vi "myRIO_BRig_RT_v0,31.vi"() -> ()   [LabVIEW 2014]
uses:
  <vilib>/Platform/TimedLoop/XDataNode/XDataNode.xnode
  <vilib>/Platform/TimedLoop/XDataNode/nitl_modes.ctl
  <vilib>/Platform/TimedLoop/XDataNode/XDNodeRunTimeDep.lvlib
  <vilib>/Platform/TimedLoop/XDataNode/wakeup.ctl
  <vilib>/Platform/TimedLoop/XDataNode/timing_clust.ctl
  <vilib>/rvi/interface/nirviReadWriteControl/nirviReadWriteControl.xnode
  <vilib>/rvi/interface/Simulation/niFpgaSimulationCallBeginRW.vi
  <vilib>/rvi/errors/niLvFpgaAdjustHostInterfaceError.vi
  <vilib>/rvi/interface/nirviCloseFPGA/nirviCloseFPGA.xnode
  <vilib>/myRIO/Instrument Drivers/Utilities/Utilities.lvlib
  <vilib>/rvi/interface/nirviOpenFPGA/nirviOpenFPGA.xnode
  myRIO_BRig_RT__Case_Exp_stateList.ctl
  <vilib>/WebDAVClient/Advanced/SessionHandle.ctl
  <vilib>/WebDAVClient/NI_WebDAV.lvlib
  myRIO_BRig_RT__Case_NonExp_stateList.ctl
  NiFpgaLv.dll
  <vilib>/Utility/error.llb/Error Cluster From Error Code.vi
  <vilib>/FPGAPlugInAG/Dynamic/niLvFpga_Close_Dynamic.vi
  myRIO_BRig_FPGA_v2,5__PortC__build.lvbitx
  myRIO_BRig_FPGA_v2,5__PortC.vi
  <vilib>/FPGAPlugInAG/myRIO-1900/niLvFpga_Open_myRIO-1900.vi
  <vilib>/rvi/interface/common/dynamic/niFpgaDynamicAddResources.vi
panel:
  in  "LC_Cue1_delayOpt":bool
  in  "LC_ENL1_delayOpt":bool
  in  "Tcycle_Cue_max":u16=1000 caption="Max [ms]" min=5 max=5000 step=5
  in  "Tcycle_Cue_min":u16=1000 caption="Min [ms]" min=5 max=5000 step=5
  in  "SendData":bool
  out "cSpout":enum16{"Left", "Right"}(ring) caption="Left or Right Spout"
  out "A4":u32 caption="LickCounter_Right"
  out "A2":u32 caption="LickCounter_Left"
  in  "tDelay_laser_wro":u32
  in  "tCycle_laser_wro":u32=1000
  in  "tDelay_laser_rew":u32
  in  "laserResponse_wrong_LED":bool
  out "error_initTrial":errorcluster
  out "error_Selection_pre":errorcluster
  out "error_Selection":errorcluster
  in  "tCycle_laser_rew":u32=1000
  out "SelectWrong":bool
  out "SelectReward":bool
  in  "Left(F)_or_Right(T)":bool
  in  "ignoreWrong":bool
  in  "SelectionState":bool
  in  "laserResponse_wrong":bool
  in  "laserResponse_reward":bool
  in  "laserResponse_reward_LED":bool
  out "nRewards_Right":u16 caption="# Rewards Total (Right)"
  out "nRewards_Left":u16 caption="# Rewards Total (Left)"
  out "nRewards_cur":u16 caption="# Rewards in Current Block"
  out "TpB_target":u16 caption="Target Trials Per Block"
  out "cState_NonExp":T1 caption="NonExperimental State"
  out "iBlock":u16 caption="Current Block"
  out "cState":T2 caption="Experimental State"
  out "iTrial":u16 caption="Current Trial"
  in  "warmupType":bool
  in  "TestConnection":bool
  in  "warmup":bool caption="WarmUp"
  in  "Host Filename Prefix":string="Exp1_TM2"
  out "Connected To Host?":bool
  in  "Host Password":string="sabalab"
  in  "Host UserName":string="Test2"
  in  "sp_RightSpout":u16(slide)=2 max=2 step=1 scale=0.0..2.0
  in  "sp_LeftSpout":u16(slide)=2 max=2 step=1 scale=0.0..2.0
  in  "BUR_max":u16 caption="Count Reward Structure  (0 = off)"
  in  "LC_Wrong_Probability":u16
  in  "LC_Wrong_Trial":u16(slide) max=2 step=1 scale=0.0..2.0
  in  "LC_Wrong_Block":u16(slide) max=2 step=1 scale=0.0..2.0
  in  "LC_Wrong_OnOff":bool
  in  "LC_Reward_Probability":u16
  in  "LC_Reward_Trial":u16(slide) max=2 step=1 scale=0.0..2.0
  in  "LC_Reward_Block":u16(slide) max=2 step=1 scale=0.0..2.0
  in  "LC_Reward_OnOff":bool
  in  "LC_Cue2_Probability":u16
  in  "LC_Cue2_Trial":u16(slide) max=2 step=1 scale=0.0..1.0
  in  "LC_Cue2_Block":u16(slide) max=2 step=1 scale=0.0..2.0
  in  "LC_Cue2_OnOff":bool
  in  "LC_Cue1_Probability":u16
  in  "LC_Cue1_Trial":u16(slide) max=2 step=1 scale=0.0..1.0
  in  "LC_Cue1_Block":u16(slide) max=2 step=1 scale=0.0..2.0
  in  "LC_Cue1_OnOff":bool
  in  "LC_ENL2_Probability":u16
  in  "LC_ENL2_Trial":u16(slide) max=2 step=1 scale=0.0..1.0
  in  "LC_ENL2_Block":u16(slide) max=2 step=1 scale=0.0..2.0
  in  "LC_ENL2_OnOff":bool
  in  "LC_ENL1_Probability":u16
  in  "LC_ENL1_Trial":u16(slide) max=2 step=1 scale=0.0..1.0
  in  "LC_ENL1_Block":u16(slide) max=2 step=1 scale=0.0..2.0
  in  "A6":bool caption="Activate Recording?\n(Select Prior to\nStarting Experiment)"
  in  "Tcycle_Timeout":u16=1000 caption="Timeout Time [ms]" min=10 max=10000 step=1
  in  "Tcycle_Wrong":u16=1000 caption="Wrong Time [ms]" min=10 max=10000 step=1
  in  "Tcycle_Selection":u16=1000 caption="Answer Time [ms]" min=1 max=10000 step=1
  in  "Tcycle_RewardPost":u16=1000 caption="Consumption Time [ms]" min=250 max=10000 step=250
  in  "Tcycle_Reward_L":u16=500 caption="Reward Time [ms]" min=1 max=1000 step=1
  in  "Tcycle_Reward_R":u16=500 caption="Reward Time [ms]" min=1 max=1000 step=1
  in  "TpB_Max_R":u16=4 caption="Max TrialsPerBlock" min=1 max=12 step=1
  in  "TpB_Min_R":u16=4 caption="Min TrialsPerBlock" min=1 max=12 step=1
  in  "TpB_Max_L":u16=4 caption="Max TrialsPerBlock" min=1 max=12 step=1
  in  "TpB_Min_L":u16=4 caption="Min TrialsPerBlock" min=1 max=12 step=1
  in  "BUR_min":u16 caption="Count Reward Structure  (0 = off)"
  in  "TrialUntilReward":bool caption="Ignore Wrong \nSelection"
  in  "CueCycles":u16=1 caption="Cue Structure" min=1 max=1 step=1
  in  "MTrig_Laser_Tcycle":u16=10 caption="Time [ms]"
  in  "MTrig_Laser_trig":bool
  in  "MTrig_Audio_trig__R":bool caption="Trigger Audio"
  in  "MTrig_Audio_trig__L":bool caption="Trigger Audio"
  in  "RewCalib_Trig_R":bool caption="Calibrate_R"
  in  "RewCalib_Trig_L":bool caption="Calibrate_L"
  in  "MTrig_Solenoid_Tcycle__R":u16=300 caption="Time [ms]"
  in  "MTrig_Solenoid_Tcycle__L":u16=300 caption="Time [ms]"
  in  "MTrig_Solenoid_trig__R":bool caption="Solenoid"
  in  "MTrig_Solenoid_trig__L":bool caption="Solenoid"
  in  "STOP_abort":bool caption="Stop LabView\n(Stops myRio and FPGA)"
  in  "STOP_endBlock":bool caption="Stop Experiment\n@ End of Block"
  in  "STOP_endTrial":bool caption="Stop Experiment\n@ End of Trial"
  in  "START":bool caption="Start Experiment"
  in  "Tcycle_CuePenalty":u16=1000 caption="Penalty [ms]" min=1 max=10000 step=1
  in  "Audio_Amp__R":u16=100 caption="Amp"
  in  "Audio_Freq__R":u16=5 caption="Freq [kHz]" max=14 step=1
  in  "Audio_Amp__L":u16=100 caption="Amp"
  in  "Audio_Freq__L":u16=5 caption="Freq [kHz]" max=14 step=1
  in  "LC_Wrong_Tdelay":u16
  in  "LC_Cue2_Tdelay":u16
  in  "LC_ENL2_Tdelay":u16
  in  "LC_Reward_Tdelay":u16
  in  "LC_Cue1_Tdelay":u16
  in  "LC_ENL1_Tdelay":u16
  in  "LC_ENL1_OnOff":bool
  in  "Tcycle_ENLPenalty":u16=100 caption="Penalty [ms]" min=10 max=100 step=10
  in  "Tcycle_ENL_max":u16=1000 caption="Max [ms]" min=250 max=10000 step=250
  in  "Tcycle_ENL_min":u16=1000 caption="Min [ms]" min=250 max=10000 step=250
  # "Manual Control"
  # "Task Structure"
  # "Task Timing"
  # "Laser Control    [10ms pulse]\n\n                              On/Off      Block          Trial    Probability [%]   Delay [ms]"
  # "Manual Solenoid Trigger\nLeft              Right"
  # "Master Structure"
  # "Enforced NonLick"
  # "Enforced NonLick 1"
  # "from end"
  # "Time = Cue Min"
  # "Min\n \n  \nMax"
  # "from start"
  # "(1) = Switching\n(2) = Two Choice"
  # "Enforced NonLick 2"
  # "Cue"
  # "Cue 1"
  # "from end"
  # "from start"
  # "Cue then reward"
  # "Min"
  # "Max"
  # "Cue 2"
  # "Cue with reward"
  # "Trial Per Block Structure\n       Left                    Right"
  # "Spout Selection Control"
  # "Manual Speaker Trigger\nLeft              Right"
  # "Selection Reward"
  # "Answer Time\n         [ms]\n\n  \nWrong Choice Penalty\n         [ms]\n \n \nChoice Timeout Penalty\n         [ms]"
  # "Selection Wrong"
  # "Cue Control"
  # "Left              Right"
  # "State"
  # "Manual Laser Trigger"
  # "Freq [kHz]\n \n \nAmp\n \n\n \n\nSpeaker\nSetting"
  # "Reward Control\n                 Left              Right"
  # "Min = 1\nMax = 32k"
  # "Reward Time\n         [ms]"
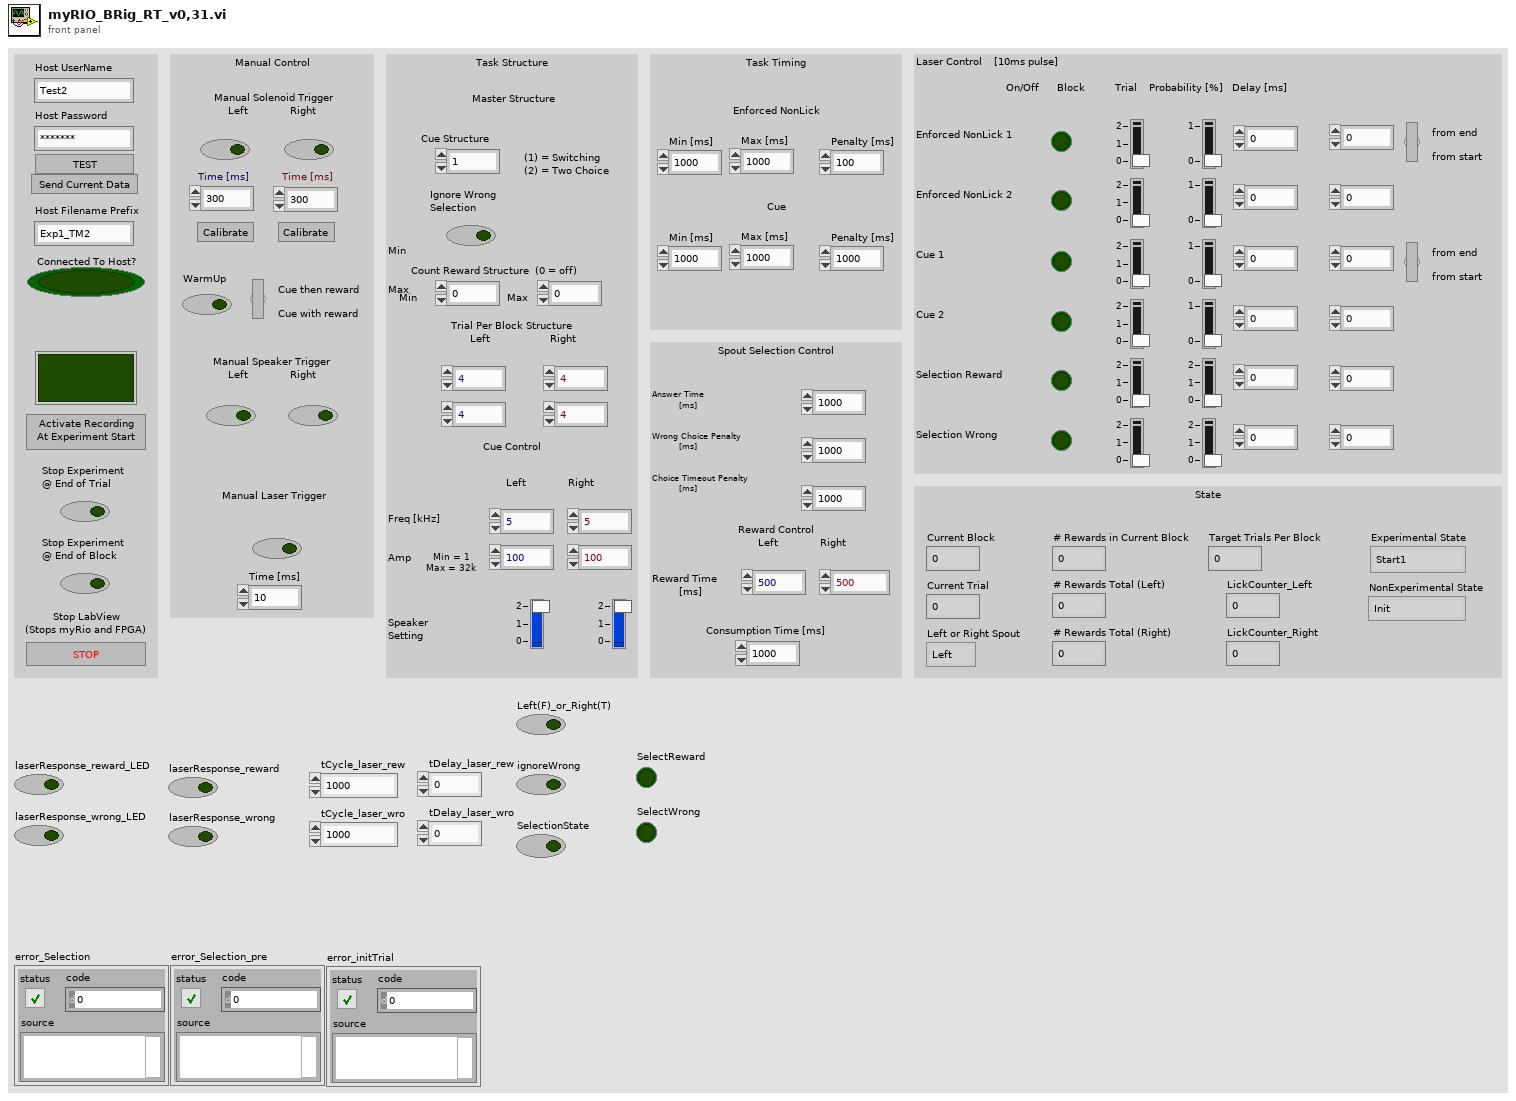
[diagram p1: front panel]
types:
  T1 = typedef "myRIO_BRig_RT__Case_NonExp_stateList.ctl" = enum16{"Init", "UploadSettings_pre", "UploadSettings_Read_dataExp", "UploadSettings_dataExp_1", "UploadSettings_Read_dataLC", "UploadSettings_dataLC_1", "UploadSettings_dataLC_2", "UploadSettings_Read_dataMTrig", "UploadSettings_dataMTrig_1", "UploadSettings_post", "Idle_pre", "IdleEmpty", "IdleEmpty2", "IdleEmpty3", "IdleEmpty4", "Idle", "Idle_2", "Idle_3", "Idle_4", "Idle_post", "Cue_pre__pre", "Cue_pre", "Cue", "Cue_post", "RewardCalibration_pre", "DispenseWater_pre__pre", "DispenseWater_pre", "DispenseWater", "DispenseWater_post", "TestConnection", "SendData", "End"}
  T2 = typedef "myRIO_BRig_RT__Case_Exp_stateList.ctl" = enum16{"Start1", "Start2", "Start3", "saveSettings1", "saveSettings2", "saveSettings3", "saveSettings4_LC_ENL", "saveSettings5_LC_Cue", "saveSettings6_LC_Other", "setSettings_Audio", "setSettings_Laser", "initBlock_pre", "initBlock", "initBlock2", "initBlock_post", "initTrial_pre", "initTrial", "initTrial2", "initTrial3", "initTrial4", "initTrial_LC_ENL1", "initTrial_LC_Cue1", "initTrial_post", "ENL1_pre", "ENL1", "ENL1_post", "ENL1Penalty_pre", "ENL1Penalty", "ENL2_pre", "ENL2", "ENL2Penalty_pre", "ENL2Penalty", "Cue1_pre", "Cue1", "Cue1_post", "Cue1Penalty_pre", "Cue1Penalty", "Cue2_pre", "Cue2", "Cue2Penalty_pre", "Cue2Penalty", "Selection_pre", "Selection", "Select_post", "SelectReward_pre", "SelectReward", "SelectRewardPost_pre", "SelectRewardPost", "SelectWrong_pre", "SelectWrong", "SelectWrong_post", "SelectTimeout_pre", "SelectTimeout", "SelectTimeout_post", "endTrial_pre", "endTrial1", "endTrial2", "endTrial3", "endTrial_post", "endBlock_pre", "endBlock", "endBlock_post", "endExp", "commConnect", "commUpload_pre", "commUpload_dataBlock", "commUpload_dataCurrent", "commUpload_dataExp", "commUpload_dataLC", "commUpload_dataTrial", "commUpload_post", "saveData_pre", "saveData_dataBlock", "saveData_dataCurrent", "saveData_dataExp", "saveData_dataLC", "saveData_dataTrial", "saveData_post"}
  T3 = typedef "XDNodeRunTimeDep.lvlib/timing_clust.ctl" = cluster{"Expected End [f-1]":u64, "Actual End [f-1]":u64, "Finished Late? [f-1]":bool, "Expected End [i-1]":u64, "Actual End [i-1]":u64, "Finished Late? [i-1]":bool, "Expected Start [i]":u64, "Actual Start [i]":u64, "Expected Start [f]":u64, "Actual Start [f]":u64, "Source Name":string, "Structure Name":string, "Period":i64, "Deadline":i64, "Offset":i64, "Start":i64, "Priority":i32, "Timeout":i32, "Mode":T4, "Wakeup Reason":T5, "Error":errorcluster, "Source Type":string, "Secondary Source Type":string, "Global End Time":u64, "Global Start Time":u64, "Frame Duration":u64, "Iteration Duration":u64, "Assigned CPU":i32, "I/O Scan Engine Mode":u32}
  T4 = typedef "XDNodeRunTimeDep.lvlib/nitl_modes.ctl" = enum32{"No Change", "Process missed periods, maintain original phase", "Discard missed periods, maintain original phase", "Process missed periods, ignore original phase", "Discard missed periods, ignore original phase"}
  T5 = typedef "XDNodeRunTimeDep.lvlib/wakeup.ctl" = enum32{"Normal", "Aborted", "Asynchronous wakeup", "Timing source error", "Timed loop error", "Timeout"}
  T6 = typedef "NI_WebDAV.lvlib/SessionHandle.ctl" = refnum<k1>
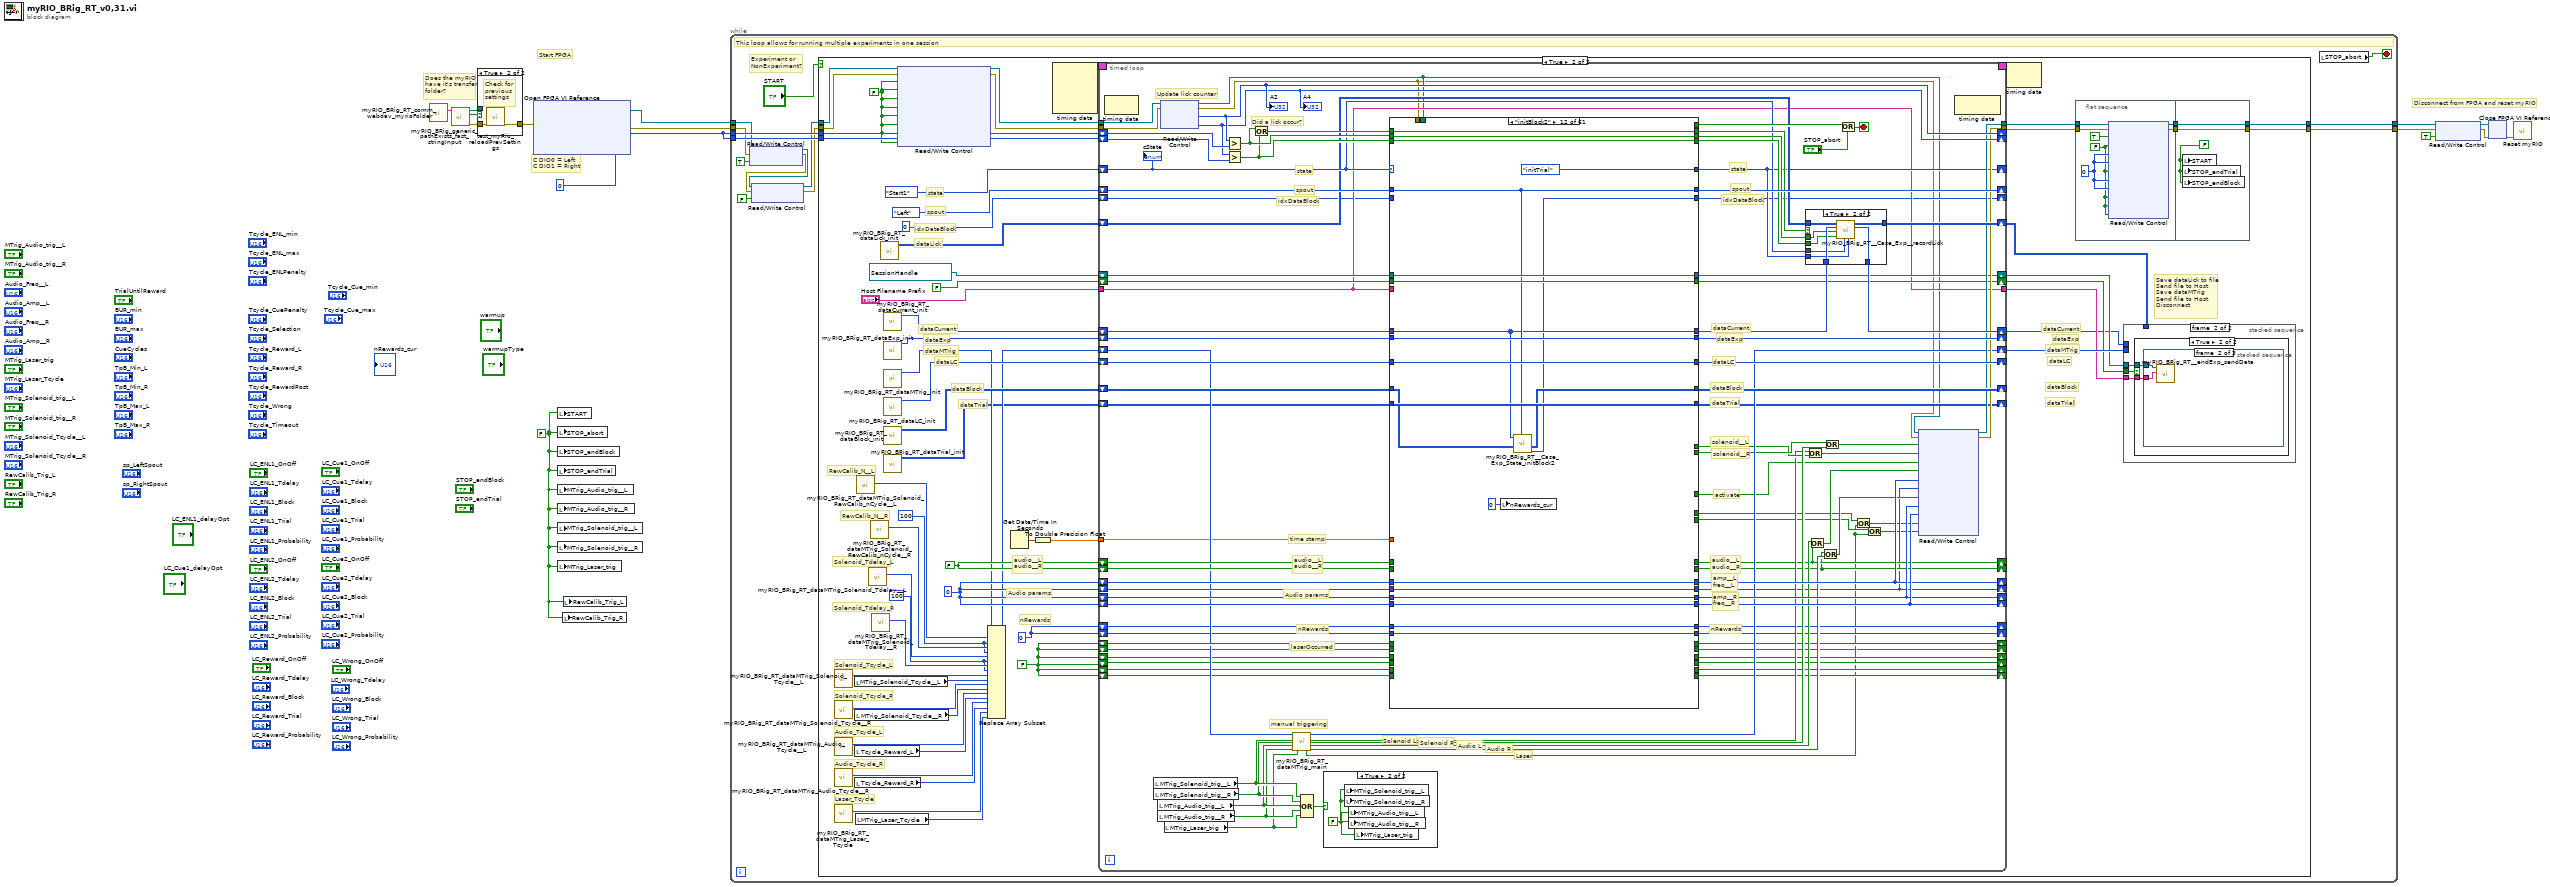
[diagram p0: block diagram]
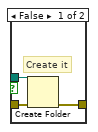
[diagram p2: hidden frame]
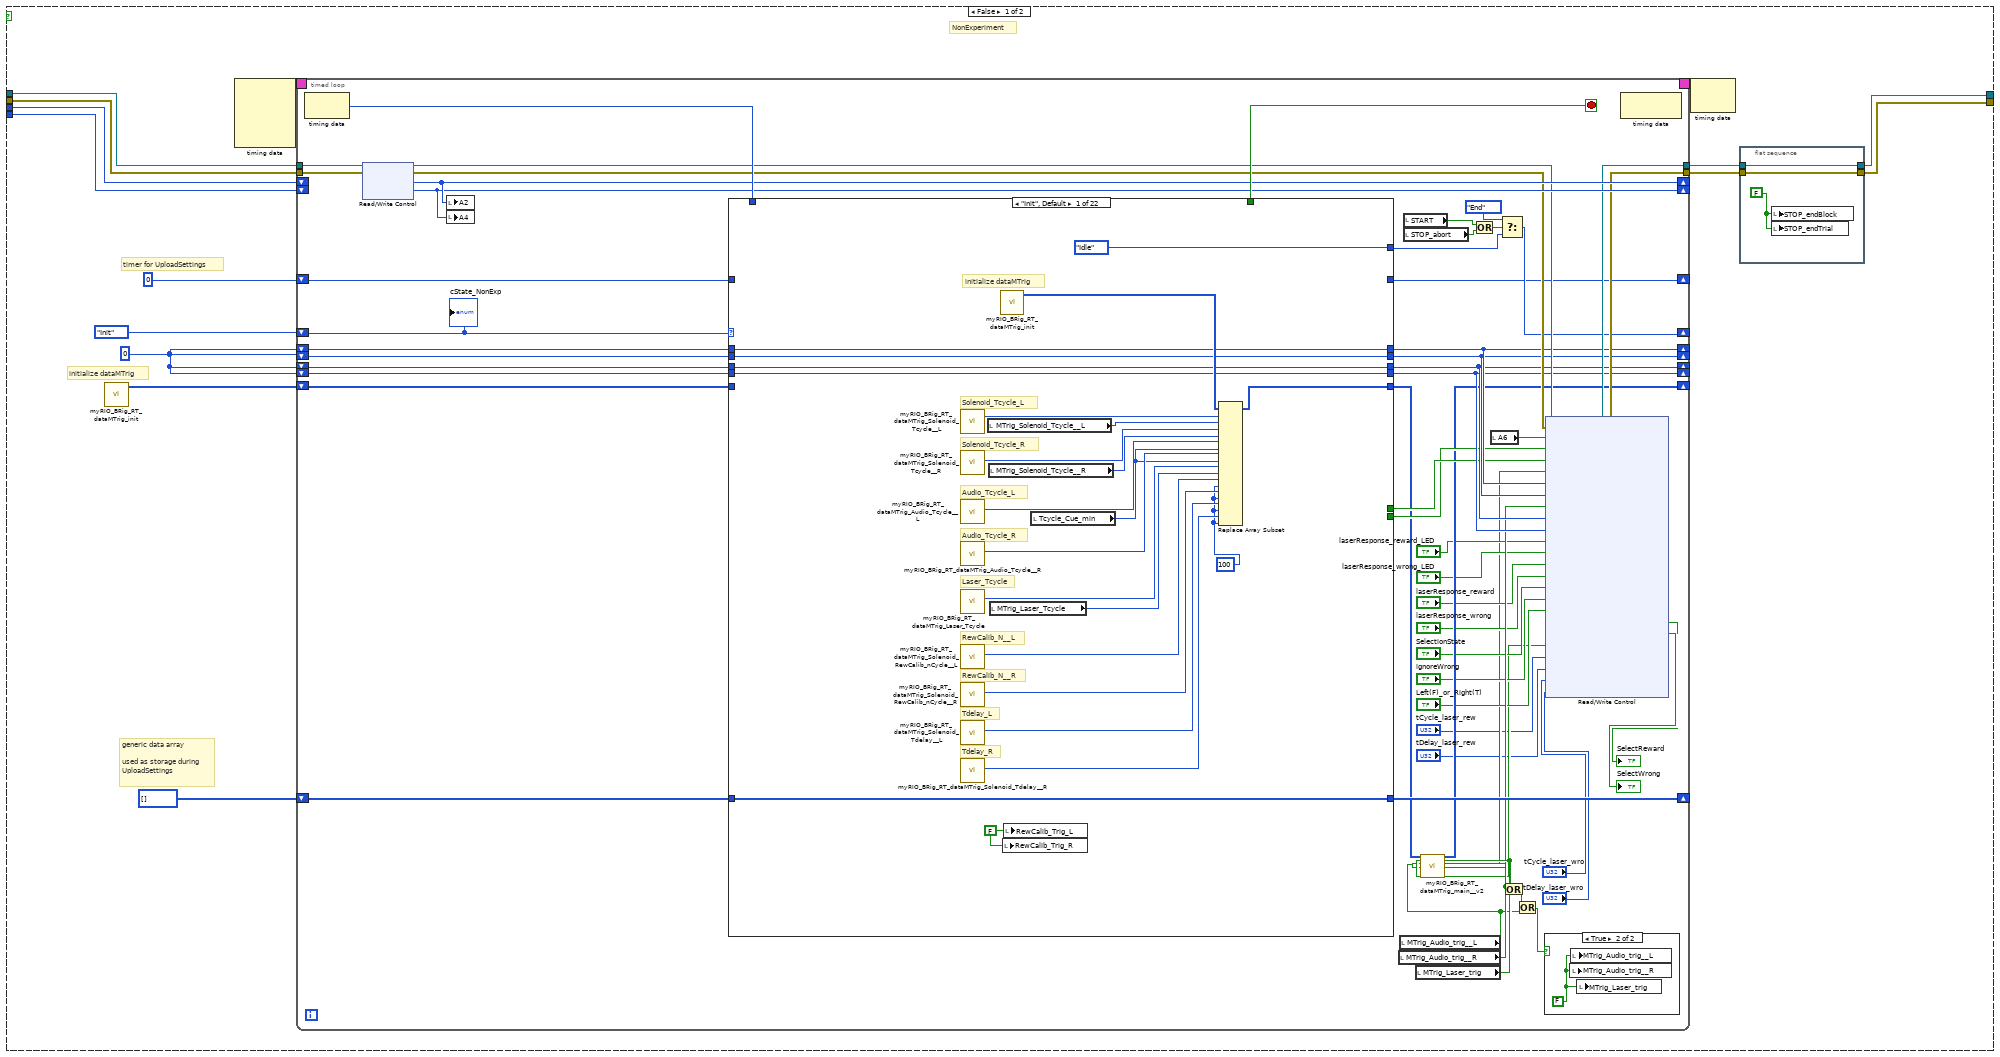
[diagram p3: hidden frame]
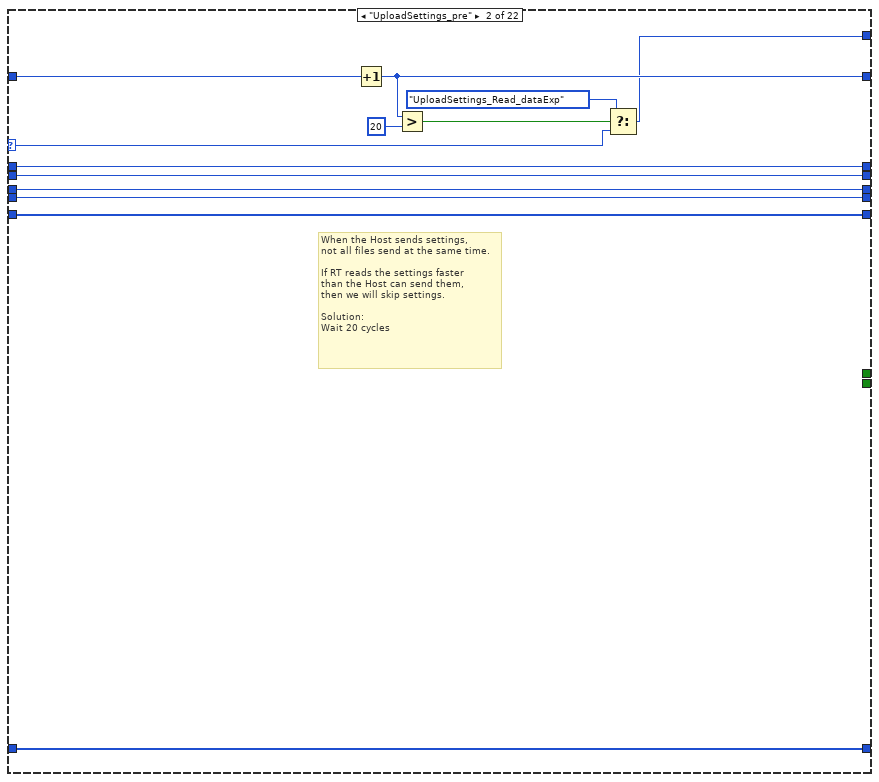
[diagram p5: hidden frame]
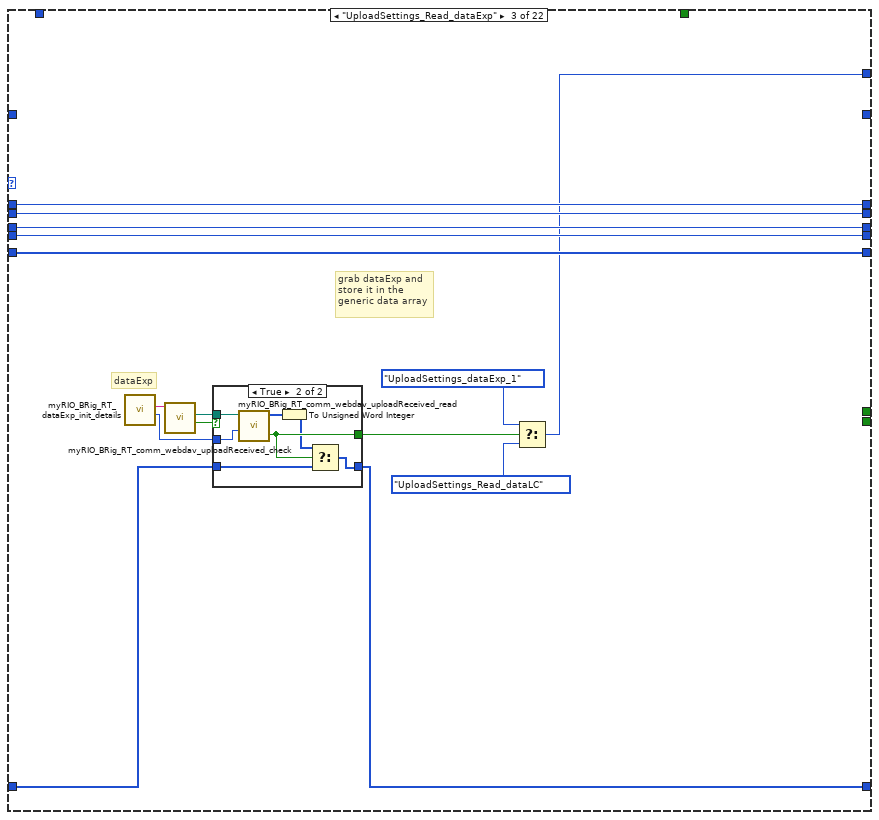
[diagram p6: hidden frame]
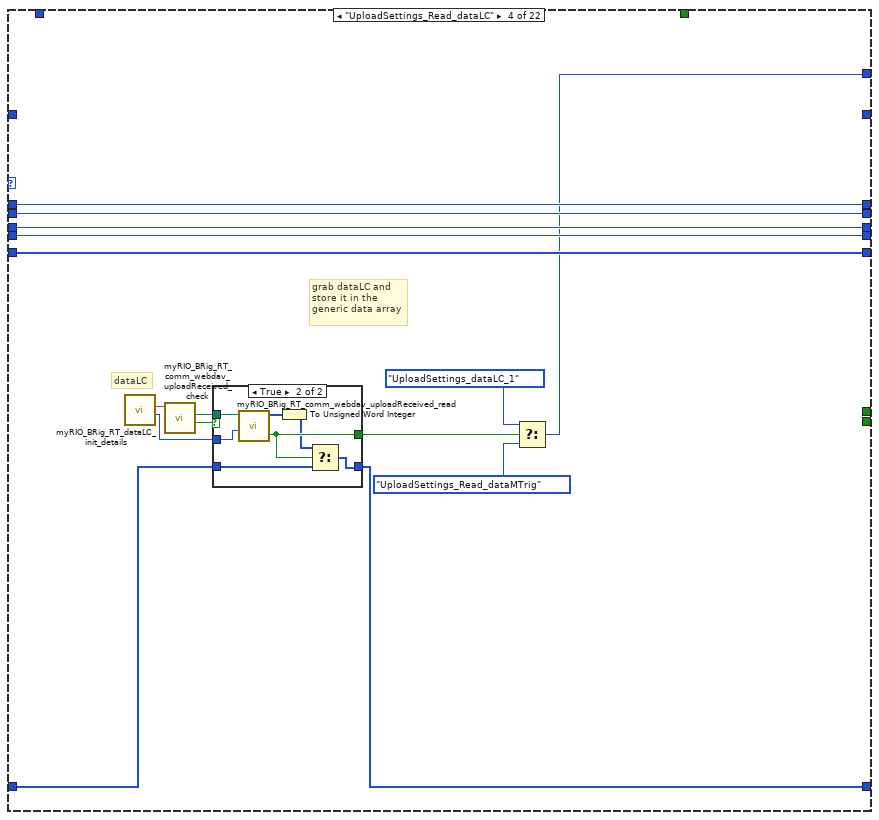
[diagram p8: hidden frame]
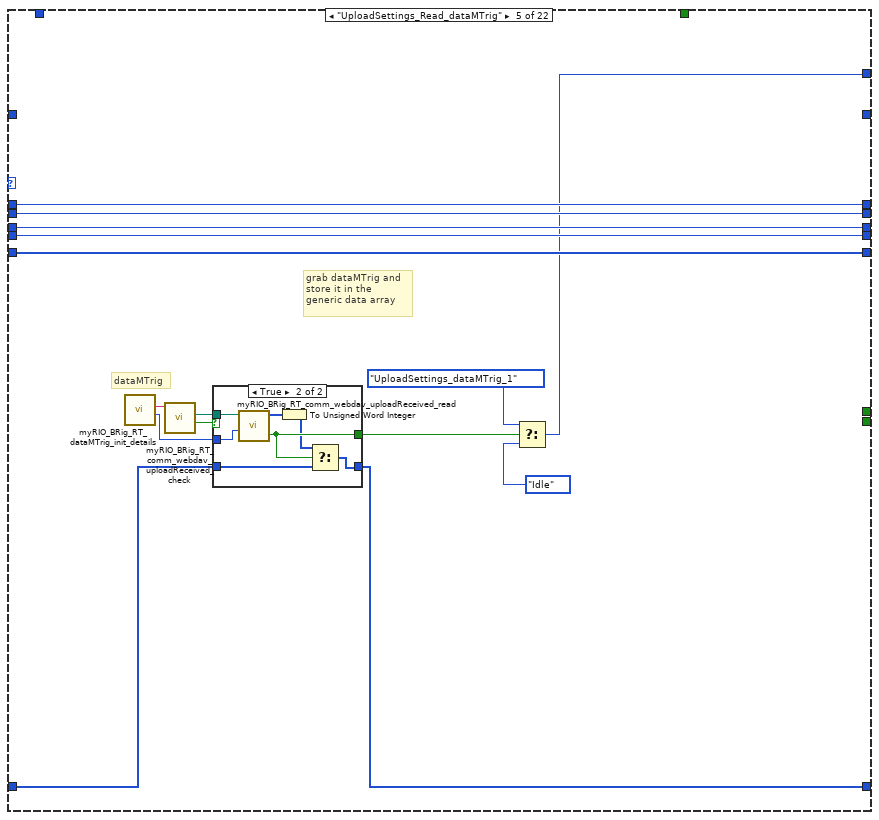
[diagram p10: hidden frame]
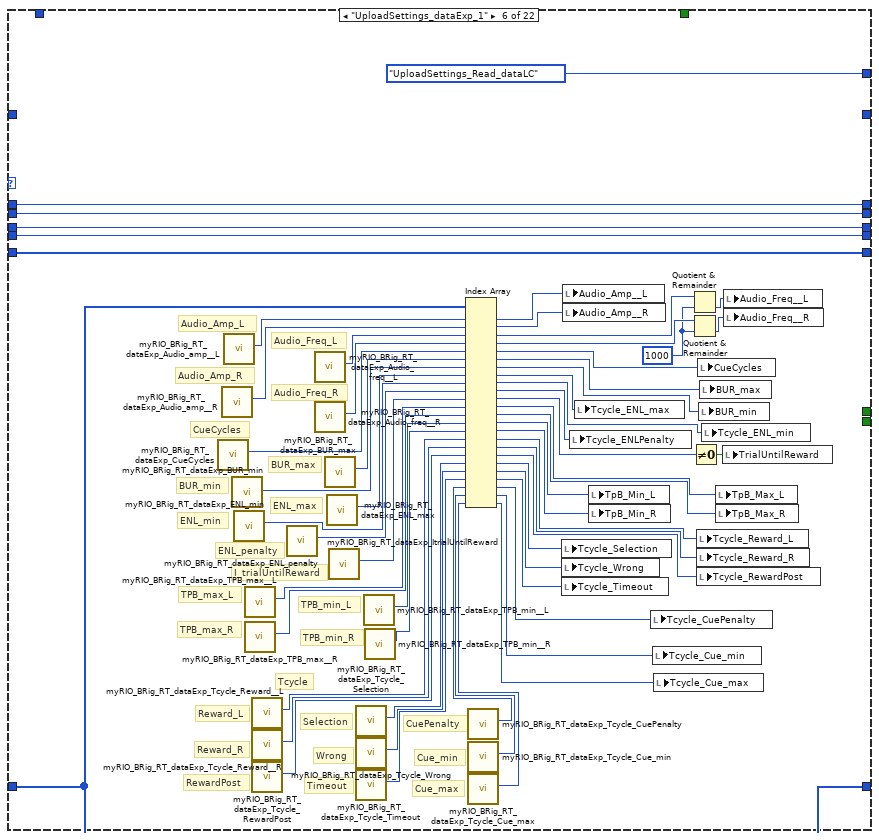
[diagram p12: hidden frame]
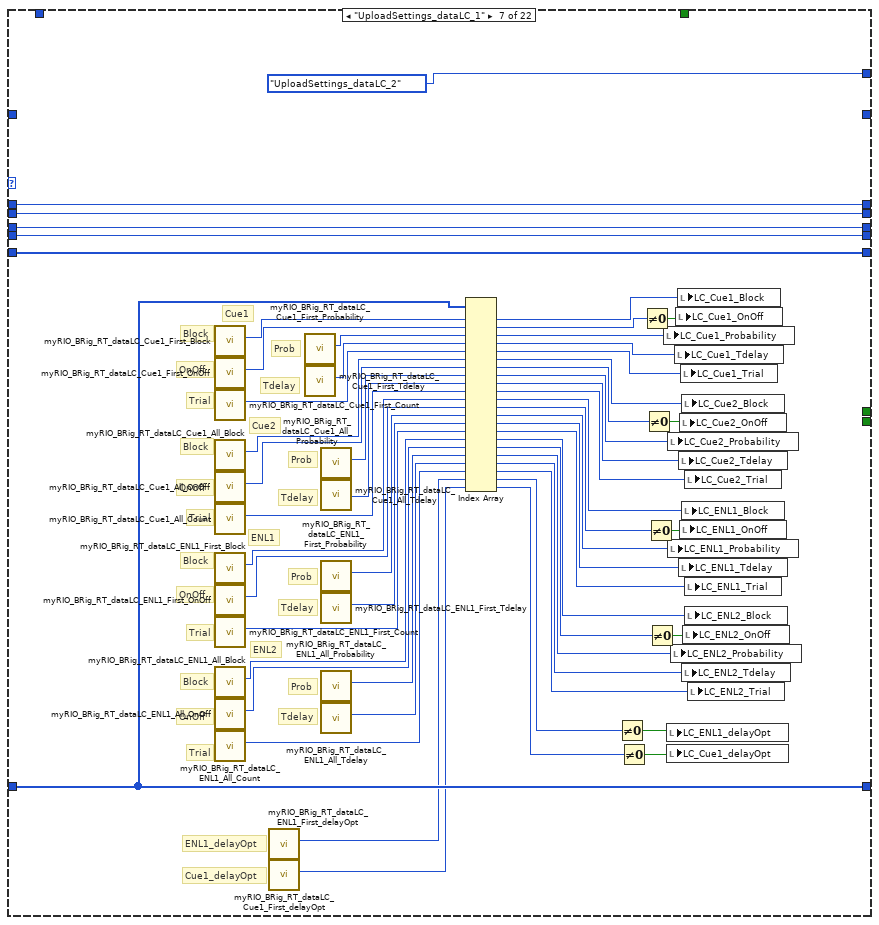
[diagram p13: hidden frame]
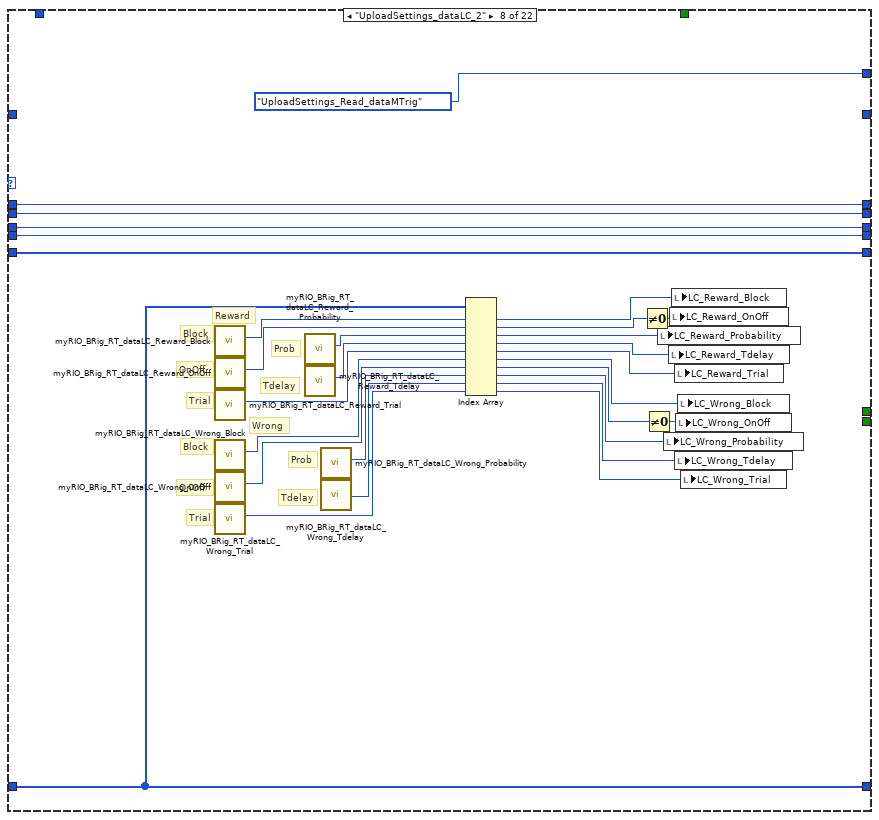
[diagram p14: hidden frame]
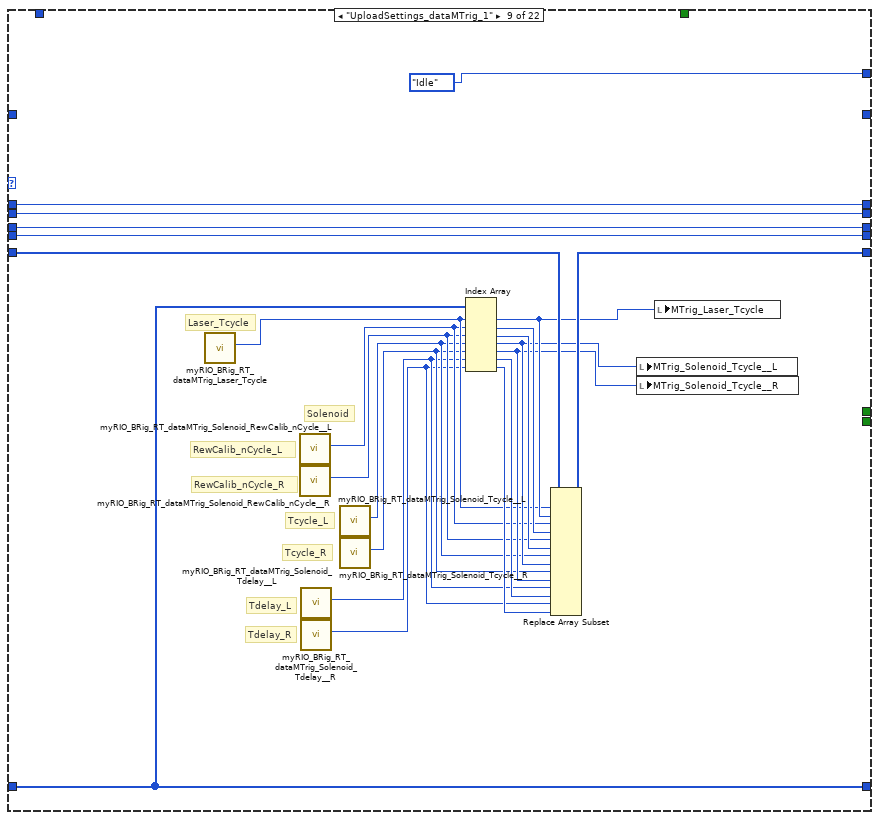
[diagram p15: hidden frame]
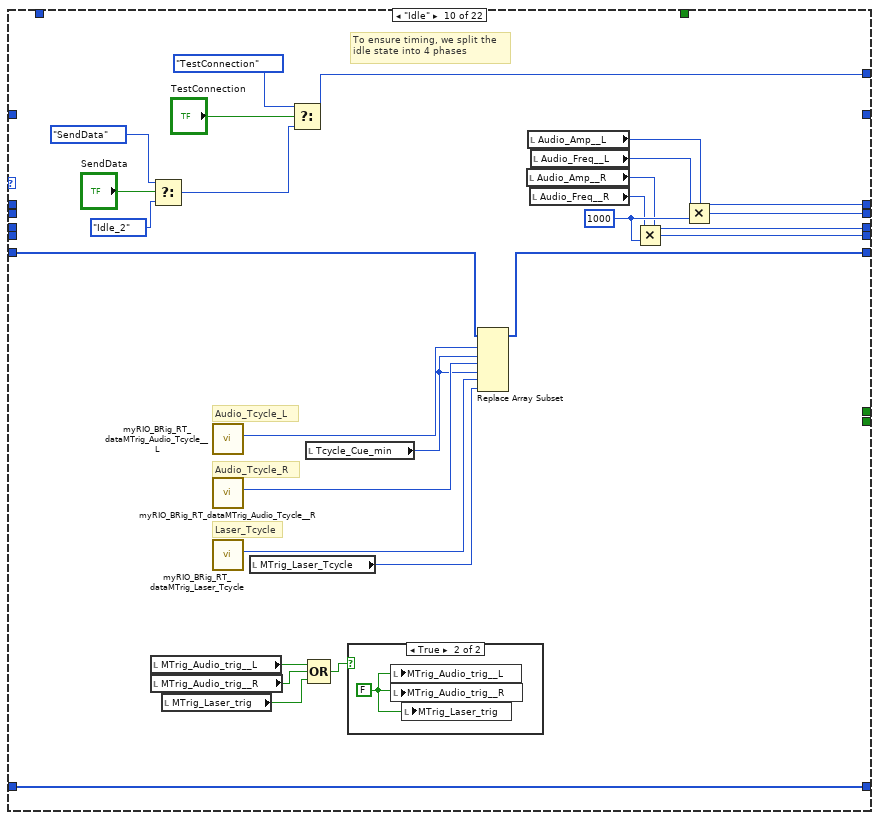
[diagram p16: hidden frame]
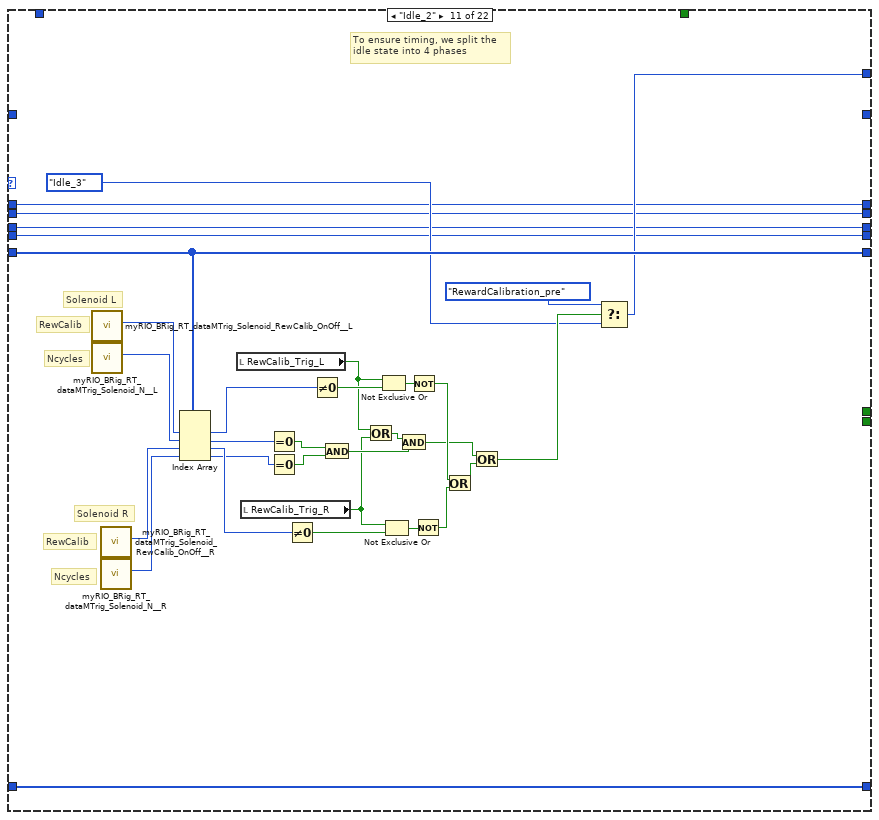
[diagram p18: hidden frame]
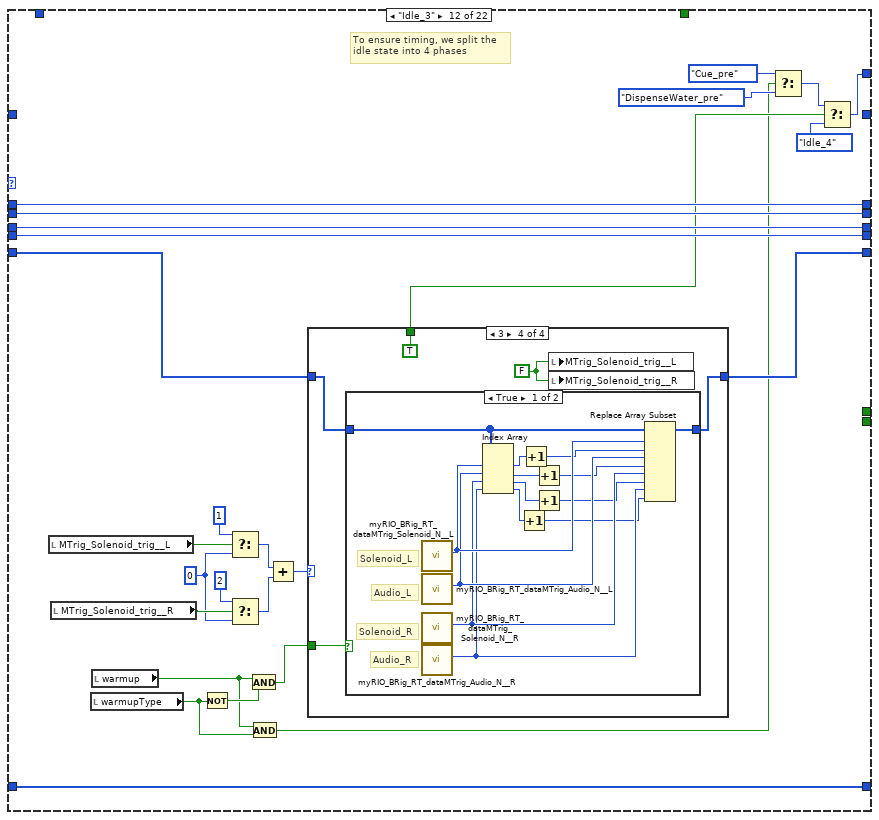
[diagram p19: hidden frame]
diagram:
  w9 = u32 0
  w6 = FALSE
  # "Does the myRIO\nhave it's transfer\nfolder?"
  # "C DIO0 = Left\nC DIO1 = Right"
  # "Start FPGA"
  # "Disconnect from FPGA and reset myRIO"
  n1 = call "myRIO_BRig_RT_comm_webdav_myrioFolder.vi"() -> ("output_myrioFolder"=w4:string)  [unwired: 11 in]
  n2 = call "myRIO_BRig_generic_pathExists_fast_stringInput.vi"("input_filePath"=w4) -> ("output_error"=w3:errorcluster, "output_Iexist"=w2:bool, "output_filePath"=w1:path)  [unwired: 8 in]
  n3 = case shown="True" w2 {
    tunnel: w1 -> [w18 _]
    tunnel: w3 -> [w17 w20]
    tunnel: [w16 w19] -> w5
    frame False {
      # "Create it"
      n4 = Create Folder(path (use dialog)=w18, error in=w17) -> (error out=w16:errorcluster)  [unwired: 1 in, 2 out]
    }
    frame True {
      # "Check for\nprevious\nsettings"
      n5 = call "test_myRio_reloadPrevSettings.vi"("input_error"=w20) -> ("output_error"=w19:errorcluster)  [unwired: 10 in]
    }
  }
  n6 = xnode "Open FPGA VI Reference"("error in"=w5) -> ("FPGA VI Reference Out"=w11:refnum<k20>, "error out"=w10:errorcluster)  [unwired: 1 in]
  n7 = local write "START"(w6) -> ()
  n8 = local write "STOP_abort"(w6) -> ()
  n9 = local write "STOP_endBlock"(w6) -> ()
  n10 = local write "STOP_endTrial"(w6) -> ()
  n11 = local write "MTrig_Audio_trig__L"(w6) -> ()
  n12 = local write "MTrig_Audio_trig__R"(w6) -> ()
  n13 = local write "MTrig_Solenoid_trig__L"(w6) -> ()
  n14 = local write "MTrig_Solenoid_trig__R"(w6) -> ()
  n15 = local write "MTrig_Laser_trig"(w6) -> ()
  n16 = local write "RewCalib_Trig_R"(w6) -> ()
  n17 = local write "RewCalib_Trig_L"(w6) -> ()
  n18 = while {
    tunnel: w11 -> [w24]
    tunnel: w10 -> [w29]
    tunnel: w9 -> [w32]
    tunnel: w9 -> [w31]
    tunnel: [w22] -> w8
    tunnel: [w21] -> w7
    stop <- w30 stop-if-true
    # "Experiment or\nNonExperiment?"
    # "This loop allows for running multiple experiments in one session"
    n19 = xnode "Read/Write Control"("FPGA VI Reference In"=w24, "error in"=w29, "Counts_Reset"=TRUE) -> ("FPGA VI Reference Out"=w26:refnum<k20>, "error out"=w27:errorcluster)
    n20 = xnode "Read/Write Control"("FPGA VI Reference In"=w26, "error in"=w27, "Counts_Reset"=FALSE) -> ("FPGA VI Reference Out"=w23:refnum<k20>, "error out"=w25:errorcluster)
    n21 = case shown="True" "START" {
      tunnel: w32 -> [w45 w908]
      tunnel: w31 -> [w44 w907]
      tunnel: w25 -> [w42 w858]
      tunnel: w23 -> [w43 w857]
      tunnel: [w40 w904] -> w22
      tunnel: [w38 w899] -> w21
      frame False {
        w37 = u16 0 ("Audio_Amp__L")
        # "generic data array\n\nused as storage during\nUploadSettings"
        # "timer for UploadSettings"
        # "initialize dataMTrig"
        # "NonExperiment"
        n22 = call "myRIO_BRig_RT_dataMTrig_init.vi"() -> ("output_dataMTrig"=w46:u16[])  [unwired: 5 in]
        n23 = node-c288() -> (w49:T3)  [unwired: 4 in]
        n24 = timed-loop {
          timing: w49 -> [_]
          timing-out: [_] -> w48
          shift-right: [w83] -> _
          shift-left: w46 -> [w107]
          shift-right: [w72] -> _
          shift-left: myRIO_BRig_RT__Case_NonExp_stateList."Init" ("Enum") -> [w97]
          shift-right: [w105] -> _
          shift-left: w45 -> [_]
          shift-right: [w104] -> _
          shift-left: w44 -> [_]
          tunnel: [w100] -> w41
          tunnel: [w98] -> w39
          tunnel: w42 -> [w103]
          tunnel: w43 -> [w102]
          shift-right: [w96] -> _
          shift-left: u16[] [] ("output_data") -> [w95]
          shift-right: [w90] -> _
          shift-left: w37 -> [w94]
          shift-right: [w89] -> _
          shift-left: w37 -> [w93]
          shift-right: [w88] -> _
          shift-left: w37 -> [w92]
          shift-right: [w87] -> _
          shift-left: w37 -> [w91]
          shift-right: [w54] -> _
          shift-left: u16 0 ("Audio_Amp__L") -> [w55]
          stop <- w108 stop-if-true
          n25 = node-c288() -> (w106:i64)  [unwired: 1 in]
          n26 = xnode "Read/Write Control"("FPGA VI Reference In"=w102, "error in"=w103) -> ("FPGA VI Reference Out"=w101:refnum<k20>, "error out"=w99:errorcluster, "A2_LickL"=w105:u32, "A4_LickR"=w104:u32)
          n27 = local write "A2"(w105) -> ()
          n28 = local write "A4"(w104) -> ()
          n29 = case shown="\"Init\", Default" w97 {
            selector: w97 -> [_ w141 _ _ _ _ _ _ _ _ _ _ _ _ w567 _ _ w752 _ _ _ w849]
            tunnel: [myRIO_BRig_RT__Case_NonExp_stateList."Idle" ("Enum") w139 w146 w169 w192 myRIO_BRig_RT__Case_NonExp_stateList."UploadSettings_Read_dataLC" ("Enum") myRIO_BRig_RT__Case_NonExp_stateList."UploadSettings_dataLC_2" ("Enum") myRIO_BRig_RT__Case_NonExp_stateList."UploadSettings_Read_dataMTrig" ("f") myRIO_BRig_RT__Case_NonExp_stateList."Idle" ("Enum") w393 w414 w447 w538 myRIO_BRig_RT__Case_NonExp_stateList."Cue" ("t") w566 myRIO_BRig_RT__Case_NonExp_stateList."DispenseWater_pre" ("Enum") w694 w750 w777 myRIO_BRig_RT__Case_NonExp_stateList."Idle" ("Enum") myRIO_BRig_RT__Case_NonExp_stateList."Idle" ("Enum") w849] -> w73
            tunnel: [w124 w134 w156 w179 w202 w273 w330 w359 w379 w404 w429 w458 w536 w554 w580 w604 w731 w757 w788 w831 w841 w847] -> w84
            tunnel: [_ _ _ _ _ _ _ _ _ _ _ _ _ _ _ _ _ _ _ _ _ TRUE] -> w108
            tunnel: w107 -> [_ w134 w156 w179 w202 w273 w330 w359 w380 w403 w429 w459 w536 w555 w580 w590 w727 w758 w789 w831 w841 w847]
            tunnel: w106 -> [_ _ _ _ _ _ _ _ _ _ _ _ _ _ _ _ _ w762 _ _ _ _]
            tunnel: [w113 w133 w147 w170 w193 w217 w280 w331 w360 w388 w409 w441 w531 w542 w565 w581 w679 w735 w770 w819 w835 w842] -> w96
            tunnel: w95 -> [w113 w133 w148 w171 w194 w217 w280 w331 w360 w388 w409 w441 w531 w542 w565 w581 w679 w735 w770 w819 w835 w842]
            tunnel: [w117 w137 w159 w182 w205 w270 w328 w334 w377 w399 w412 w451 w533 w562 w577 w584 w733 w768 w795 w822 w838 w845] -> w89
            tunnel: [w115 w135 w157 w180 w203 w268 w326 w332 w375 w398 w410 w453 w535 w560 w579 w582 w732 w766 w793 w820 w836 w843] -> w87
            tunnel: [w118 w138 w160 w183 w206 w271 w329 w335 w378 w397 w413 w450 w532 w564 w576 w585 w734 w769 w796 w823 w839 w846] -> w90
            tunnel: [w116 w136 w158 w181 w204 w269 w327 w333 w376 w396 w411 w452 w534 w561 w578 w583 w732 w767 w794 w821 w837 w844] -> w88
            tunnel: w94 -> [w118 w138 w160 w183 w206 w271 w329 w335 w378 _ w413 w450 w532 w564 w576 w585 w734 w769 w796 w823 w839 w846]
            tunnel: w93 -> [w117 w137 w159 w182 w205 w270 w328 w334 w377 _ w412 w451 w533 w562 w577 w584 w733 w768 w795 w822 w838 w845]
            tunnel: w92 -> [w116 w136 w158 w181 w204 w269 w327 w333 w376 _ w411 w452 w534 w561 w578 w583 w732 w767 w794 w821 w837 w844]
            tunnel: w91 -> [w115 w135 w157 w180 w203 w268 w326 w332 w375 _ w410 w453 w535 w560 w579 w582 _ w766 w793 w820 w836 w843]
            tunnel: [_ _ _ _ _ _ _ _ _ _ _ _ _ _ _ _ _ w759 _ _ _ _] -> w86
            tunnel: [_ _ _ _ _ _ _ _ _ _ _ _ _ _ _ _ _ w741 _ _ _ _] -> w85
            tunnel: w55 -> [_ w145 _ _ _ _ _ _ _ _ _ _ _ _ _ _ _ _ _ _ _ _]
            tunnel: [_ w144 _ _ _ _ _ _ _ _ _ _ _ _ _ _ _ _ _ _ _ _] -> w54
            frame "Init", Default {
              w114 = FALSE ("RewCalib_Trig_L")
              w110 = u16 100 ("new element/subarray")
              # "Tdelay_R"
              # "Tdelay_L"
              # "RewCalib_N__R"
              # "RewCalib_N__L"
              # "Solenoid_Tcycle_R"
              # "Solenoid_Tcycle_L"
              # "Laser_Tcycle"
              # "Audio_Tcycle_R"
              # "Audio_Tcycle_L"
              # "initialize dataMTrig"
              n30 = call "myRIO_BRig_RT_dataMTrig_Solenoid_Tcycle__L.vi"() -> ("output_Solenoid_Tcycle__L"=w126:i32)  [unwired: 11 in]
              n31 = call "myRIO_BRig_RT_dataMTrig_Solenoid_Tcycle__R.vi"() -> ("output_Solenoid_Tcycle__R"=w127:i32)  [unwired: 11 in]
              n32 = call "myRIO_BRig_RT_dataMTrig_Audio_Tcycle__L.vi"() -> ("output_Audio_Tcycle__L"=w128:i32)  [unwired: 11 in]
              n33 = call "myRIO_BRig_RT_dataMTrig_Audio_Tcycle__R.vi"() -> ("output_Audio_Tcycle__R"=w129:i32)  [unwired: 11 in]
              n34 = call "myRIO_BRig_RT_dataMTrig_Laser_Tcycle.vi"() -> ("output_Laser_Tcycle"=w130:i32)  [unwired: 11 in]
              n35 = call "myRIO_BRig_RT_dataMTrig_Solenoid_RewCalib_nCycle__L.vi"() -> ("output_Solenoid_RewCalib_nCycle__L"=w122:i32)  [unwired: 11 in]
              n36 = call "myRIO_BRig_RT_dataMTrig_Solenoid_RewCalib_nCycle__R.vi"() -> ("output_Solenoid_RewCalib_nCycle__R"=w121:i32)  [unwired: 11 in]
              n37 = call "myRIO_BRig_RT_dataMTrig_Solenoid_Tdelay__L.vi"() -> ("output_Solenoid_Tdelay__L"=w120:i32)  [unwired: 11 in]
              n38 = call "myRIO_BRig_RT_dataMTrig_Solenoid_Tdelay__R.vi"() -> ("output_Solenoid_Tdelay__R"=w119:i32)  [unwired: 11 in]
              n39 = local read "MTrig_Solenoid_Tcycle__L"() -> (w131:u16)
              n40 = local read "MTrig_Solenoid_Tcycle__R"() -> (w132:u16)
              n41 = local read "MTrig_Laser_Tcycle"() -> (w111:u16)
              n42 = call "myRIO_BRig_RT_dataMTrig_init.vi"() -> ("output_dataMTrig"=w125:u16[])  [unwired: 5 in]
              n43 = local write "RewCalib_Trig_R"(w114) -> ()
              n44 = local write "RewCalib_Trig_L"(w114) -> ()
              n45 = local read "Tcycle_Cue_min"() -> (w112:u16)
              n46 = Replace Array Subset(array=w125, new element #1=w131, index #1=w126, new element #2=w132, index #2=w127, new element #3=w112, index #3=w128, new element #4=w112, index #4=w129, new element #5=w111, index #5=w130, new element #6=w110, index #6=w122, new element #7=w110, index #7=w121, new element #8=w110, index #8=w120, new element #9=w110, index #9=w119) -> (w124:u16[])
            }
            frame "UploadSettings_pre" {
              # "When the Host sends settings,\nnot all files send at the same time.\n\nIf RT reads the settings faster\nthan the Host can send them,\nthen we will skip settings.\n\nSolution:\nWait 20 cycles"
              n47 = Increment(x=w145) -> (x+1=w144:u16)
              n48 = Greater?(x=w144, y=u16 20) -> (0:w142:bool)
              n49 = Select(t=myRIO_BRig_RT__Case_NonExp_stateList."UploadSettings_Read_dataExp", s=w142, f=w141) -> (s? t:f=w139:T1)
            }
            frame "UploadSettings_Read_dataExp" {
              # "grab dataExp and\nstore it in the\ngeneric data array"
              # "dataExp"
              n50 = call "myRIO_BRig_RT_dataExp_init_details.vi"() -> ("output_dataSize"=w152:i32, "output_dataName"=w155:string)  [unwired: 10 in]
              n51 = call "myRIO_BRig_RT_comm_webdav_uploadReceived_check.vi"("input_dataName"=w155) -> ("output_Iexist"=w154:bool, "output_dataPath"=w153:path)  [unwired: 9 in]
              n52 = case shown="True" w154 {
                tunnel: w153 -> [_ w168]
                tunnel: w152 -> [_ w167]
                tunnel: [_ w166] -> w151
                tunnel: w148 -> [w161 w165]
                tunnel: [w161 w162] -> w147
                frame False {
                }
                frame True {
                  n53 = call "myRIO_BRig_RT_comm_webdav_uploadReceived_read.vi"("input_dataSize"=w167, "input_filePath"=w168) -> ("output_Ivalid"=w166:bool, "output_data"=w164:i64[])  [unwired: 8 in]
                  n54 = To Unsigned Word Integer(number=w164) -> (unsigned 16bit integer=w163:u16[])
                  n55 = Select(t=w163, s=w166, f=w165) -> (s? t:f=w162:u16[])
                }
              }
              n56 = Select(t=myRIO_BRig_RT__Case_NonExp_stateList."UploadSettings_dataExp_1", s=w151, f=myRIO_BRig_RT__Case_NonExp_stateList."UploadSettings_Read_dataLC" ("t")) -> (s? t:f=w146:T1)
            }
            frame "UploadSettings_Read_dataLC" {
              # "grab dataLC and\nstore it in the\ngeneric data array"
              # "dataLC"
              n57 = call "myRIO_BRig_RT_dataLC_init_details.vi"() -> ("output_dataSize"=w175:i32, "output_dataName"=w178:string)  [unwired: 10 in]
              n58 = call "myRIO_BRig_RT_comm_webdav_uploadReceived_check.vi"("input_dataName"=w178) -> ("output_Iexist"=w177:bool, "output_dataPath"=w176:path)  [unwired: 9 in]
              n59 = case shown="True" w177 {
                tunnel: w176 -> [_ w191]
                tunnel: w175 -> [_ w190]
                tunnel: [_ w189] -> w174
                tunnel: w171 -> [w184 w188]
                tunnel: [w184 w185] -> w170
                frame False {
                }
                frame True {
                  n60 = call "myRIO_BRig_RT_comm_webdav_uploadReceived_read.vi"("input_dataSize"=w190, "input_filePath"=w191) -> ("output_Ivalid"=w189:bool, "output_data"=w187:i64[])  [unwired: 8 in]
                  n61 = To Unsigned Word Integer(number=w187) -> (unsigned 16bit integer=w186:u16[])
                  n62 = Select(t=w186, s=w189, f=w188) -> (s? t:f=w185:u16[])
                }
              }
              n63 = Select(t=myRIO_BRig_RT__Case_NonExp_stateList."UploadSettings_dataLC_1", s=w174, f=myRIO_BRig_RT__Case_NonExp_stateList."UploadSettings_Read_dataMTrig" ("t")) -> (s? t:f=w169:T1)
            }
            frame "UploadSettings_Read_dataMTrig" {
              # "grab dataMTrig and\nstore it in the\ngeneric data array"
              # "dataMTrig"
              n64 = call "myRIO_BRig_RT_dataMTrig_init_details.vi"() -> ("output_dataSize"=w198:i32, "output_dataName"=w201:string)  [unwired: 10 in]
              n65 = call "myRIO_BRig_RT_comm_webdav_uploadReceived_check.vi"("input_dataName"=w201) -> ("output_Iexist"=w200:bool, "output_dataPath"=w199:path)  [unwired: 9 in]
              n66 = case shown="True" w200 {
                tunnel: w199 -> [_ w214]
                tunnel: w198 -> [_ w213]
                tunnel: [_ w212] -> w197
                tunnel: w194 -> [w207 w211]
                tunnel: [w207 w208] -> w193
                frame False {
                }
                frame True {
                  n67 = call "myRIO_BRig_RT_comm_webdav_uploadReceived_read.vi"("input_dataSize"=w213, "input_filePath"=w214) -> ("output_Ivalid"=w212:bool, "output_data"=w210:i64[])  [unwired: 8 in]
                  n68 = To Unsigned Word Integer(number=w210) -> (unsigned 16bit integer=w209:u16[])
                  n69 = Select(t=w209, s=w212, f=w211) -> (s? t:f=w208:u16[])
                }
              }
              n70 = Select(t=myRIO_BRig_RT__Case_NonExp_stateList."UploadSettings_dataMTrig_1", s=w197, f=myRIO_BRig_RT__Case_NonExp_stateList."Idle" ("t")) -> (s? t:f=w192:T1)
            }
            frame "UploadSettings_dataExp_1" {
              w218 = u16 1000 ("y")
              # "Cue_max"
              # "Cue_min"
              # "CuePenalty"
              # "Timeout"
              # "Wrong"
              # "Selection"
              # "RewardPost"
              # "Reward_R"
              # "Reward_L"
              # "Tcycle"
              # "TPB_min_R"
              # "TPB_min_L"
              # "TPB_max_R"
              # "TPB_max_L"
              # "I_trialUntilReward"
              # "ENL_penalty"
              # "ENL_min"
              # "ENL_max"
              # "BUR_max"
              # "BUR_min"
              # "CueCycles"
              # "Audio_Freq_R"
              # "Audio_Freq_L"
              # "Audio_Amp_R"
              # "Audio_Amp_L"
              n71 = call "myRIO_BRig_RT_dataExp_CueCycles.vi"() -> ("output_CueCycles"=w261:i32)  [unwired: 11 in]
              n72 = call "myRIO_BRig_RT_dataExp_Audio_amp__R.vi"() -> ("output_Audio_amp__R"=w265:i32)  [unwired: 11 in]
              n73 = call "myRIO_BRig_RT_dataExp_Audio_amp__L.vi"() -> ("output_Audio_amp__L"=w267:i32)  [unwired: 11 in]
              n74 = call "myRIO_BRig_RT_dataExp_BUR_min.vi"() -> ("output_BUR_min"=w258:i32)  [unwired: 11 in]
              n75 = call "myRIO_BRig_RT_dataExp_ENL_min.vi"() -> ("output_ENL_min"=w254:i32)  [unwired: 11 in]
              n76 = call "myRIO_BRig_RT_dataExp_TPB_max__L.vi"() -> ("output_TPB_max__L"=w246:i32)  [unwired: 11 in]
              n77 = call "myRIO_BRig_RT_dataExp_TPB_max__R.vi"() -> ("output_TPB_max__R"=w245:i32)  [unwired: 11 in]
              n78 = call "myRIO_BRig_RT_dataExp_Tcycle_Reward__L.vi"() -> ("output_Tcycle_Reward__L"=w238:i32)  [unwired: 11 in]
              n79 = call "myRIO_BRig_RT_dataExp_Tcycle_Reward__R.vi"() -> ("output_Tcycle_Reward__R"=w237:i32)  [unwired: 11 in]
              n80 = call "myRIO_BRig_RT_dataExp_Tcycle_RewardPost.vi"() -> ("output_Tcycle_RewardPost"=w236:i32)  [unwired: 11 in]
              n81 = call "myRIO_BRig_RT_dataExp_ENL_penalty.vi"() -> ("output_ENL_penalty"=w253:i32)  [unwired: 11 in]
              n82 = call "myRIO_BRig_RT_dataExp_Audio_freq__L.vi"() -> ("output_Audio_freq__L"=w263:i32)  [unwired: 11 in]
              n83 = call "myRIO_BRig_RT_dataExp_Audio_freq__R.vi"() -> ("output_Audio_freq__R"=w262:i32)  [unwired: 11 in]
              n84 = call "myRIO_BRig_RT_dataExp_BUR_max.vi"() -> ("output_BUR_max"=w259:i32)  [unwired: 11 in]
              n85 = call "myRIO_BRig_RT_dataExp_ENL_max.vi"() -> ("output_ENL_max"=w255:i32)  [unwired: 11 in]
              n86 = call "myRIO_BRig_RT_dataExp_ItrialUntilReward.vi"() -> ("output_I_trialUntilReward"=w249:i32)  [unwired: 11 in]
              n87 = call "myRIO_BRig_RT_dataExp_Tcycle_Selection.vi"() -> ("output_Tcycle_Selection"=w235:i32)  [unwired: 11 in]
              n88 = call "myRIO_BRig_RT_dataExp_Tcycle_Wrong.vi"() -> ("output_Tcycle_Wrong"=w234:i32)  [unwired: 11 in]
              n89 = call "myRIO_BRig_RT_dataExp_Tcycle_Timeout.vi"() -> ("output_Tcycle_Timeout"=w233:i32)  [unwired: 11 in]
              n90 = call "myRIO_BRig_RT_dataExp_TPB_min__L.vi"() -> ("output_TPB_min__L"=w244:i32)  [unwired: 11 in]
              n91 = call "myRIO_BRig_RT_dataExp_TPB_min__R.vi"() -> ("output_TPB_min__R"=w243:i32)  [unwired: 11 in]
              n92 = call "myRIO_BRig_RT_dataExp_Tcycle_CuePenalty.vi"() -> ("output_Tcycle_CuePenalty"=w226:i32)  [unwired: 11 in]
              n93 = call "myRIO_BRig_RT_dataExp_Tcycle_Cue_min.vi"() -> ("output_Tcycle_Cue_min"=w225:i32)  [unwired: 11 in]
              n94 = call "myRIO_BRig_RT_dataExp_Tcycle_Cue_max.vi"() -> ("output_Tcycle_Cue_max"=w224:i32)  [unwired: 11 in]
              n95 = Index Array(array=w217, index #1=w267, index #2=w265, index #3=w263, index #4=w262, index #5=w261, index #6=w259, index #7=w258, index #8=w255, index #9=w254, index #10=w253, index #11=w249, index #12=w246, index #13=w245, index #14=w244, index #15=w243, index #16=w238, index #17=w237, index #18=w236, index #19=w235, index #20=w234, index #21=w233, index #22=w226, index #23=w225, index #24=w224) -> (element #1=w266:u16, element #2=w264:u16, element #3=w221:u16, element #4=w220:u16, element #5=w260:u16, element #6=w257:u16, element #7=w256:u16, element #8=w252:u16, element #9=w251:u16, element #10=w250:u16, element #11=w247:u16, element #12=w242:u16, element #13=w241:u16, element #14=w240:u16, element #15=w239:u16, element #16=w232:u16, element #17=w231:u16, element #18=w230:u16, element #19=w229:u16, element #20=w228:u16, element #21=w227:u16, element #22=w223:u16, element #23=w216:u16, element #24=w215:u16)
              n96 = local write "Tcycle_Selection"(w229) -> ()
              n97 = local write "Tcycle_Wrong"(w228) -> ()
              n98 = local write "Tcycle_Timeout"(w227) -> ()
              n99 = local write "Audio_Amp__L"(w266) -> ()
              n100 = local write "Audio_Amp__R"(w264) -> ()
              n101 = local write "Tcycle_ENLPenalty"(w250) -> ()
              n102 = local write "Tcycle_ENL_max"(w252) -> ()
              n103 = local write "TpB_Min_L"(w240) -> ()
              n104 = local write "TpB_Min_R"(w239) -> ()
              n105 = local write "Tcycle_CuePenalty"(w223) -> ()
              n106 = local write "Tcycle_Cue_min"(w216) -> ()
              n107 = local write "Tcycle_Cue_max"(w215) -> ()
              n108 = Quotient & Remainder(x=w221, y=w218) -> (floor(x/y)=w222:u16)  [unwired: 1 out]
              n109 = Quotient & Remainder(x=w220, y=w218) -> (floor(x/y)=w219:u16)  [unwired: 1 out]
              n110 = Not Equal To 0?(x=w247) -> (x != 0?=w248:bool)
              n111 = local write "Tcycle_Reward_L"(w232) -> ()
              n112 = local write "Tcycle_Reward_R"(w231) -> ()
              n113 = local write "Tcycle_RewardPost"(w230) -> ()
              n114 = local write "CueCycles"(w260) -> ()
              n115 = local write "BUR_min"(w256) -> ()
              n116 = local write "BUR_max"(w257) -> ()
              n117 = local write "Tcycle_ENL_min"(w251) -> ()
              n118 = local write "TpB_Max_L"(w242) -> ()
              n119 = local write "TpB_Max_R"(w241) -> ()
              n120 = local write "TrialUntilReward"(w248) -> ()
              n121 = local write "Audio_Freq__L"(w222) -> ()
              n122 = local write "Audio_Freq__R"(w219) -> ()
            }
            frame "UploadSettings_dataLC_1" {
              # "Cue1_delayOpt"
              # "ENL1_delayOpt"
              # "ENL1"
              # "Cue2"
              # "Cue1"
              # "Trial"
              # "Tdelay"
              # "Prob"
              # "OnOff"
              # "Block"
              # "ENL2"
              # "Trial"
              # "Tdelay"
              # "Prob"
              # "OnOff"
              # "Block"
              # "Trial"
              # "Tdelay"
              # "Prob"
              # "Block"
              # "OnOff"
              # "Trial"
              # "Tdelay"
              # "Prob"
              # "OnOff"
              # "Block"
              n123 = call "myRIO_BRig_RT_dataLC_Cue1_First_Block.vi"() -> ("output_Cue1_First_Block"=w324:i32)  [unwired: 11 in]
              n124 = call "myRIO_BRig_RT_dataLC_Cue1_First_OnOff.vi"() -> ("output_Cue1_First_OnOff"=w322:i32)  [unwired: 11 in]
              n125 = call "myRIO_BRig_RT_dataLC_Cue1_First_Count.vi"() -> ("output_Cue1_First_Count"=w319:i32)  [unwired: 11 in]
              n126 = call "myRIO_BRig_RT_dataLC_Cue1_All_Block.vi"() -> ("output_Cue1_All_Block"=w306:i32)  [unwired: 11 in]
              n127 = call "myRIO_BRig_RT_dataLC_Cue1_All_OnOff.vi"() -> ("output_Cue1_All_OnOff"=w305:i32)  [unwired: 11 in]
              n128 = call "myRIO_BRig_RT_dataLC_Cue1_All_Count.vi"() -> ("output_Cue1_All_Count"=w316:i32)  [unwired: 11 in]
              n129 = call "myRIO_BRig_RT_dataLC_ENL1_First_Block.vi"() -> ("output_ENL1_First_Block"=w304:i32)  [unwired: 11 in]
              n130 = call "myRIO_BRig_RT_dataLC_ENL1_First_OnOff.vi"() -> ("output_ENL1_First_OnOff"=w315:i32)  [unwired: 11 in]
              n131 = call "myRIO_BRig_RT_dataLC_ENL1_First_Count.vi"() -> ("output_ENL1_First_Count"=w312:i32)  [unwired: 11 in]
              n132 = call "myRIO_BRig_RT_dataLC_ENL1_All_Block.vi"() -> ("output_ENL1_All_Block"=w311:i32)  [unwired: 11 in]
              n133 = call "myRIO_BRig_RT_dataLC_ENL1_All_OnOff.vi"() -> ("output_ENL1_All_OnOff"=w310:i32)  [unwired: 11 in]
              n134 = call "myRIO_BRig_RT_dataLC_ENL1_All_Count.vi"() -> ("output_ENL1_All_Count"=w307:i32)  [unwired: 11 in]
              n135 = call "myRIO_BRig_RT_dataLC_ENL1_First_delayOpt.vi"() -> ("output_ENL1_First_delayOpt"=w279:i32)  [unwired: 11 in]
              n136 = call "myRIO_BRig_RT_dataLC_Cue1_First_delayOpt.vi"() -> ("output_Cue1_First_delayOpt"=w278:i32)  [unwired: 11 in]
              n137 = call "myRIO_BRig_RT_dataLC_Cue1_First_Probability.vi"() -> ("output_Cue1_First_Probability"=w321:i32)  [unwired: 11 in]
              n138 = call "myRIO_BRig_RT_dataLC_Cue1_First_Tdelay.vi"() -> ("output_Cue1_First_Tdelay"=w320:i32)  [unwired: 11 in]
              n139 = call "myRIO_BRig_RT_dataLC_Cue1_All_Probability.vi"() -> ("output_Cue1_All_Probability"=w318:i32)  [unwired: 11 in]
              n140 = call "myRIO_BRig_RT_dataLC_Cue1_All_Tdelay.vi"() -> ("output_Cue1_All_Tdelay"=w317:i32)  [unwired: 11 in]
              n141 = call "myRIO_BRig_RT_dataLC_ENL1_First_Probability.vi"() -> ("output_ENL1_First_Probability"=w314:i32)  [unwired: 11 in]
              n142 = call "myRIO_BRig_RT_dataLC_ENL1_First_Tdelay.vi"() -> ("output_ENL1_First_Tdelay"=w313:i32)  [unwired: 11 in]
              n143 = call "myRIO_BRig_RT_dataLC_ENL1_All_Probability.vi"() -> ("output_ENL1_All_Probability"=w309:i32)  [unwired: 11 in]
              n144 = call "myRIO_BRig_RT_dataLC_ENL1_All_Tdelay.vi"() -> ("output_ENL1_All_Tdelay"=w308:i32)  [unwired: 11 in]
              n145 = Index Array(array=w280, index #1=w324, index #2=w322, index #3=w321, index #4=w320, index #5=w319, index #6=w306, index #7=w305, index #8=w318, index #9=w317, index #10=w316, index #11=w304, index #12=w315, index #13=w314, index #14=w313, index #15=w312, index #16=w311, index #17=w310, index #18=w309, index #19=w308, index #20=w307, index #21=w279, index #22=w278) -> (element #1=w323:u16, element #2=w302:u16, element #3=w301:u16, element #4=w300:u16, element #5=w299:u16, element #6=w295:u16, element #7=w294:u16, element #8=w293:u16, element #9=w292:u16, element #10=w291:u16, element #11=w290:u16, element #12=w289:u16, element #13=w288:u16, element #14=w287:u16, element #15=w286:u16, element #16=w285:u16, element #17=w284:u16, element #18=w283:u16, element #19=w282:u16, element #20=w281:u16, element #21=w276:u16, element #22=w274:u16)
              n146 = Not Equal To 0?(x=w276) -> (x != 0?=w277:bool)
              n147 = Not Equal To 0?(x=w274) -> (x != 0?=w275:bool)
              n148 = Not Equal To 0?(x=w302) -> (x != 0?=w303:bool)
              n149 = Not Equal To 0?(x=w294) -> (x != 0?=w298:bool)
              n150 = Not Equal To 0?(x=w289) -> (x != 0?=w297:bool)
              n151 = Not Equal To 0?(x=w284) -> (x != 0?=w296:bool)
              n152 = local write "LC_Cue1_Probability"(w301) -> ()
              n153 = local write "LC_ENL1_delayOpt"(w277) -> ()
              n154 = local write "LC_Cue1_delayOpt"(w275) -> ()
              n155 = local write "LC_Cue2_Probability"(w293) -> ()
              n156 = local write "LC_ENL1_Probability"(w288) -> ()
              n157 = local write "LC_ENL2_Probability"(w283) -> ()
              n158 = local write "LC_Cue1_Tdelay"(w300) -> ()
              n159 = local write "LC_Cue1_OnOff"(w303) -> ()
              n160 = local write "LC_Cue1_Block"(w323) -> ()
              n161 = local write "LC_Cue2_Tdelay"(w292) -> ()
              n162 = local write "LC_ENL1_Tdelay"(w287) -> ()
              n163 = local write "LC_Cue2_OnOff"(w298) -> ()
              n164 = local write "LC_ENL1_OnOff"(w297) -> ()
              n165 = local write "LC_Cue1_Trial"(w299) -> ()
              n166 = local write "LC_Cue2_Block"(w295) -> ()
              n167 = local write "LC_ENL1_Block"(w290) -> ()
              n168 = local write "LC_ENL2_Tdelay"(w282) -> ()
              n169 = local write "LC_ENL2_OnOff"(w296) -> ()
              n170 = local write "LC_Cue2_Trial"(w291) -> ()
              n171 = local write "LC_ENL1_Trial"(w286) -> ()
              n172 = local write "LC_ENL2_Block"(w285) -> ()
              n173 = local write "LC_ENL2_Trial"(w281) -> ()
            }
            frame "UploadSettings_dataLC_2" {
              # "Wrong"
              # "Reward"
              # "Trial"
              # "Tdelay"
              # "Prob"
              # "Block"
              # "OnOff"
              # "Trial"
              # "Tdelay"
              # "Prob"
              # "OnOff"
              # "Block"
              n174 = call "myRIO_BRig_RT_dataLC_Reward_Block.vi"() -> ("output_Reward_Block"=w357:i32)  [unwired: 11 in]
              n175 = call "myRIO_BRig_RT_dataLC_Reward_OnOff.vi"() -> ("output_Reward_OnOff"=w355:i32)  [unwired: 11 in]
              n176 = call "myRIO_BRig_RT_dataLC_Reward_Trial.vi"() -> ("output_Reward_Trial"=w352:i32)  [unwired: 11 in]
              n177 = call "myRIO_BRig_RT_dataLC_Wrong_Block.vi"() -> ("output_Wrong_Block"=w348:i32)  [unwired: 11 in]
              n178 = call "myRIO_BRig_RT_dataLC_Wrong_OnOff.vi"() -> ("output_Wrong_OnOff"=w347:i32)  [unwired: 11 in]
              n179 = call "myRIO_BRig_RT_dataLC_Wrong_Trial.vi"() -> ("output_Wrong_Trial"=w349:i32)  [unwired: 11 in]
              n180 = call "myRIO_BRig_RT_dataLC_Reward_Probability.vi"() -> ("output_Reward_Probability"=w354:i32)  [unwired: 11 in]
              n181 = call "myRIO_BRig_RT_dataLC_Reward_Tdelay.vi"() -> ("output_Reward_Tdelay"=w353:i32)  [unwired: 11 in]
              n182 = call "myRIO_BRig_RT_dataLC_Wrong_Probability.vi"() -> ("output_Wrong_Probability"=w351:i32)  [unwired: 11 in]
              n183 = call "myRIO_BRig_RT_dataLC_Wrong_Tdelay.vi"() -> ("output_Wrong_Tdelay"=w350:i32)  [unwired: 11 in]
              n184 = Index Array(array=w331, index #1=w357, index #2=w355, index #3=w354, index #4=w353, index #5=w352, index #6=w348, index #7=w347, index #8=w351, index #9=w350, index #10=w349) -> (element #1=w356:u16, element #2=w345:u16, element #3=w344:u16, element #4=w343:u16, element #5=w342:u16, element #6=w340:u16, element #7=w339:u16, element #8=w338:u16, element #9=w337:u16, element #10=w336:u16)
              n185 = Not Equal To 0?(x=w345) -> (x != 0?=w346:bool)
              n186 = Not Equal To 0?(x=w339) -> (x != 0?=w341:bool)
              n187 = local write "LC_Reward_Probability"(w344) -> ()
              n188 = local write "LC_Wrong_Probability"(w338) -> ()
              n189 = local write "LC_Reward_Tdelay"(w343) -> ()
              n190 = local write "LC_Reward_OnOff"(w346) -> ()
              n191 = local write "LC_Reward_Block"(w356) -> ()
              n192 = local write "LC_Reward_Trial"(w342) -> ()
              n193 = local write "LC_Wrong_Tdelay"(w337) -> ()
              n194 = local write "LC_Wrong_OnOff"(w341) -> ()
              n195 = local write "LC_Wrong_Block"(w340) -> ()
              n196 = local write "LC_Wrong_Trial"(w336) -> ()
            }
            frame "UploadSettings_dataMTrig_1" {
              # "Tdelay_R"
              # "Tdelay_L"
              # "Tcycle_R"
              # "Tcycle_L"
              # "RewCalib_nCycle_R"
              # "RewCalib_nCycle_L"
              # "Solenoid"
              # "Laser_Tcycle"
              n197 = call "myRIO_BRig_RT_dataMTrig_Laser_Tcycle.vi"() -> ("output_Laser_Tcycle"=w367:i32)  [unwired: 11 in]
              n198 = call "myRIO_BRig_RT_dataMTrig_Solenoid_RewCalib_nCycle__L.vi"() -> ("output_Solenoid_RewCalib_nCycle__L"=w366:i32)  [unwired: 11 in]
              n199 = call "myRIO_BRig_RT_dataMTrig_Solenoid_RewCalib_nCycle__R.vi"() -> ("output_Solenoid_RewCalib_nCycle__R"=w365:i32)  [unwired: 11 in]
              n200 = call "myRIO_BRig_RT_dataMTrig_Solenoid_Tdelay__L.vi"() -> ("output_Solenoid_Tdelay__L"=w362:i32)  [unwired: 11 in]
              n201 = call "myRIO_BRig_RT_dataMTrig_Solenoid_Tdelay__R.vi"() -> ("output_Solenoid_Tdelay__R"=w361:i32)  [unwired: 11 in]
              n202 = call "myRIO_BRig_RT_dataMTrig_Solenoid_Tcycle__L.vi"() -> ("output_Solenoid_Tcycle__L"=w364:i32)  [unwired: 11 in]
              n203 = call "myRIO_BRig_RT_dataMTrig_Solenoid_Tcycle__R.vi"() -> ("output_Solenoid_Tcycle__R"=w363:i32)  [unwired: 11 in]
              n204 = Index Array(array=w360, index #1=w367, index #2=w366, index #3=w365, index #4=w364, index #5=w363, index #6=w362, index #7=w361) -> (element #1=w374:u16, element #2=w373:u16, element #3=w372:u16, element #4=w371:u16, element #5=w370:u16, element #6=w369:u16, element #7=w368:u16)
              n205 = Replace Array Subset(array=w380, new element #1=w374, index #1=w367, new element #2=w373, index #2=w366, new element #3=w372, index #3=w365, new element #4=w371, index #4=w364, new element #5=w370, index #5=w363, new element #6=w369, index #6=w362, new element #7=w368, index #7=w361) -> (w379:u16[])
              n206 = local write "MTrig_Solenoid_Tcycle__L"(w371) -> ()
              n207 = local write "MTrig_Solenoid_Tcycle__R"(w370) -> ()
              n208 = local write "MTrig_Laser_Tcycle"(w374) -> ()
            }
            frame "Idle" {
              w400 = u16 1000 ("y")
              # "To ensure timing, we split the\nidle state into 4 phases"
              # "Laser_Tcycle"
              # "Audio_Tcycle_R"
              # "Audio_Tcycle_L"
              n209 = local read "MTrig_Audio_trig__L"() -> (w389:bool)
              n210 = local read "MTrig_Audio_trig__R"() -> (w391:bool)
              n211 = Select(t=myRIO_BRig_RT__Case_NonExp_stateList."SendData" ("Enum"), s="SendData", f=myRIO_BRig_RT__Case_NonExp_stateList."Idle_2" ("Enum")) -> (s? t:f=w384:T1)
              n212 = local read "MTrig_Laser_trig"() -> (w390:bool)
              n213 = call "myRIO_BRig_RT_dataMTrig_Audio_Tcycle__L.vi"() -> ("output_Audio_Tcycle__L"=w407:i32)  [unwired: 11 in]
              n214 = call "myRIO_BRig_RT_dataMTrig_Audio_Tcycle__R.vi"() -> ("output_Audio_Tcycle__R"=w406:i32)  [unwired: 11 in]
              n215 = call "myRIO_BRig_RT_dataMTrig_Laser_Tcycle.vi"() -> ("output_Laser_Tcycle"=w405:i32)  [unwired: 11 in]
              n216 = local read "MTrig_Laser_Tcycle"() -> (w382:u16)
              n217 = Select(t=myRIO_BRig_RT__Case_NonExp_stateList."TestConnection" ("Enum"), s="TestConnection", f=w384) -> (s? t:f=w393:T1)
              n218 = local read "Tcycle_Cue_min"() -> (w383:u16)
              n219 = Compound Arithmetic op=OR(w389, w391, w390) -> (w392:bool)
              n220 = case shown="True" w392 {
                frame False {
                }
                frame True {
                  w408 = FALSE
                  n221 = local write "MTrig_Audio_trig__L"(w408) -> ()
                  n222 = local write "MTrig_Audio_trig__R"(w408) -> ()
                  n223 = local write "MTrig_Laser_trig"(w408) -> ()
                }
              }
              n224 = Replace Array Subset(array=w403, new element #1=w383, index #1=w407, new element #2=w383, index #2=w406, new element #3=w382, index #3=w405) -> (w404:u16[])
              n225 = local read "Audio_Amp__R"() -> (w396:u16)
              n226 = local read "Audio_Amp__L"() -> (w397:u16)
              n227 = local read "Audio_Freq__R"() -> (w394:u16)
              n228 = local read "Audio_Freq__L"() -> (w395:u16)
              n229 = Multiply(x=w394, y=w400) -> (x*y=w398:u16)
              n230 = Multiply(x=w395, y=w400) -> (x*y=w399:u16)
            }
            frame "Idle_2" {
              # "To ensure timing, we split the\nidle state into 4 phases"
              # "Ncycles"
              # "Ncycles"
              # "RewCalib"
              # "RewCalib"
              # "Solenoid R"
              # "Solenoid L"
              n231 = call "myRIO_BRig_RT_dataMTrig_Solenoid_RewCalib_OnOff__L.vi"() -> ("output_Solenoid_RewCalib_OnOff__L"=w438:i32)  [unwired: 11 in]
              n232 = call "myRIO_BRig_RT_dataMTrig_Solenoid_N__L.vi"() -> ("output_Solenoid_N__L"=w426:i32)  [unwired: 11 in]
              n233 = call "myRIO_BRig_RT_dataMTrig_Solenoid_RewCalib_OnOff__R.vi"() -> ("output_Solenoid_RewCalib_OnOff__R"=w423:i32)  [unwired: 11 in]
              n234 = call "myRIO_BRig_RT_dataMTrig_Solenoid_N__R.vi"() -> ("output_Solenoid_N__R"=w422:i32)  [unwired: 11 in]
              n235 = Index Array(array=w429, index #1=w438, index #2=w426, index #3=w423, index #4=w422) -> (element #1=w425:u16, element #2=w420:u16, element #3=w421:u16, element #4=w419:u16)
              n236 = local read "RewCalib_Trig_L"() -> (w418:bool)
              n237 = local read "RewCalib_Trig_R"() -> (w417:bool)
              n238 = Equal To 0?(x=w420) -> (x = 0?=w428:bool)
              n239 = Equal To 0?(x=w419) -> (x = 0?=w427:bool)
              n240 = Not Equal To 0?(x=w421) -> (x != 0?=w439:bool)
              n241 = Not Equal To 0?(x=w425) -> (x != 0?=w440:bool)
              n242 = And(x=w428, y=w427) -> (x .and. y?=w432:bool)
              n243 = Or(x=w418, y=w417) -> (x .or. y?=w433:bool)
              n244 = Not Exclusive Or(1:w440, 2:w418) -> (0:w435:bool)
              n245 = Not Exclusive Or(1:w439, 2:w417) -> (0:w437:bool)
              n246 = And(x=w433, y=w432) -> (x .and. y?=w415:bool)
              n247 = Not(x=w435) -> (.not. x?=w434:bool)
              n248 = Not(x=w437) -> (.not. x?=w436:bool)
              n249 = Or(x=w434, y=w436) -> (x .or. y?=w416:bool)
              n250 = Or(x=w415, y=w416) -> (x .or. y?=w431:bool)
              n251 = Select(t=myRIO_BRig_RT__Case_NonExp_stateList."RewardCalibration_pre" ("Enum"), s=w431, f=myRIO_BRig_RT__Case_NonExp_stateList."Idle_3" ("Enum")) -> (s? t:f=w414:T1)
            }
            frame "Idle_3" {
              w463 = u8 0 ("f")
              # "To ensure timing, we split the\nidle state into 4 phases"
              n252 = local read "MTrig_Solenoid_trig__L"() -> (w449:bool)
              n253 = local read "MTrig_Solenoid_trig__R"() -> (w464:bool)
              n254 = local read "warmupType"() -> (w455:bool)
              n255 = local read "warmup"() -> (w456:bool)
              n256 = Not(x=w455) -> (.not. x?=w457:bool)
              n257 = Select(t=u8 1, s=w449, f=w463) -> (s? t:f=w462:u8)
              n258 = Select(t=u8 2, s=w464, f=w463) -> (s? t:f=w461:u8)
              n259 = And(x=w456, y=w457) -> (x .and. y?=w454:bool)
              n260 = And(x=w456, y=w455) -> (x .and. y?=w444:bool)
              n261 = Add(x=w462, y=w461) -> (x+y=w460:u8)
              n262 = case shown="3" w460 {
                tunnel: w459 -> [w467 w471 w489 w507]
                tunnel: [w467 w470 w488 w506] -> w458
                tunnel: w454 -> [_ w469 w487 w505]
                tunnel: [_ TRUE TRUE TRUE] -> w446
                frame 0, Default {
                }
                frame 1 {
                  n263 = case shown="True" w469 {
                    tunnel: w471 -> [w480 w485]
                    tunnel: [w479 w484] -> w470
                    frame True {
                      # "Audio_L"
                      # "Solenoid_L"
                      n264 = call "myRIO_BRig_RT_dataMTrig_Solenoid_N__L.vi"() -> ("output_Solenoid_N__L"=w476:i32)  [unwired: 11 in]
                      n265 = call "myRIO_BRig_RT_dataMTrig_Audio_N__L.vi"() -> ("output_Audio_N__L"=w474:i32)  [unwired: 11 in]
                      n266 = Index Array(array=w480, index #1=w476, index #2=w474) -> (element #1=w478:u16, element #2=w477:u16)
                      n267 = Increment(x=w478) -> (x+1=w475:u16)
                      n268 = Increment(x=w477) -> (x+1=w473:u16)
                      n269 = Replace Array Subset(array=w480, new element #1=w475, index #1=w476, new element #2=w473, index #2=w474) -> (w479:u16[])
                    }
                    frame False {
                      # "Solenoid_L"
                      n270 = call "myRIO_BRig_RT_dataMTrig_Solenoid_N__L.vi"() -> ("output_Solenoid_N__L"=w482:i32)  [unwired: 11 in]
                      n271 = Index Array(array=w485, index=w482) -> (element=w483:u16)
                      n272 = Increment(x=w483) -> (x+1=w481:u16)
                      n273 = Replace Array Subset(array=w485, new element=w481, index=w482) -> (w484:u16[])
                    }
                  }
                  n274 = local write "MTrig_Solenoid_trig__L"(FALSE) -> ()
                }
                frame 2 {
                  n275 = case shown="True" w487 {
                    tunnel: w489 -> [w498 w503]
                    tunnel: [w497 w502] -> w488
                    frame True {
                      # "Audio_R"
                      # "Solenoid_R"
                      n276 = call "myRIO_BRig_RT_dataMTrig_Solenoid_N__R.vi"() -> ("output_Solenoid_N__R"=w494:i32)  [unwired: 11 in]
                      n277 = call "myRIO_BRig_RT_dataMTrig_Audio_N__R.vi"() -> ("output_Audio_N__R"=w493:i32)  [unwired: 11 in]
                      n278 = Index Array(array=w498, index #1=w494, index #2=w493) -> (element #1=w496:u16, element #2=w495:u16)
                      n279 = Increment(x=w495) -> (x+1=w491:u16)
                      n280 = Increment(x=w496) -> (x+1=w492:u16)
                      n281 = Replace Array Subset(array=w498, new element #1=w492, index #1=w494, new element #2=w491, index #2=w493) -> (w497:u16[])
                    }
                    frame False {
                      # "Solenoid_R"
                      n282 = call "myRIO_BRig_RT_dataMTrig_Solenoid_N__R.vi"() -> ("output_Solenoid_N__R"=w499:i32)  [unwired: 11 in]
                      n283 = Index Array(array=w503, index=w499) -> (element=w501:u16)
                      n284 = Increment(x=w501) -> (x+1=w500:u16)
                      n285 = Replace Array Subset(array=w503, new element=w500, index=w499) -> (w502:u16[])
                    }
                  }
                  n286 = local write "MTrig_Solenoid_trig__R"(FALSE) -> ()
                }
                frame 3 {
                  w508 = FALSE
                  n287 = case shown="True" w505 {
                    tunnel: w507 -> [w522 w530]
                    tunnel: [w521 w529] -> w506
                    frame True {
                      # "Audio_R"
                      # "Solenoid_R"
                      # "Audio_L"
                      # "Solenoid_L"
                      n288 = call "myRIO_BRig_RT_dataMTrig_Solenoid_N__L.vi"() -> ("output_Solenoid_N__L"=w516:i32)  [unwired: 11 in]
                      n289 = call "myRIO_BRig_RT_dataMTrig_Audio_N__L.vi"() -> ("output_Audio_N__L"=w514:i32)  [unwired: 11 in]
                      n290 = call "myRIO_BRig_RT_dataMTrig_Solenoid_N__R.vi"() -> ("output_Solenoid_N__R"=w512:i32)  [unwired: 11 in]
                      n291 = call "myRIO_BRig_RT_dataMTrig_Audio_N__R.vi"() -> ("output_Audio_N__R"=w511:i32)  [unwired: 11 in]
                      n292 = Index Array(array=w522, index #1=w516, index #2=w514, index #3=w512, index #4=w511) -> (element #1=w520:u16, element #2=w519:u16, element #3=w518:u16, element #4=w517:u16)
                      n293 = Increment(x=w517) -> (x+1=w509:u16)
                      n294 = Increment(x=w520) -> (x+1=w515:u16)
                      n295 = Increment(x=w519) -> (x+1=w513:u16)
                      n296 = Increment(x=w518) -> (x+1=w510:u16)
                      n297 = Replace Array Subset(array=w522, new element #1=w515, index #1=w516, new element #2=w513, index #2=w514, new element #3=w510, index #3=w512, new element #4=w509, index #4=w511) -> (w521:u16[])
                    }
                    frame False {
                      # "Solenoid_R"
                      # "Solenoid_L"
                      n298 = call "myRIO_BRig_RT_dataMTrig_Solenoid_N__L.vi"() -> ("output_Solenoid_N__L"=w526:i32)  [unwired: 11 in]
                      n299 = call "myRIO_BRig_RT_dataMTrig_Solenoid_N__R.vi"() -> ("output_Solenoid_N__R"=w523:i32)  [unwired: 11 in]
                      n300 = Index Array(array=w530, index #1=w526, index #2=w523) -> (element #1=w528:u16, element #2=w527:u16)
                      n301 = Increment(x=w528) -> (x+1=w525:u16)
                      n302 = Increment(x=w527) -> (x+1=w524:u16)
                      n303 = Replace Array Subset(array=w530, new element #1=w525, index #1=w526, new element #2=w524, index #2=w523) -> (w529:u16[])
                    }
                  }
                  n304 = local write "MTrig_Solenoid_trig__L"(w508) -> ()
                  n305 = local write "MTrig_Solenoid_trig__R"(w508) -> ()
                }
              }
              n306 = Select(t=myRIO_BRig_RT__Case_NonExp_stateList."Cue_pre", s=w444, f=myRIO_BRig_RT__Case_NonExp_stateList."DispenseWater_pre" ("Enum")) -> (s? t:f=w442:T1)
              n307 = Select(t=w442, s=w446, f=myRIO_BRig_RT__Case_NonExp_stateList."Idle_4" ("Enum")) -> (s? t:f=w447:T1)
            }
            frame "Idle_4" {
              # "use dataMTrig as it is one of the last to transfer"
              # "To ensure timing, we split the\nidle state into 4 phases"
              n308 = call "myRIO_BRig_RT_comm_webdav_uploadReceived_check_v2,0.vi"("input_dataName"="dataMTrig") -> ("output_Iexist"=w540:bool)  [unwired: 9 in, 1 out]
              n309 = Select(t=myRIO_BRig_RT__Case_NonExp_stateList."UploadSettings_pre" ("Enum"), s=w540, f=myRIO_BRig_RT__Case_NonExp_stateList."Idle") -> (s? t:f=w538:T1)
            }
            frame "Cue_pre" {
              w548 = u16 1 ("t")
              w547 = u16 0 ("new element/subarray")
              w544 = u16 0 ("new element/subarray")
              # "Ncycle"
              # "count"
              # "Audio_R"
              # "Solenoid_R"
              # "Solenoid_L"
              # "Ncycle"
              # "count"
              # "Audio_L"
              n310 = call "myRIO_BRig_RT_dataMTrig_Solenoid_N__L.vi"() -> ("output_Solenoid_N__L"=w559:i32)  [unwired: 11 in]
              n311 = call "myRIO_BRig_RT_dataMTrig_Solenoid_N__R.vi"() -> ("output_Solenoid_N__R"=w558:i32)  [unwired: 11 in]
              n312 = Index Array(array=w555, index #1=w559, index #2=w558) -> (element #1=w557:u16, element #2=w556:u16)
              n313 = Not Equal To 0?(x=w556) -> (x != 0?=w549:bool)
              n314 = Not Equal To 0?(x=w557) -> (x != 0?=w551:bool)
              n315 = Select(t=w548, s=w551, f=w547) -> (s? t:f=w550:u16)
              n316 = Select(t=w548, s=w549, f=w547) -> (s? t:f=w543:u16)
              n317 = call "myRIO_BRig_RT_dataMTrig_Audio_c__L.vi"() -> ("output_Audio_c__L"=w553:i32)  [unwired: 11 in]
              n318 = call "myRIO_BRig_RT_dataMTrig_Audio_N__L.vi"() -> ("output_Audio_N__L"=w552:i32)  [unwired: 11 in]
              n319 = call "myRIO_BRig_RT_dataMTrig_Audio_c__R.vi"() -> ("output_Audio_c__R"=w546:i32)  [unwired: 11 in]
              n320 = call "myRIO_BRig_RT_dataMTrig_Audio_N__R.vi"() -> ("output_Audio_N__R"=w545:i32)  [unwired: 11 in]
              n321 = Replace Array Subset(array=w555, new element #1=w544, index #1=w553, new element #2=w550, index #2=w552, new element #3=w544, index #3=w546, new element #4=w543, index #4=w545) -> (w554:u16[])
            }
            frame "Cue" {
              # "Ncycle"
              # "Audio_R"
              # "Ncycle"
              # "Audio_L"
              n322 = call "myRIO_BRig_RT_dataMTrig_Audio_N__L.vi"() -> ("output_Audio_N__L"=w575:i32)  [unwired: 11 in]
              n323 = call "myRIO_BRig_RT_dataMTrig_Audio_N__R.vi"() -> ("output_Audio_N__R"=w574:i32)  [unwired: 11 in]
              n324 = Index Array(array=w580, index #1=w575, index #2=w574) -> (element #1=w573:u16, element #2=w572:u16)
              n325 = Equal To 0?(x=w573) -> (x = 0?=w571:bool)
              n326 = Equal To 0?(x=w572) -> (x = 0?=w570:bool)
              n327 = And(x=w571, y=w570) -> (x .and. y?=w569:bool)
              n328 = Select(t=myRIO_BRig_RT__Case_NonExp_stateList."DispenseWater_pre", s=w569, f=w567) -> (s? t:f=w566:T1)
            }
            frame "RewardCalibration_pre" {
              (unwired) FALSE
              w586 = FALSE
              w597 = u8 0
              w613 = u8 0
              # "Are we starting a RewardCalibration?\nOr are we stopping a RewardCalibration?\nOr is a RewardCalibration over?"
              # "RewCalib\nOnOff"
              # "N"
              # "Solenoid R"
              # "RewCalib\nOnOff"
              # "N"
              # "Solenoid L"
              n329 = local read "RewCalib_Trig_L"() -> (w620:bool)
              n330 = local read "RewCalib_Trig_R"() -> (w589:bool)
              n331 = call "myRIO_BRig_RT_dataMTrig_Solenoid_N__R.vi"() -> ("output_Solenoid_N__R"=w591:i32)  [unwired: 11 in]
              n332 = call "myRIO_BRig_RT_dataMTrig_Solenoid_RewCalib_OnOff__R.vi"() -> ("output_Solenoid_RewCalib_OnOff__R"=w588:i32)  [unwired: 11 in]
              n333 = call "myRIO_BRig_RT_dataMTrig_Solenoid_N__L.vi"() -> ("output_Solenoid_N__L"=w606:i32)  [unwired: 11 in]
              n334 = call "myRIO_BRig_RT_dataMTrig_Solenoid_RewCalib_OnOff__L.vi"() -> ("output_Solenoid_RewCalib_OnOff__L"=w607:i32)  [unwired: 11 in]
              n335 = Index Array(array=w590, index #1=w591, index #2=w588) -> (element #1=w601:u16, element #2=w596:u16)
              n336 = Index Array(array=w590, index #1=w606, index #2=w607) -> (element #1=w617:u16, element #2=w612:u16)
              n337 = Equal To 0?(x=w601) -> (x = 0?=w602:bool)
              n338 = Not Equal To 0?(x=w596) -> (x != 0?=w599:bool)
              n339 = Equal To 0?(x=w617) -> (x = 0?=w618:bool)
              n340 = Not Equal To 0?(x=w612) -> (x != 0?=w615:bool)
              n341 = local write "MTrig_Solenoid_trig__L"(w586) -> ()
              n342 = local write "MTrig_Solenoid_trig__R"(w586) -> ()
              n343 = Select(t=u8 1, s=w589, f=w597) -> (s? t:f=w593:u8)
              n344 = Select(t=u8 1, s=w620, f=w613) -> (s? t:f=w609:u8)
              n345 = Select(t=u8 2, s=w602, f=w597) -> (s? t:f=w594:u8)
              n346 = Select(t=u8 4, s=w599, f=w597) -> (s? t:f=w595:u8)
              n347 = Select(t=u8 2, s=w618, f=w613) -> (s? t:f=w610:u8)
              n348 = Select(t=u8 4, s=w615, f=w613) -> (s? t:f=w611:u8)
              n349 = Compound Arithmetic op=ADD(w593, w594, w595) -> (w592:u8)
              n350 = Compound Arithmetic op=ADD(w609, w610, w611) -> (w608:u8)
              n351 = case shown="7" w608 {
                tunnel: w590 -> [w650 w655 w657 w662 w667 w669 w672 w677]
                tunnel: [w650 w656 w657 w663 w668 w669 w673 w678] -> w605
                tunnel: w607 -> [_ w653 _ w660 w665 _ w671 w676]
                tunnel: w606 -> [_ w654 _ w661 w666 _ _ _]
                frame 0, Default {
                }
                frame 1 {
                  n352 = Replace Array Subset(array=w655, new element #1=u16 100 ("new element/subarray"), index #1=w654, new element #2=u16 1 ("new element/subarray"), index #2=w653) -> (w656:u16[])
                }
                frame 2 {
                }
                frame 3 {
                  n353 = Replace Array Subset(array=w662, new element #1=u16 100 ("new element/subarray"), index #1=w661, new element #2=u16 1 ("new element/subarray"), index #2=w660) -> (w663:u16[])
                }
                frame 4 {
                  w664 = u16 0 ("new element/subarray")
                  n354 = Replace Array Subset(array=w667, new element #1=w664, index #1=w666, new element #2=w664, index #2=w665) -> (w668:u16[])
                }
                frame 5 {
                }
                frame 6 {
                  n355 = Replace Array Subset(array=w672, new element=u16 0 ("new element/subarray"), index=w671) -> (w673:u16[])
                }
                frame 7 {
                  n356 = local write "RewCalib_Trig_L"(FALSE ("RewCalib_Trig_L")) -> ()
                  n357 = Replace Array Subset(array=w677, new element=u16 0 ("new element/subarray"), index=w676) -> (w678:u16[])
                }
              }
              n358 = case shown="7" w592 {
                tunnel: w605 -> [w621 w626 w628 w633 w638 w640 w643 w648]
                tunnel: [w621 w627 w628 w634 w639 w640 w644 w649] -> w604
                tunnel: w588 -> [_ w624 _ w631 w636 _ w642 w647]
                tunnel: w591 -> [_ w625 _ w632 w637 _ _ _]
                frame 0, Default {
                }
                frame 1 {
                  n359 = Replace Array Subset(array=w626, new element #1=u16 100 ("new element/subarray"), index #1=w625, new element #2=u16 1 ("new element/subarray"), index #2=w624) -> (w627:u16[])
                }
                frame 2 {
                }
                frame 3 {
                  n360 = Replace Array Subset(array=w633, new element #1=u16 100 ("new element/subarray"), index #1=w632, new element #2=u16 1 ("new element/subarray"), index #2=w631) -> (w634:u16[])
                }
                frame 4 {
                  w635 = u16 0 ("new element/subarray")
                  n361 = Replace Array Subset(array=w638, new element #1=w635, index #1=w637, new element #2=w635, index #2=w636) -> (w639:u16[])
                }
                frame 5 {
                }
                frame 6 {
                  n362 = Replace Array Subset(array=w643, new element=u16 0 ("new element/subarray"), index=w642) -> (w644:u16[])
                }
                frame 7 {
                  n363 = local write "RewCalib_Trig_R"(FALSE ("RewCalib_Trig_L")) -> ()
                  n364 = Replace Array Subset(array=w648, new element=u16 0 ("new element/subarray"), index=w647) -> (w649:u16[])
                }
              }
            }
            frame "DispenseWater_pre" {
              w685 = u16 0 ("t")
              w728 = u16 0 ("new element/subarray")
              # "just trust me on this one"
              # "RewCalib\nOnOff"
              # "RewCalib\nOnOff"
              # "nCycle"
              # "Solenoid__R"
              # "Tdelay"
              # "delay"
              # "nCycle"
              # "Solenoid__L"
              # "Tdelay"
              # "delay"
              # "Solenoid__R"
              # "count"
              # "Solenoid_Tcycle_R"
              # "Solenoid_Tcycle_L"
              # "Solenoid__L"
              # "count"
              n365 = call "myRIO_BRig_RT_dataMTrig_Solenoid_RewCalib_OnOff__L.vi"() -> ("output_Solenoid_RewCalib_OnOff__L"=w692:i32)  [unwired: 11 in]
              n366 = call "myRIO_BRig_RT_dataMTrig_Solenoid_N__L.vi"() -> ("output_Solenoid_N__L"=w683:i32)  [unwired: 11 in]
              n367 = call "myRIO_BRig_RT_dataMTrig_Solenoid_delay__L.vi"() -> ("output_Solenoid_delay__L"=w726:i32)  [unwired: 11 in]
              n368 = call "myRIO_BRig_RT_dataMTrig_Solenoid_Tdelay__L.vi"() -> ("output_Solenoid_Tdelay__L"=w725:i32)  [unwired: 11 in]
              n369 = call "myRIO_BRig_RT_dataMTrig_Solenoid_N__R.vi"() -> ("output_Solenoid_N__R"=w681:i32)  [unwired: 11 in]
              n370 = call "myRIO_BRig_RT_dataMTrig_Solenoid_delay__R.vi"() -> ("output_Solenoid_delay__R"=w715:i32)  [unwired: 11 in]
              n371 = call "myRIO_BRig_RT_dataMTrig_Solenoid_Tdelay__R.vi"() -> ("output_Solenoid_Tdelay__R"=w714:i32)  [unwired: 11 in]
              n372 = call "myRIO_BRig_RT_dataMTrig_Solenoid_RewCalib_OnOff__R.vi"() -> ("output_Solenoid_RewCalib_OnOff__R"=w688:i32)  [unwired: 11 in]
              n373 = Index Array(array=w727, index #1=w683, index #2=w726, index #3=w725, index #4=w681, index #5=w715, index #6=w714, index #7=w692, index #8=w688) -> (element #1=w684:u16, element #2=w724:u16, element #3=w719:u16, element #4=w687:u16, element #5=w709:u16, element #6=w708:u16, element #7=w693:u16, element #8=w690:u16)
              n374 = Equal To 0?(x=w724) -> (x = 0?=w723:bool)
              n375 = Equal To 0?(x=w709) -> (x = 0?=w713:bool)
              n376 = local read "RewCalib_Trig_L"() -> (w704:bool)
              n377 = local read "RewCalib_Trig_R"() -> (w699:bool)
              n378 = Not Equal To 0?(x=w684) -> (x != 0?=w722:bool)
              n379 = Not Equal To 0?(x=w687) -> (x != 0?=w712:bool)
              n380 = local read "MTrig_Solenoid_Tcycle__L"() -> (w721:u16)
              n381 = local read "MTrig_Solenoid_Tcycle__R"() -> (w707:u16)
              n382 = Not Equal To 0?(x=w693) -> (x != 0?=w703:bool)
              n383 = Not Equal To 0?(x=w690) -> (x != 0?=w701:bool)
              n384 = Not(x=w704) -> (.not. x?=w702:bool)
              n385 = Not(x=w699) -> (.not. x?=w700:bool)
              n386 = And(x=w703, y=w702) -> (x .and. y?=w698:bool)
              n387 = And(x=w701, y=w700) -> (x .and. y?=w697:bool)
              n388 = call "myRIO_BRig_RT_dataMTrig_Solenoid_c__L.vi"() -> ("output_Solenoid_c__L"=w730:i32)  [unwired: 11 in]
              n389 = call "myRIO_BRig_RT_dataMTrig_Solenoid_c__R.vi"() -> ("output_Solenoid_c__R"=w729:i32)  [unwired: 11 in]
              n390 = Select(t=w721, s=w722, f=u16 0) -> (s? t:f=w718:u16)
              n391 = Or(x=w698, y=w697) -> (x .or. y?=w686:bool)
              n392 = Select(t=w707, s=w712, f=u16 0) -> (s? t:f=w710:u16)
              n393 = Select(t=w718, s=w723, f=w719) -> (s? t:f=w716:u16)
              n394 = Select(t=w710, s=w713, f=w708) -> (s? t:f=w705:u16)
              n395 = call "myRIO_BRig_RT_dataMTrig_Solenoid_Tcycle__L.vi"() -> ("output_Solenoid_Tcycle__L"=w717:i32)  [unwired: 11 in]
              n396 = call "myRIO_BRig_RT_dataMTrig_Solenoid_Tcycle__R.vi"() -> ("output_Solenoid_Tcycle__R"=w706:i32)  [unwired: 11 in]
              n397 = Select(t=w685, s=w686, f=w684) -> (s? t:f=w682:u16)
              n398 = Select(t=w685, s=w686, f=w687) -> (s? t:f=w680:u16)
              n399 = Select(t=myRIO_BRig_RT__Case_NonExp_stateList."Idle" ("Enum"), s=w686, f=myRIO_BRig_RT__Case_NonExp_stateList."DispenseWater" ("Enum")) -> (s? t:f=w694:T1)
              n400 = Select(t=w685, s=w686, f=w693) -> (s? t:f=w691:u16)
              n401 = Select(t=w685, s=w686, f=w690) -> (s? t:f=w689:u16)
              n402 = Replace Array Subset(array=w727, new element #1=w728, index #1=w730, new element #2=w728, index #2=w729, new element #3=w716, index #3=w717, new element #4=w705, index #4=w706, new element #5=w691, index #5=w692, new element #6=w689, index #6=w688, new element #7=w682, index #7=w683, new element #8=w680, index #8=w681) -> (w731:u16[])
            }
            frame "DispenseWater" {
              # "D"
              # "C"
              # "B"
              # "A"
              # "(A) Add COUNT and INCREMENT\n(B) Is (A) smaller than Tcycle?\n(C) Are we dispensing water or in the delay phase?\n(D) If (A) is smaller than Tcycle   AND   if we are dispensing water\n      then send TRUE to solenoid"
              # "delay"
              # "Tcycle"
              # "Solenoid__R"
              # "count"
              # "delay"
              # "Tcycle"
              # "Solenoid__L"
              # "count"
              n403 = To Unsigned Word Integer(number=w762) -> (unsigned 16bit integer=w744:u16)
              n404 = call "myRIO_BRig_RT_dataMTrig_Solenoid_delay__R.vi"() -> ("output_Solenoid_delay__R"=w748:i32)  [unwired: 11 in]
              n405 = call "myRIO_BRig_RT_dataMTrig_Solenoid_c__R.vi"() -> ("output_Solenoid_c__R"=w747:i32)  [unwired: 11 in]
              n406 = call "myRIO_BRig_RT_dataMTrig_Solenoid_Tcycle__R.vi"() -> ("output_Solenoid_Tcycle__R"=w749:i32)  [unwired: 11 in]
              n407 = call "myRIO_BRig_RT_dataMTrig_Solenoid_delay__L.vi"() -> ("output_Solenoid_delay__L"=w764:i32)  [unwired: 11 in]
              n408 = call "myRIO_BRig_RT_dataMTrig_Solenoid_c__L.vi"() -> ("output_Solenoid_c__L"=w756:i32)  [unwired: 11 in]
              n409 = call "myRIO_BRig_RT_dataMTrig_Solenoid_Tcycle__L.vi"() -> ("output_Solenoid_Tcycle__L"=w765:i32)  [unwired: 11 in]
              n410 = Index Array(array=w758, index #1=w756, index #2=w765, index #3=w764, index #4=w747, index #5=w749, index #6=w748) -> (element #1=w763:u16, element #2=w753:u16, element #3=w761:u16, element #4=w743:u16, element #5=w740:u16, element #6=w739:u16)
              n411 = Add(x=w763, y=w744) -> (x+y=w754:u16)
              n412 = Add(x=w743, y=w744) -> (x+y=w745:u16)
              n413 = Less?(x=w754, y=w753) -> (x < y?=w737:bool)
              n414 = Equal To 0?(x=w761) -> (x = 0?=w760:bool)
              n415 = Less?(x=w745, y=w740) -> (x < y?=w738:bool)
              n416 = Equal To 0?(x=w739) -> (x = 0?=w746:bool)
              n417 = And(x=w737, y=w760) -> (x .and. y?=w759:bool)
              n418 = Or(x=w737, y=w738) -> (x .or. y?=w736:bool)
              n419 = And(x=w738, y=w746) -> (x .and. y?=w741:bool)
              n420 = Select(t=w754, s=w737, f=w753) -> (s? t:f=w755:u16)
              n421 = Select(t=w745, s=w738, f=w740) -> (s? t:f=w742:u16)
              n422 = Replace Array Subset(array=w758, new element #1=w755, index #1=w756, new element #2=w742, index #2=w747) -> (w757:u16[])
              n423 = Select(t=w752, s=w736, f=myRIO_BRig_RT__Case_NonExp_stateList."DispenseWater_post" ("Enum")) -> (s? t:f=w750:T1)
            }
            frame "DispenseWater_post" {
              # "nCycle"
              # "delay"
              # "Solenoid__R"
              # "nCycle"
              # "delay"
              # "Solenoid__L"
              n424 = call "myRIO_BRig_RT_dataMTrig_Solenoid_N__L.vi"() -> ("output_Solenoid_N__L"=w787:i32)  [unwired: 11 in]
              n425 = call "myRIO_BRig_RT_dataMTrig_Solenoid_delay__L.vi"() -> ("output_Solenoid_delay__L"=w786:i32)  [unwired: 11 in]
              n426 = call "myRIO_BRig_RT_dataMTrig_Solenoid_N__R.vi"() -> ("output_Solenoid_N__R"=w783:i32)  [unwired: 11 in]
              n427 = call "myRIO_BRig_RT_dataMTrig_Solenoid_delay__R.vi"() -> ("output_Solenoid_delay__R"=w782:i32)  [unwired: 11 in]
              n428 = Index Array(array=w789, index #1=w787, index #2=w786, index #3=w783, index #4=w782) -> (element #1=w791:u16, element #2=w790:u16, element #3=w774:u16, element #4=w776:u16)
              n429 = Not Equal To 0?(x=w791) -> (x != 0?=w792:bool)
              n430 = Not Equal To 0?(x=w774) -> (x != 0?=w775:bool)
              n431 = case shown="True" w775 {
                selector: w775 -> [_ w800]
                tunnel: w774 -> [w798 w806]
                tunnel: w776 -> [_ w807]
                tunnel: [w798 w804] -> w773
                tunnel: [u16 0 w803] -> w772
                tunnel: [_ w800] -> w771
                frame False {
                }
                frame True {
                  n432 = Equal To 0?(x=w807) -> (x = 0?=w799:bool)
                  n433 = Decrement(x=w806) -> (x-1=w805:u16)
                  n434 = Select(t=w805, s=w799, f=w806) -> (s? t:f=w804:u16)
                  n435 = Select(t=u16 1, s=w799, f=u16 0) -> (s? t:f=w803:u16)
                }
              }
              n436 = case shown="True" w792 {
                selector: w792 -> [_ w811]
                tunnel: w791 -> [w809 w817]
                tunnel: w790 -> [_ w818]
                tunnel: [w809 w815] -> w785
                tunnel: [u16 0 w814] -> w784
                tunnel: [_ w811] -> w781
                frame False {
                }
                frame True {
                  n437 = Equal To 0?(x=w818) -> (x = 0?=w810:bool)
                  n438 = Decrement(x=w817) -> (x-1=w816:u16)
                  n439 = Select(t=w816, s=w810, f=w817) -> (s? t:f=w815:u16)
                  n440 = Select(t=u16 1, s=w810, f=u16 0) -> (s? t:f=w814:u16)
                }
              }
              n441 = Or(x=w781, y=w771) -> (x .or. y?=w780:bool)
              n442 = Replace Array Subset(array=w789, new element #1=w785, index #1=w787, new element #2=w784, index #2=w786, new element #3=w773, index #3=w783, new element #4=w772, index #4=w782) -> (w788:u16[])
              n443 = Select(t=myRIO_BRig_RT__Case_NonExp_stateList."DispenseWater_pre" ("Enum"), s=w780, f=myRIO_BRig_RT__Case_NonExp_stateList."Idle" ("Enum")) -> (s? t:f=w777:T1)
            }
            frame "TestConnection" {
              n444 = local read "Host Password"() -> (w829:string)
              n445 = local read "Host UserName"() -> (w830:string)
              n446 = call "myRIO_BRig_RT_comm_webdav_testConnect.vi"("input_password"=w829, "input_username"=w830) -> ("output_Iconnected"=w827:bool)  [unwired: 9 in]
              n447 = Select(t="Connection accepted!" ("message"), s=w827, f="Error!") -> (s? t:f=w825:string)
              n448 = One Button Dialog(message=w825) -> ()  [unwired: 1 in, 1 out]
            }
            frame "SendData" {
              n449 = local read "Host Filename Prefix"() -> (w832:string)
              n450 = local read "Host Password"() -> (w833:string)
              n451 = local read "Host UserName"() -> (w834:string)
              n452 = call "myRIO_BRig_RT_comm_webdav_sendData_all.vi"("Host Filename Prefix"=w832, "Host Password"=w833, "Host UserName"=w834) -> ()  [unwired: 9 in]
            }
            frame "End" {
            }
          }
          n453 = local read "MTrig_Audio_trig__R"() -> (w81:bool)
          n454 = local read "MTrig_Audio_trig__L"() -> (w80:bool)
          n455 = local read "START"() -> (w76:bool)
          n456 = local read "STOP_abort"() -> (w75:bool)
          n457 = local read "MTrig_Laser_trig"() -> (w82:bool)
          n458 = call "myRIO_BRig_RT_dataMTrig_main__v2.vi"("input_dataMTrig"=w84, "input_Audio_trig_L"=w80, "input_Audio_trig_R"=w81, "input_Laser_trig"=w82) -> ("output_dataMTrig"=w83:u16[], "output_Audio_L"=w60:bool, "output_Audio_R"=w71:bool, "output_Laser"=w63:bool)  [unwired: 12 in]
          n459 = Or(x=w76, y=w75) -> (x .or. y?=w74:bool)
          n460 = local read "A6"() -> (w53:bool)
          n461 = Select(t=myRIO_BRig_RT__Case_NonExp_stateList."End" ("Enum"), s=w74, f=w73) -> (s? t:f=w72:T1)
          n462 = Or(x=w81, y=w82) -> (x .or. y?=w79:bool)
          n463 = Or(x=w79, y=w80) -> (x .or. y?=w78:bool)
          n464 = case shown="True" w78 {
            frame False {
            }
            frame True {
              w109 = FALSE
              n465 = local write "MTrig_Audio_trig__R"(w109) -> ()
              n466 = local write "MTrig_Audio_trig__L"(w109) -> ()
              n467 = local write "MTrig_Laser_trig"(w109) -> ()
            }
          }
          n468 = xnode "Read/Write Control"("FPGA VI Reference In"=w101, "error in"=w99, "A6_Act"=w53, "A1_SR"=w85, "A3_SL"=w86, "audioTrigger_L"=w60, "audioAmp_L"=w90, "audioFreq_L_Hz"=w89, "audioTrigger_R"=w71, "audioAmp_R"=w88, "audioFreq_R_Hz"=w87, "laserResponse_reward_LED"="laserResponse_reward_LED", "laserResponse_wrong_LED"="laserResponse_wrong_LED", "laserResponse_reward"="laserResponse_reward", "laserResponse_wrong"="laserResponse_wrong", "SelectionState"="SelectionState", "ignoreWrong"="ignoreWrong", "Left(F)_or_Right(T)"="Left(F)_or_Right(T)", "laserMTrig"=w63, "tCycle_laser_rew"="tCycle_laser_rew", "tDelay_laser_rew"="tDelay_laser_rew", "tCycle_laser_wro"="tCycle_laser_wro", "tDelay_laser_wro"="tDelay_laser_wro") -> ("FPGA VI Reference Out"=w100:refnum<k20>, "error out"=w98:errorcluster, "SelectReward"=→"SelectReward":bool, "SelectWrong"=→"SelectWrong":bool)
          n469 = node-c288() -> ()  [unwired: 1 in, 1 out]
          "cState_NonExp" <- w97
        }
        n470 = node-c288(w48) -> ()  [unwired: 1 out]
        n471 = flat-sequence {
          tunnel: w41 -> [w52]
          tunnel: [w52] -> w40
          tunnel: w39 -> [w51]
          tunnel: [w51] -> w38
          frame #0 {
            w50 = FALSE
            n472 = local write "STOP_endBlock"(w50) -> ()
            n473 = local write "STOP_endTrial"(w50) -> ()
          }
        }
      }
      frame True {
        w856 = FALSE ("SelectionState")
        w861 = u16 0 ("idxDataBlock")
        w863 = u16 100 ("new element/subarray")
        w864 = u16 100 ("new element/subarray")
        w884 = T6 refnum items=["Session NI_WebDAV"] ("output_hSession")
        w893 = FALSE
        w894 = u16 0
        w855 = FALSE
        # "audio__L\naudio__R"
        # "Audio params"
        # "nRewards"
        # "idxDataBlock"
        # "Solenoid_Tdelay_R"
        # "Solenoid_Tdelay_L"
        # "RewCalib_N__R"
        # "RewCalib_N__L"
        # "Save dataLick to file\nSend file to Host\nSave dataMTrig\nSend file to Host\nDisconnect"
        # "dataTrial"
        # "dataTrial"
        # "Solenoid_Tcycle_R"
        # "Solenoid_Tcycle_L"
        # "Laser_Tcycle"
        # "Audio_Tcycle_R"
        # "Audio_Tcycle_L"
        # "dataLick"
        # "dataLC"
        # "dataLC"
        # "dataBlock"
        # "dataBlock"
        # "dataMTrig"
        # "dataMTrig"
        # "dataExp"
        # "dataCurrent"
        # "dataExp"
        # "dataCurrent"
        # "spout"
        # "state"
        n474 = call "myRIO_BRig_RT_dataMTrig_Solenoid_Tcycle__L.vi"() -> ("output_Solenoid_Tcycle__L"=w890:i32)  [unwired: 11 in]
        n475 = call "myRIO_BRig_RT_dataMTrig_Solenoid_Tcycle__R.vi"() -> ("output_Solenoid_Tcycle__R"=w889:i32)  [unwired: 11 in]
        n476 = call "myRIO_BRig_RT_dataMTrig_Audio_Tcycle__L.vi"() -> ("output_Audio_Tcycle__L"=w888:i32)  [unwired: 11 in]
        n477 = call "myRIO_BRig_RT_dataMTrig_Audio_Tcycle__R.vi"() -> ("output_Audio_Tcycle__R"=w887:i32)  [unwired: 11 in]
        n478 = call "myRIO_BRig_RT_dataMTrig_Laser_Tcycle.vi"() -> ("output_Laser_Tcycle"=w886:i32)  [unwired: 11 in]
        n479 = local read "MTrig_Solenoid_Tcycle__L"() -> (w869:u16)
        n480 = local read "MTrig_Solenoid_Tcycle__R"() -> (w868:u16)
        n481 = local read "Tcycle_Reward_L"() -> (w865:u16)
        n482 = local read "Tcycle_Reward_R"() -> (w866:u16)
        n483 = local read "MTrig_Laser_Tcycle"() -> (w867:u16)
        n484 = call "myRIO_BRig_RT_dataMTrig_Solenoid_RewCalib_nCycle__L.vi"() -> ("output_Solenoid_RewCalib_nCycle__L"=w872:i32)  [unwired: 11 in]
        n485 = call "myRIO_BRig_RT_dataMTrig_Solenoid_Tdelay__L.vi"() -> ("output_Solenoid_Tdelay__L"=w874:i32)  [unwired: 11 in]
        n486 = call "myRIO_BRig_RT_dataMTrig_Solenoid_RewCalib_nCycle__R.vi"() -> ("output_Solenoid_RewCalib_nCycle__R"=w873:i32)  [unwired: 11 in]
        n487 = call "myRIO_BRig_RT_dataMTrig_Solenoid_Tdelay__R.vi"() -> ("output_Solenoid_Tdelay__R"=w875:i32)  [unwired: 11 in]
        n488 = call "myRIO_BRig_RT_dataLick_init.vi"() -> ("output_dataLick"=w896:u16[][])  [unwired: 11 in]
        n489 = call "myRIO_BRig_RT_dataCurrent_init.vi"() -> ("output_dataCurrent"=w903:u16[])  [unwired: 11 in]
        n490 = call "myRIO_BRig_RT_dataExp_init.vi"() -> ("output_dataExp"=w902:u16[])  [unwired: 11 in]
        n491 = call "myRIO_BRig_RT_dataMTrig_init.vi"() -> ("output_dataMTrig"=w892:u16[])  [unwired: 5 in]
        n492 = call "myRIO_BRig_RT_dataLC_init.vi"() -> ("output_dataLC"=w900:u16[])  [unwired: 11 in]
        n493 = call "myRIO_BRig_RT_dataBlock_init.vi"() -> ("output_dataBlock"=w901:u16[][])  [unwired: 11 in]
        n494 = call "myRIO_BRig_RT_dataTrial_init.vi"() -> ("output_dataTrial"=w885:u16[][])  [unwired: 11 in]
        n495 = xnode "Read/Write Control"("FPGA VI Reference In"=w857, "error in"=w858, "SelectionState"=w856, "laserResponse_reward"=w856, "laserResponse_wrong"=w856, "laserResponse_reward_LED"=w856, "laserResponse_wrong_LED"=w856, "Left(F)_or_Right(T)"=w856, "ignoreWrong"=w856, "SelectionState"=w856) -> ("FPGA VI Reference Out"=w859:refnum<k20>, "error out"=w860:errorcluster)
        n496 = Replace Array Subset(array=w892, new element #1=w864, index #1=w872, new element #2=w864, index #2=w873, new element #3=w863, index #3=w874, new element #4=w863, index #4=w875, new element #5=w869, index #5=w890, new element #6=w868, index #6=w889, new element #7=w865, index #7=w888, new element #8=w866, index #8=w887, new element #9=w867, index #9=w886) -> (w891:u16[])
        n497 = Get Date/Time In Seconds() -> (seconds since 1Jan1904=w871:timestamp)
        n498 = To Double Precision Float(number=w871) -> (double precision float=w870:dbl)
        n499 = node-c288() -> (w911:T3)  [unwired: 4 in]
        n500 = timed-loop {
          timing: w911 -> [_]
          timing-out: [_] -> w910
          shift-right: [w989] -> _
          shift-left: myRIO_BRig_RT__Case_Exp_stateList."Start1" ("Enum") -> [w1020]
          shift-right: [w1041] -> _
          shift-left: enum16{"Left", "Right"}."Left" -> [w1043]
          tunnel: w859 -> [w1040]
          tunnel: w860 -> [w1039]
          shift-right: [w1034] -> _
          shift-left: w908 -> [w1038]
          shift-right: [w1033] -> _
          shift-left: w907 -> [w1037]
          tunnel: [w1014] -> w905
          tunnel: [w1015] -> w906
          shift-right: [w1016] -> w876
          shift-left: w903 -> [w981]
          shift-right: [w1032] -> _
          shift-left: w902 -> [w976]
          shift-right: [w1003] -> w880
          shift-left: w891 -> [w1004]
          shift-right: [w1030] -> _
          shift-left: w901 -> [w1031]
          shift-right: [w1028] -> _
          shift-left: w900 -> [w1029]
          shift-right: [w961] -> _
          shift-left: w855 -> [w1027]
          shift-right: [w1018] -> w882
          shift-left: w896 -> [w1019]
          shift-right: [w1005] -> _
          shift-left: w894 -> [w1013]
          shift-right: [w973] -> _
          shift-left: w894 -> [w1012]
          shift-right: [w1006] -> _
          shift-left: w894 -> [w1011]
          shift-right: [w1007] -> _
          shift-left: w894 -> [w1010]
          shift-right: [w974] -> _
          shift-left: w893 -> [w1008]
          shift-right: [w975] -> _
          shift-left: w893 -> [w1009]
          shift-right: [w987] -> _
          shift-left: w885 -> [w988]
          shift-right: [w986] -> w878
          shift-left: w884 -> [w984]
          shift-right: [w985] -> w879
          shift-left: FALSE ("output_Iconnected") -> [w983]
          tunnel: "Host Filename Prefix" -> [w982]
          tunnel: [w982] -> w877
          shift-right: [w956] -> _
          shift-left: w855 -> [w980]
          tunnel: w870 -> [w977]
          shift-right: [w971] -> _
          shift-left: 0 ("idxDataBlock") -> [w972]
          shift-right: [w968] -> _
          shift-left: w861 -> [w970]
          shift-right: [w967] -> _
          shift-left: w861 -> [w969]
          shift-right: [w955] -> _
          shift-left: w855 -> [w962]
          shift-right: [w958] -> _
          shift-left: w855 -> [w960]
          shift-right: [w957] -> _
          shift-left: w855 -> [w959]
          shift-right: [w948] -> _
          shift-left: w855 -> [w949]
          stop <- w1026 stop-if-true
          # "Laser"
          # "Audio R"
          # "Audio L"
          # "Solenoid R"
          # "Solenoid L"
          # "manual triggering"
          # "dataTrial"
          # "dataBlock"
          # "nRewards"
          # "laserOccurred"
          # "dataExp"
          # "dataCurrent"
          # "audio__L\naudio__R"
          # "time stamp"
          # "Audio params"
          # "nRewards"
          # "idxDataBlock"
          # "idxDataBlock"
          # "activate"
          # "audio__L\naudio__R"
          # "amp__R\nfreq__R"
          # "amp__L\nfreq__L"
          # "dataLC"
          # "solenoid__R"
          # "solenoid__L"
          # "Did a lick occur?"
          # "Update lick counter"
          # "spout"
          # "spout"
          # "state"
          # "state"
          n501 = node-c288() -> ()  [unwired: 1 in, 1 out]
          n502 = local read "MTrig_Solenoid_trig__L"() -> (w1001:bool)
          n503 = local read "MTrig_Solenoid_trig__R"() -> (w1000:bool)
          n504 = local read "MTrig_Audio_trig__L"() -> (w999:bool)
          n505 = local read "MTrig_Audio_trig__R"() -> (w998:bool)
          n506 = xnode "Read/Write Control"("FPGA VI Reference In"=w1040, "error in"=w1039) -> ("FPGA VI Reference Out"=w966:refnum<k20>, "error out"=w965:errorcluster, "A2_LickL"=w1034:u32, "A4_LickR"=w1033:u32)
          "A2" <- w1034
          "A4" <- w1033
          n507 = local read "MTrig_Laser_trig"() -> (w997:bool)
          n508 = Greater?(x=w1034, y=w1038) -> (0:w1036:bool)
          n509 = Greater?(x=w1033, y=w1037) -> (0:w1035:bool)
          n510 = Or(x=w1036, y=w1035) -> (x .or. y?=w1042:bool)
          n511 = call "myRIO_BRig_RT_dataMTrig_main.vi"("input_dataMTrig"=w1004, "input_Solenoid_trig_L"=w1001, "input_Solenoid_trig_R"=w1000, "input_Audio_trig_L"=w999, "input_Audio_trig_R"=w998, "input_Laser_trig"=w997) -> ("output_Laser"=w953:bool, "output_dataMTrig"=w1003:u16[], "output_Solenoid_L"=w991:bool, "output_Solenoid_R"=w993:bool, "output_Audio_L"=w995:bool, "output_Audio_R"=w996:bool)  [unwired: 8 in]
          n512 = Compound Arithmetic op=OR(w1001, w1000, w999, w998, w997) -> (w1002:bool)
          n513 = case shown="True" w1002 {
            frame False {
            }
            frame True {
              w1044 = FALSE
              n514 = local write "MTrig_Solenoid_trig__L"(w1044) -> ()
              n515 = local write "MTrig_Solenoid_trig__R"(w1044) -> ()
              n516 = local write "MTrig_Audio_trig__L"(w1044) -> ()
              n517 = local write "MTrig_Audio_trig__R"(w1044) -> ()
              n518 = local write "MTrig_Laser_trig"(w1044) -> ()
            }
          }
          n519 = case shown="\"initBlock2\"" w1020 {
            selector: w1020 -> [_ _ _ _ _ _ _ _ _ _ _ _ _ _ _ _ _ w1588 _ w1656 _ _ _ _ _ w1794 _ w1870 _ _ _ _ _ w2002 _ w2079 _ w2143 _ w2187 _ _ w2254 _ _ _ _ _ w2422 _ _ _ _ _ _ _ _ _ _ _ _]
            tunnel: [myRIO_BRig_RT__Case_Exp_stateList."Start2" ("Enum") myRIO_BRig_RT__Case_Exp_stateList."Start3" ("Enum") myRIO_BRig_RT__Case_Exp_stateList."saveSettings1" ("Enum") myRIO_BRig_RT__Case_Exp_stateList."saveSettings2" ("Enum") myRIO_BRig_RT__Case_Exp_stateList."saveSettings3" ("Enum") myRIO_BRig_RT__Case_Exp_stateList."saveSettings4_LC_ENL" ("Enum") myRIO_BRig_RT__Case_Exp_stateList."saveSettings5_LC_Cue" ("Enum") myRIO_BRig_RT__Case_Exp_stateList."saveSettings6_LC_Other" ("Enum") myRIO_BRig_RT__Case_Exp_stateList."setSettings_Audio" ("Enum") myRIO_BRig_RT__Case_Exp_stateList."commConnect" ("Enum") w1408 myRIO_BRig_RT__Case_Exp_stateList."initTrial" ("Enum") w1448 myRIO_BRig_RT__Case_Exp_stateList."initTrial3" ("Enum") myRIO_BRig_RT__Case_Exp_stateList."initTrial4" ("Enum") myRIO_BRig_RT__Case_Exp_stateList."ENL1_pre" ("Enum") w1547 w1585 myRIO_BRig_RT__Case_Exp_stateList."ENL1Penalty" ("Enum") w1657 myRIO_BRig_RT__Case_Exp_stateList."endExp" ("Enum") myRIO_BRig_RT__Case_Exp_stateList."endExp" ("Enum") myRIO_BRig_RT__Case_Exp_stateList."endExp" ("Enum") myRIO_BRig_RT__Case_Exp_stateList."endExp" ("Enum") w1750 w1793 myRIO_BRig_RT__Case_Exp_stateList."Cue1Penalty" ("Enum") w1868 myRIO_BRig_RT__Case_Exp_stateList."endExp" ("Enum") myRIO_BRig_RT__Case_Exp_stateList."endExp" ("Enum") myRIO_BRig_RT__Case_Exp_stateList."endExp" ("Enum") myRIO_BRig_RT__Case_Exp_stateList."endExp" ("Enum") w1956 w2010 myRIO_BRig_RT__Case_Exp_stateList."SelectReward" ("Enum") w2080 myRIO_BRig_RT__Case_Exp_stateList."SelectRewardPost" ("Enum") w2144 myRIO_BRig_RT__Case_Exp_stateList."SelectWrong" ("Enum") w2183 myRIO_BRig_RT__Case_Exp_stateList."endTrial1" ("Enum") myRIO_BRig_RT__Case_Exp_stateList."SelectTimeout" ("Enum") w2256 myRIO_BRig_RT__Case_Exp_stateList."endTrial1" ("Enum") myRIO_BRig_RT__Case_Exp_stateList."endTrial2" ("Enum") myRIO_BRig_RT__Case_Exp_stateList."saveData_dataBlock" ("Enum") w2335 w2405 w2422 myRIO_BRig_RT__Case_Exp_stateList."initBlock" ("Enum") w2449 myRIO_BRig_RT__Case_Exp_stateList."commUpload_dataCurrent" ("Enum") myRIO_BRig_RT__Case_Exp_stateList."commUpload_dataExp" ("Enum") myRIO_BRig_RT__Case_Exp_stateList."commUpload_dataLC" ("Enum") myRIO_BRig_RT__Case_Exp_stateList."commUpload_dataTrial" ("Enum") myRIO_BRig_RT__Case_Exp_stateList."endTrial3" ("Enum") myRIO_BRig_RT__Case_Exp_stateList."saveData_dataCurrent" ("Enum") myRIO_BRig_RT__Case_Exp_stateList."saveData_dataExp" ("Enum") myRIO_BRig_RT__Case_Exp_stateList."saveData_dataLC" ("Enum") myRIO_BRig_RT__Case_Exp_stateList."saveData_dataTrial" ("Enum") myRIO_BRig_RT__Case_Exp_stateList."commUpload_pre" ("Enum")] -> w989
            tunnel: [w1070 w1090 w1112 w1169 w1213 w1240 w1276 w1312 w1356 w1380 w1384 w1416 w1449 w1472 w1493 w1521 w1563 w1601 w1634 w1661 w1677 w1699 w1718 w1737 w1769 w1815 w1841 w1867 w1888 w1909 w1928 w1947 w1967 w2028 w2053 w2076 w2091 w2141 w2165 w2198 w2219 w2235 w2267 w2290 w2302 w2321 w2359 w2378 w2421 w2438 w2452 w2486 w2507 w2528 w2549 w2570 w2598 w2618 w2645 w2665 w2690] -> w1041
            tunnel: w1043 -> [w1070 w1090 w1112 w1169 w1213 w1240 w1276 w1312 w1356 w1380 w1407 w1416 w1449 w1472 w1493 w1521 w1563 w1601 w1634 w1661 w1677 w1699 w1718 w1737 w1769 w1815 w1841 w1867 w1888 w1909 w1928 w1947 w1967 w2028 w2053 w2076 w2091 w2141 w2165 w2198 w2219 w2235 w2267 w2290 w2302 w2321 w2359 w2378 w2421 w2438 w2452 w2486 w2507 w2528 w2549 w2570 w2598 w2618 w2645 w2665 w2690]
            tunnel: w1042 -> [w1073 w1093 w1109 w1172 w1216 w1243 w1279 w1315 w1359 w1383 w1401 w1427 w1450 w1490 w1510 w1535 w1550 w1582 w1637 w1664 w1683 w1702 w1721 w1740 w1749 w1792 w1849 w1874 w1893 w1912 w1931 w1950 w1965 w2026 w2063 w2087 w2122 w2149 w2176 w2201 w2218 w2247 w2272 w2287 w2310 w2320 w2370 w2404 w2425 w2435 w2461 w2489 w2510 w2531 w2552 w2573 w2601 w2621 w2648 w2668 w2693]
            tunnel: w1036 -> [w1072 w1092 w1110 w1171 w1215 w1242 w1278 w1314 w1358 w1382 w1400 w1426 w1451 w1489 w1511 w1536 w1573 w1603 w1636 w1663 w1682 w1701 w1720 w1739 w1783 w1816 w1848 w1873 w1892 w1911 w1930 w1949 w1966 w2025 w2062 w2086 w2121 w2148 w2175 w2200 w2217 w2246 w2271 w2288 w2311 w2319 w2369 w2403 w2424 w2436 w2462 w2488 w2509 w2530 w2551 w2572 w2600 w2620 w2647 w2667 w2692]
            tunnel: w1035 -> [w1071 w1091 w1111 w1170 w1214 w1241 w1277 w1313 w1357 w1381 w1399 w1425 w1452 w1488 w1512 w1537 w1572 w1602 w1635 w1662 w1681 w1700 w1719 w1738 w1782 w1817 w1847 w1872 w1891 w1910 w1929 w1948 w1985 w2029 w2061 w2085 w2120 w2147 w2174 w2199 w2216 w2245 w2270 w2289 w2312 w2318 w2368 w2402 w2423 w2437 w2463 w2487 w2508 w2529 w2550 w2571 w2599 w2619 w2646 w2666 w2691]
            tunnel: [w1073 w1093 w1109 w1172 w1216 w1243 w1279 w1315 w1359 w1383 w1401 w1427 w1450 w1490 w1510 w1535 w1550 w1582 w1637 w1664 w1683 w1702 w1721 w1740 w1749 w1792 w1849 w1874 w1893 w1912 w1931 w1950 w1965 w2026 w2063 w2087 w2122 w2149 w2176 w2201 w2218 w2247 w2272 w2287 w2310 w2320 w2370 w2404 w2425 w2435 w2461 w2489 w2510 w2531 w2552 w2573 w2601 w2621 w2648 w2668 w2693] -> w1023
            tunnel: [w1072 w1092 w1110 w1171 w1215 w1242 w1278 w1314 w1358 w1382 w1400 w1426 w1451 w1489 w1511 w1536 w1573 w1603 w1636 w1663 w1682 w1701 w1720 w1739 w1783 w1816 w1848 w1873 w1892 w1911 w1930 w1949 w1966 w2025 w2062 w2086 w2121 w2148 w2175 w2200 w2217 w2246 w2271 w2288 w2311 w2319 w2369 w2403 w2424 w2436 w2462 w2488 w2509 w2530 w2551 w2572 w2600 w2620 w2647 w2667 w2692] -> w1022
            tunnel: [w1071 w1091 w1111 w1170 w1214 w1241 w1277 w1313 w1357 w1381 w1399 w1425 w1452 w1488 w1512 w1537 w1572 w1602 w1635 w1662 w1681 w1700 w1719 w1738 w1782 w1817 w1847 w1872 w1891 w1910 w1929 w1948 w1985 w2029 w2061 w2085 w2120 w2147 w2174 w2199 w2216 w2245 w2270 w2289 w2312 w2318 w2368 w2402 w2423 w2437 w2463 w2487 w2508 w2529 w2550 w2571 w2599 w2619 w2646 w2666 w2691] -> w1021
            tunnel: w981 -> [w1069 w1089 w1108 w1130 w1189 w1239 w1275 w1311 w1355 w1378 w1406 w1415 w1447 w1461 w1494 w1516 w1562 w1587 w1628 w1660 w1678 w1698 w1717 w1736 w1753 w1812 w1840 w1871 w1889 w1908 w1927 w1946 w1976 w2006 w2045 w2082 w2093 w2146 w2166 w2197 w2215 w2236 w2269 w2286 w2299 w2323 w2339 w2376 w2420 w2439 w2464 w2483 w2504 w2525 w2546 w2557 w2587 w2606 w2630 w2662 w2679]
            tunnel: w976 -> [w1068 w1088 w1107 w1167 w1211 w1236 w1273 w1309 w1353 w1371 w1405 w1424 w1446 w1469 w1498 w1524 w1565 w1600 w1627 w1658 w1680 w1697 w1716 w1735 w1771 w1814 w1838 w1866 w1890 w1907 w1926 w1945 w1978 w2027 w2059 w2084 w2114 w2142 w2167 w2195 w2214 w2238 w2266 w2285 w2309 w2326 w2338 w2395 w2419 w2440 w2465 w2482 w2503 w2524 w2545 w2558 w2595 w2615 w2626 w2661 w2687]
            tunnel: [w1069 w1089 w1108 w1130 w1189 w1239 w1275 w1311 w1355 w1378 w1390 w1415 w1435 w1461 w1494 w1515 w1566 w1586 w1629 w1659 w1678 w1698 w1717 w1736 w1778 w1811 w1839 w1869 w1889 w1908 w1927 w1946 w1979 w2001 w2060 w2081 w2115 w2145 w2168 w2196 w2215 w2239 w2268 w2286 w2298 w2322 w2339 w2374 w2420 w2439 w2464 w2483 w2504 w2525 w2546 w2557 w2587 w2606 w2630 w2662 w2679] -> w1017
            tunnel: [w1068 w1088 w1107 w1166 w1210 w1231 w1273 w1309 w1353 w1371 w1404 w1424 w1445 w1469 w1498 w1524 w1565 w1600 w1627 w1658 w1680 w1697 w1716 w1735 w1771 w1814 w1838 w1866 w1890 w1907 w1926 w1945 w1978 w2027 w2059 w2084 w2114 w2142 w2167 w2195 w2214 w2238 w2266 w2285 w2309 w2326 w2338 w2395 w2419 w2440 w2465 w2482 w2503 w2524 w2545 w2558 w2595 w2615 w2629 w2661 w2687] -> w1032
            tunnel: [_ _ _ _ _ _ _ _ _ _ _ _ _ _ _ _ _ _ _ _ _ _ _ _ _ _ _ _ _ _ _ _ _ _ _ w2074 _ _ _ _ _ _ _ _ _ _ _ _ _ _ _ _ _ _ _ _ _ _ _ _ _] -> w992
            tunnel: [_ _ _ _ _ _ _ _ _ _ _ _ _ _ _ _ _ _ _ _ _ _ _ _ _ _ _ _ _ _ _ _ _ _ _ w2075 _ _ _ _ _ _ _ _ _ _ _ _ _ _ _ _ _ _ _ _ _ _ _ _ _] -> w994
            tunnel: w1031 -> [w1066 w1086 w1105 w1132 w1191 w1237 w1274 w1310 w1354 w1376 w1402 w1417 w1443 w1481 w1508 w1534 w1564 w1599 w1624 w1654 w1679 w1695 w1714 w1733 w1777 w1813 w1837 w1864 w1886 w1905 w1924 w1943 w1977 w2023 w2051 w2083 w2095 w2139 w2164 w2192 w2212 w2237 w2265 w2283 w2301 w2328 w2366 w2387 w2417 w2442 w2467 w2480 w2501 w2522 w2543 w2567 w2581 w2608 w2636 w2655 w2681]
            tunnel: [w1066 w1086 w1105 w1132 w1191 w1237 w1274 w1310 w1354 w1376 w1402 w1414 w1443 w1481 w1508 w1534 w1564 w1599 w1624 w1654 w1679 w1695 w1714 w1733 w1777 w1813 w1837 w1864 w1886 w1905 w1924 w1943 w1977 w2023 w2051 w2083 w2094 w2139 w2164 w2192 w2212 w2237 w2265 w2283 w2300 w2328 w2366 w2387 w2417 w2442 w2467 w2480 w2501 w2522 w2543 w2567 w2581 w2608 w2636 w2655 w2681] -> w1030
            tunnel: w1029 -> [w1067 w1087 w1106 w1131 w1190 w1238 w1271 w1307 w1351 w1377 w1403 w1423 w1444 w1458 w1509 w1522 w1561 w1581 w1625 w1655 w1676 w1696 w1715 w1734 w1776 w1791 w1836 w1865 w1887 w1906 w1925 w1944 w1975 w2024 w2052 w2078 w2112 w2140 w2163 w2194 w2213 w2234 w2263 w2284 w2308 w2327 w2367 w2394 w2418 w2441 w2466 w2481 w2502 w2523 w2544 w2568 w2594 w2614 w2642 w2653 w2686]
            tunnel: [w1067 w1087 w1106 w1131 w1190 w1238 w1272 w1308 w1352 w1377 w1403 w1423 w1444 w1458 w1509 w1522 w1561 w1581 w1625 w1655 w1676 w1696 w1715 w1734 w1776 w1791 w1836 w1865 w1887 w1906 w1925 w1944 w1975 w2024 w2052 w2078 w2112 w2140 w2163 w2194 w2213 w2234 w2263 w2284 w2308 w2327 w2367 w2394 w2418 w2441 w2466 w2481 w2502 w2523 w2544 w2568 w2594 w2614 w2642 w2653 w2686] -> w1028
            tunnel: w1027 -> [_ _ _ _ _ _ _ _ _ _ _ _ _ _ _ _ w1546 w1580 w1609 w1643 _ _ _ _ _ w1784 w1818 w1852 _ _ _ _ _ _ _ w2077 _ _ _ w2193 _ _ w2264 _ _ _ _ _ _ _ _ _ _ _ _ _ _ _ _ _ _]
            tunnel: [_ _ _ _ _ _ _ _ _ _ _ _ _ _ _ _ _ _ _ _ _ _ _ _ _ _ _ _ _ _ _ _ _ _ _ _ _ _ _ _ _ _ _ _ _ _ _ _ TRUE _ _ _ _ _ _ _ _ _ _ _ _] -> w1024
            tunnel: w1013 -> [w1064 w1084 w1103 w1122 w1184 w1226 w1258 w1294 w1323 _ w1398 w1422 w1442 w1480 w1507 w1533 w1560 w1598 w1622 w1653 w1674 w1693 w1712 w1731 w1775 w1808 w1834 w1863 w1884 w1903 w1922 w1941 w1974 w2022 w2041 w2073 w2110 w2138 w2161 w2191 w2211 w2232 w2262 w2282 w2306 w2332 w2365 w2391 w2415 w2433 w2460 w2478 w2499 w2520 w2541 w2565 w2592 w2612 w2640 w2659 w2685]
            tunnel: w1012 -> [w1063 w1083 w1102 w1121 w1183 w1225 w1257 w1293 w1324 _ w1397 w1421 w1441 w1479 w1506 w1532 w1559 w1597 w1621 w1652 w1673 w1692 w1711 w1730 w1774 w1807 w1833 w1862 w1883 w1902 w1921 w1940 w1973 w2021 w2040 w2072 w2109 w2137 w2160 w2190 w2210 w2231 w2261 w2281 w2305 w2331 w2364 w2390 w2414 w2432 w2459 w2477 w2498 w2519 w2540 w2564 w2591 w2611 w2639 w2658 w2684]
            tunnel: w1011 -> [w1062 w1082 w1101 w1120 w1182 w1224 w1256 w1292 w1325 _ w1396 w1420 w1440 w1478 w1505 w1531 w1558 w1596 w1620 w1651 w1672 w1691 w1710 w1729 w1773 w1806 w1832 w1861 w1882 w1901 w1920 w1939 w1972 w2020 w2039 w2071 w2108 w2136 w2159 w2189 w2209 w2230 w2260 w2280 w2304 w2330 w2363 w2389 w2413 w2431 w2458 w2476 w2497 w2518 w2539 w2563 w2590 w2610 w2638 w2657 w2683]
            tunnel: w1010 -> [w1061 w1081 w1100 w1119 w1181 w1223 w1255 w1291 w1326 _ w1395 w1419 w1439 w1477 w1504 w1530 w1557 w1595 w1619 w1650 w1671 w1690 w1709 w1728 w1772 w1805 w1831 w1860 w1881 w1900 w1919 w1938 w1971 w2019 w2038 w2070 w2107 w2135 w2158 w2188 w2208 w2229 w2259 w2279 w2303 w2329 w2362 w2388 w2412 w2430 w2457 w2475 w2496 w2517 w2538 w2562 w2589 w2609 w2637 w2656 w2682]
            tunnel: w1009 -> [_ _ _ _ _ _ _ _ _ _ _ _ _ _ _ _ _ _ _ _ _ _ _ _ _ w1810 _ _ _ _ _ _ _ _ _ _ _ _ _ _ _ _ _ _ _ _ _ _ _ _ _ _ _ _ _ _ _ _ _ _ _]
            tunnel: w1008 -> [_ _ _ _ _ _ _ _ _ _ _ _ _ _ _ _ _ _ _ _ _ _ _ _ _ w1809 _ _ _ _ _ _ _ _ _ _ _ _ _ _ _ _ _ _ _ _ _ _ _ _ _ _ _ _ _ _ _ _ _ _ _]
            tunnel: [w1064 w1084 w1103 w1122 w1184 w1226 w1258 w1294 w1323 w1370 w1398 w1422 w1442 w1480 w1507 w1533 w1560 w1598 w1622 w1653 w1674 w1693 w1712 w1731 w1775 w1808 w1834 w1863 w1884 w1903 w1922 w1941 w1974 w2022 w2041 w2073 w2110 w2138 w2161 w2191 w2211 w2232 w2262 w2282 w2306 w2332 w2365 w2391 w2415 w2433 w2460 w2478 w2499 w2520 w2541 w2565 w2592 w2612 w2640 w2659 w2685] -> w1005
            tunnel: [w1063 w1083 w1102 w1121 w1183 w1225 w1257 w1293 w1324 w1369 w1397 w1421 w1441 w1479 w1506 w1532 w1559 w1597 w1621 w1652 w1673 w1692 w1711 w1730 w1774 w1807 w1833 w1862 w1883 w1902 w1921 w1940 w1973 w2021 w2040 w2072 w2109 w2137 w2160 w2190 w2210 w2231 w2261 w2281 w2305 w2331 w2364 w2390 w2414 w2432 w2459 w2477 w2498 w2519 w2540 w2564 w2591 w2611 w2639 w2658 w2684] -> w973
            tunnel: [w1062 w1082 w1101 w1120 w1182 w1224 w1256 w1292 w1325 w1368 w1396 w1420 w1440 w1478 w1505 w1531 w1558 w1596 w1620 w1651 w1672 w1691 w1710 w1729 w1773 w1806 w1832 w1861 w1882 w1901 w1920 w1939 w1972 w2020 w2039 w2071 w2108 w2136 w2159 w2189 w2209 w2230 w2260 w2280 w2304 w2330 w2363 w2389 w2413 w2431 w2458 w2476 w2497 w2518 w2539 w2563 w2590 w2610 w2638 w2657 w2683] -> w1006
            tunnel: [w1061 w1081 w1100 w1119 w1181 w1223 w1255 w1291 w1326 w1367 w1395 w1419 w1439 w1477 w1504 w1530 w1557 w1595 w1619 w1650 w1671 w1690 w1709 w1728 w1772 w1805 w1831 w1860 w1881 w1900 w1919 w1938 w1971 w2019 w2038 w2070 w2107 w2135 w2158 w2188 w2208 w2229 w2259 w2279 w2303 w2329 w2362 w2388 w2412 w2430 w2457 w2475 w2496 w2517 w2538 w2562 w2589 w2609 w2637 w2656 w2682] -> w1007
            tunnel: [_ _ _ _ _ _ _ _ _ _ _ _ _ _ _ _ _ _ _ _ _ _ _ _ w1762 w1810 _ _ _ _ _ _ _ _ _ _ _ _ _ _ _ _ _ _ _ _ _ _ _ _ _ _ _ _ _ _ _ _ _ _ _] -> w975
            tunnel: [_ _ _ _ _ _ _ _ _ _ _ _ _ _ _ _ _ _ _ _ _ _ _ _ w1761 w1809 _ _ _ _ _ _ _ _ _ _ _ _ _ _ _ _ _ _ _ _ _ _ _ _ _ _ _ _ _ _ _ _ _ _ _] -> w974
            tunnel: w988 -> [w1060 w1080 w1099 w1118 w1180 w1222 w1254 w1290 w1322 w1366 w1394 w1418 w1438 w1463 w1496 w1514 w1556 w1594 w1618 w1649 w1670 w1689 w1708 w1727 w1760 w1804 w1830 w1859 w1880 w1899 w1918 w1937 w1970 w2018 w2035 w2069 w2106 w2134 w2155 w2182 w2207 w2226 w2253 w2278 w2297 w2325 w2355 w2386 w2411 w2443 w2468 w2479 w2500 w2521 w2542 w2566 w2593 w2613 w2641 w2660 w2676]
            tunnel: [w1060 w1080 w1099 w1118 w1180 w1222 w1254 w1290 w1322 w1366 w1394 w1418 w1438 w1462 w1495 w1513 w1556 w1594 w1618 w1649 w1670 w1689 w1708 w1727 w1760 w1804 w1830 w1859 w1880 w1899 w1918 w1937 w1970 w2018 w2035 w2069 w2106 w2134 w2155 w2182 w2207 w2226 w2253 w2278 w2297 w2324 w2355 w2386 w2411 w2443 w2468 w2479 w2500 w2521 w2542 w2566 w2593 w2613 w2641 w2660 w2676] -> w987
            tunnel: [w1059 w1079 w1098 w1117 w1179 w1221 w1253 w1289 w1321 w1365 w1393 w1429 w1437 w1483 w1503 w1529 w1555 w1593 w1617 w1648 w1669 w1688 w1707 w1726 w1759 w1803 w1829 w1858 w1879 w1898 w1917 w1936 w1969 w2017 w2034 w2068 w2105 w2133 w2154 w2181 w2206 w2225 w2252 w2277 w2296 w2317 w2361 w2385 w2409 w2444 w2454 w2474 w2495 w2516 w2537 w2561 w2597 w2617 w2644 w2664 w2689] -> w986
            tunnel: [w1058 w1078 w1097 w1116 w1178 w1220 w1252 w1288 w1320 w1364 w1392 w1428 w1436 w1482 w1502 w1528 w1554 w1592 w1616 w1647 w1668 w1687 w1706 w1725 w1758 w1802 w1828 w1857 w1878 w1897 w1916 w1935 w1968 w2016 w2033 w2067 w2104 w2132 w2153 w2180 w2205 w2224 w2251 w2276 w2295 w2316 w2360 w2384 w2410 w2426 w2451 w2484 w2505 w2526 w2547 w2569 w2596 w2616 w2643 w2663 w2688] -> w985
            tunnel: w984 -> [w1059 w1079 w1098 w1117 w1179 w1221 w1253 w1289 w1321 w1365 w1393 w1429 w1437 w1483 w1503 w1529 w1555 w1593 w1617 w1648 w1669 w1688 w1707 w1726 w1759 w1803 w1829 w1858 w1879 w1898 w1917 w1936 w1969 w2017 w2034 w2068 w2105 w2133 w2154 w2181 w2206 w2225 w2252 w2277 w2296 w2317 w2361 w2385 w2409 _ w2454 w2474 w2495 w2516 w2537 w2561 w2597 w2617 w2644 w2664 w2689]
            tunnel: w983 -> [w1058 w1078 w1097 w1116 w1178 w1220 w1252 w1288 w1320 w1364 w1392 w1428 w1436 w1482 w1502 w1528 w1554 w1592 w1616 w1647 w1668 w1687 w1706 w1725 w1758 w1802 w1828 w1857 w1878 w1897 w1916 w1935 w1968 w2016 w2033 w2067 w2104 w2132 w2153 w2180 w2205 w2224 w2251 w2276 w2295 w2316 w2360 w2384 w2410 _ w2451 w2484 w2505 w2526 w2547 w2569 w2596 w2616 w2643 w2663 w2688]
            tunnel: w982 -> [_ _ _ _ _ _ _ _ _ _ _ _ _ _ _ _ _ _ _ _ _ _ _ _ _ _ _ _ _ _ _ _ _ _ _ _ _ _ _ _ _ _ _ _ _ _ _ _ _ _ _ w2472 w2493 w2514 w2535 w2559 _ _ _ _ _]
            tunnel: w980 -> [_ _ _ _ _ _ _ _ _ _ _ _ _ _ _ _ w1543 w1578 w1610 w1639 _ _ _ _ _ _ _ _ _ _ _ _ _ _ _ _ _ _ _ _ _ _ _ _ _ _ _ _ _ _ _ _ _ _ _ _ _ _ _ _ _]
            tunnel: [_ "A6" _ _ _ _ _ _ _ _ _ _ _ _ _ _ _ _ _ _ _ _ _ _ _ _ _ _ _ _ _ _ _ _ _ _ _ _ _ _ _ _ _ _ _ _ _ _ _ _ _ _ _ _ _ _ _ _ _ _ _] -> w963
            tunnel: w977 -> [_ _ _ _ _ _ _ _ _ _ _ _ _ _ _ _ _ _ _ _ _ _ _ _ _ _ _ _ _ _ _ _ _ _ _ _ _ _ _ _ _ _ _ _ _ _ _ _ _ _ _ _ _ _ _ _ _ _ w2631 _ _]
            tunnel: [w1057 w1076 w1096 w1115 w1177 w1219 w1251 w1287 w1319 w1363 w1387 w1412 w1432 w1484 w1501 w1527 w1553 w1591 w1615 w1646 w1667 w1686 w1705 w1724 w1757 w1801 w1827 w1856 w1877 w1896 w1915 w1934 w1964 w2015 w2032 w2066 w2089 w2131 w2152 w2179 w2204 w2223 w2250 w2275 w2294 w2315 w2358 w2371 w2408 w2429 w2453 w2471 w2492 w2513 w2534 w2556 w2576 w2605 w2625 w2652 w2672] -> w971
            tunnel: w972 -> [w1057 w1076 w1096 w1115 w1177 w1219 w1251 w1287 w1319 w1363 w1387 _ w1432 w1484 w1501 w1527 w1553 w1591 w1615 w1646 w1667 w1686 w1705 w1724 w1757 w1801 w1827 w1856 w1877 w1896 w1915 w1934 w1964 w2015 w2032 w2066 w2089 w2131 w2152 w2179 w2204 w2223 w2250 w2275 w2294 w2315 w2358 w2372 w2408 w2429 w2453 w2471 w2492 w2513 w2534 w2556 w2576 w2605 w2625 w2652 w2672]
            tunnel: w970 -> [w1056 w1075 w1095 w1114 w1176 w1218 w1250 w1286 w1318 w1362 w1386 w1411 w1431 w1476 w1500 w1526 w1552 w1590 w1614 w1645 w1666 w1685 w1704 w1723 w1756 w1800 w1826 w1855 w1876 w1895 w1914 w1933 w1963 w2014 w2031 w2065 w2103 w2130 w2151 w2178 w2203 w2222 w2249 w2274 w2293 w2314 w2357 w2383 w2407 w2428 w2456 w2470 w2491 w2512 w2533 w2555 w2575 w2604 w2624 w2651 w2671]
            tunnel: w969 -> [w1055 w1074 w1094 w1113 w1175 w1217 w1249 w1285 w1317 w1361 w1385 w1410 w1430 w1475 w1499 w1525 w1551 w1589 w1613 w1644 w1665 w1684 w1703 w1722 w1755 w1799 w1825 w1854 w1875 w1894 w1913 w1932 w1962 w2013 w2030 w2064 w2100 w2129 w2150 w2177 w2202 w2221 w2248 w2273 w2292 w2313 w2356 w2382 w2406 w2427 w2455 w2469 w2490 w2511 w2532 w2554 w2574 w2603 w2623 w2650 w2670]
            tunnel: [w1056 w1075 w1095 w1114 w1176 w1218 w1250 w1286 w1318 w1362 w1386 w1411 w1431 w1476 w1500 w1526 w1552 w1590 w1614 w1645 w1666 w1685 w1704 w1723 w1756 w1800 w1826 w1855 w1876 w1895 w1914 w1933 w1963 w2014 w2031 w2065 w2102 w2130 w2151 w2178 w2203 w2222 w2249 w2274 w2293 w2314 w2357 w2383 w2407 w2428 w2456 w2470 w2491 w2512 w2533 w2555 w2575 w2604 w2624 w2651 w2671] -> w968
            tunnel: [w1055 w1074 w1094 w1113 w1175 w1217 w1249 w1285 w1317 w1361 w1385 w1410 w1430 w1475 w1499 w1525 w1551 w1589 w1613 w1644 w1665 w1684 w1703 w1722 w1755 w1799 w1825 w1854 w1875 w1894 w1913 w1932 w1962 w2013 w2030 w2064 w2101 w2129 w2150 w2177 w2202 w2221 w2248 w2273 w2292 w2313 w2356 w2382 w2406 w2427 w2455 w2469 w2490 w2511 w2532 w2554 w2574 w2603 w2623 w2650 w2670] -> w967
            tunnel: w966 -> [_ _ _ _ _ _ _ _ _ _ _ _ _ w1487 _ _ _ _ _ _ _ _ _ _ _ w1796 _ _ _ _ _ _ w1960 w2012 _ _ _ _ _ _ _ _ _ _ _ _ _ _ _ _ _ _ _ _ _ _ _ _ _ _ _]
            tunnel: w965 -> [_ _ _ _ _ _ _ _ _ _ _ _ _ w1486 _ _ _ _ _ _ _ _ _ _ _ w1795 _ _ _ _ _ _ w1961 w2011 _ _ _ _ _ _ _ _ _ _ _ _ _ _ _ _ _ _ _ _ _ _ _ _ _ _ _]
            tunnel: w962 -> [_ _ _ _ _ _ _ _ _ _ _ _ _ _ _ _ w1542 w1577 w1608 w1640 _ _ _ _ _ _ _ _ _ _ _ _ _ _ _ _ _ _ _ _ _ _ _ _ _ _ _ _ _ _ _ _ _ _ _ _ _ _ _ _ _]
            tunnel: [_ _ _ _ _ _ _ _ _ _ _ _ _ _ _ _ w1546 w1579 w1609 w1643 _ _ _ _ TRUE w1784 w1818 w1852 _ _ _ _ _ _ _ _ _ _ _ _ _ _ _ _ _ _ _ _ _ _ _ _ _ _ _ _ _ _ _ _ _] -> w961
            tunnel: w960 -> [_ _ _ _ _ _ _ _ _ _ _ _ _ _ _ _ w1545 w1584 w1612 w1641 _ _ _ _ w1747 w1790 w1823 w1851 _ _ _ _ _ _ _ _ _ _ _ _ _ _ _ _ _ _ _ _ _ _ _ _ _ _ _ _ _ _ _ _ _]
            tunnel: w959 -> [_ _ _ _ _ _ _ _ _ _ _ _ _ _ _ _ w1544 w1583 w1611 w1642 _ _ _ _ w1746 w1789 w1822 w1850 _ _ _ _ _ _ _ _ _ _ _ _ _ _ _ _ _ _ _ _ _ _ _ _ _ _ _ _ _ _ _ _ _]
            tunnel: [_ _ _ _ _ _ _ _ _ _ _ _ _ _ _ w1519 w1545 w1584 w1612 w1641 _ _ _ _ w1747 w1790 w1820 w1851 _ _ _ _ _ _ _ _ _ _ _ _ _ _ _ _ _ _ _ _ _ _ _ _ _ _ _ _ _ _ _ _ _] -> w958
            tunnel: [_ _ _ _ _ _ _ _ _ _ _ _ _ _ _ w1520 w1544 w1583 w1611 w1642 _ _ _ _ w1746 w1789 w1821 w1850 _ _ _ _ _ _ _ _ _ _ _ _ _ _ _ _ _ _ _ _ _ _ _ _ _ _ _ _ _ _ _ _ _] -> w957
            tunnel: [_ _ _ _ _ _ _ _ _ _ _ _ _ _ _ w1517 w1543 w1578 w1605 w1639 _ _ _ _ _ _ _ _ _ _ _ _ _ _ _ _ _ _ _ _ _ _ _ _ _ _ _ _ _ _ _ _ _ _ _ _ _ _ _ _ _] -> w956
            tunnel: [_ _ _ _ _ _ _ _ _ _ _ _ _ _ _ w1518 w1542 w1577 w1606 w1640 _ _ _ _ _ _ _ _ _ _ _ _ _ _ _ _ _ _ _ _ _ _ _ _ _ _ _ _ _ _ _ _ _ _ _ _ _ _ _ _ _] -> w955
            tunnel: [_ _ _ _ _ _ _ _ _ _ _ _ _ _ _ _ _ w1576 _ _ _ _ _ _ _ w1787 _ _ _ _ _ _ _ _ _ _ _ _ _ _ _ _ _ _ _ _ _ _ _ _ _ _ _ _ _ _ _ _ _ _ _] -> w952
            tunnel: [_ _ _ _ _ _ _ _ _ _ _ _ _ _ _ _ _ w1575 _ _ _ _ _ _ _ w1788 _ _ _ _ _ _ _ _ _ _ _ _ _ _ _ _ _ _ _ _ _ _ _ _ _ _ _ _ _ _ _ _ _ _ _] -> w954
            tunnel: w949 -> [_ _ _ _ _ _ _ _ _ _ _ _ _ _ _ _ w1541 w1574 w1604 w1638 _ _ _ _ w1742 w1786 w1819 w1853 _ _ _ _ _ _ _ _ _ _ _ _ _ _ _ _ _ _ _ _ _ _ _ _ _ _ _ _ _ _ _ _ _]
            tunnel: [_ _ _ _ _ _ _ _ _ _ _ _ _ _ _ _ w1541 w1574 w1604 w1638 _ _ _ _ w1742 w1785 w1819 w1853 _ _ _ _ _ _ _ _ _ _ _ _ _ _ _ _ _ _ _ _ _ _ _ _ _ _ _ _ _ _ _ _ _] -> w948
            frame "Start1", Default {
            }
            frame "Start2" {
            }
            frame "Start3" {
            }
            frame "saveSettings1" {
              n520 = call "myRIO_BRig_RT_dataExp_Audio_freq__L.vi"() -> ("output_Audio_freq__L"=w1142:i32)  [unwired: 11 in]
              n521 = call "myRIO_BRig_RT_dataExp_Audio_freq__R.vi"() -> ("output_Audio_freq__R"=w1139:i32)  [unwired: 11 in]
              n522 = call "myRIO_BRig_RT_dataExp_Audio_amp__L.vi"() -> ("output_Audio_amp__L"=w1136:i32)  [unwired: 11 in]
              n523 = call "myRIO_BRig_RT_dataExp_Audio_amp__R.vi"() -> ("output_Audio_amp__R"=w1134:i32)  [unwired: 11 in]
              n524 = call "myRIO_BRig_RT_dataExp_TPB_min__L.vi"() -> ("output_TPB_min__L"=w1152:i32)  [unwired: 11 in]
              n525 = call "myRIO_BRig_RT_dataExp_TPB_min__R.vi"() -> ("output_TPB_min__R"=w1150:i32)  [unwired: 11 in]
              n526 = call "myRIO_BRig_RT_dataExp_TPB_max__L.vi"() -> ("output_TPB_max__L"=w1148:i32)  [unwired: 11 in]
              n527 = call "myRIO_BRig_RT_dataExp_TPB_max__R.vi"() -> ("output_TPB_max__R"=w1146:i32)  [unwired: 11 in]
              n528 = call "myRIO_BRig_RT_dataExp_ItrialUntilReward.vi"() -> ("output_I_trialUntilReward"=w1165:i32)  [unwired: 11 in]
              n529 = call "myRIO_BRig_RT_dataExp_IblockUntilReward.vi"() -> ("output_I_blockUntilReward"=w1161:i32)  [unwired: 11 in]
              n530 = call "myRIO_BRig_RT_dataExp_CueCycles.vi"() -> ("output_CueCycles"=w1160:i32)  [unwired: 11 in]
              n531 = call "myRIO_BRig_RT_dataExp_ENL_min.vi"() -> ("output_ENL_min"=w1158:i32)  [unwired: 11 in]
              n532 = call "myRIO_BRig_RT_dataExp_ENL_max.vi"() -> ("output_ENL_max"=w1156:i32)  [unwired: 11 in]
              n533 = call "myRIO_BRig_RT_dataExp_ENL_penalty.vi"() -> ("output_ENL_penalty"=w1154:i32)  [unwired: 11 in]
              n534 = local read "Audio_Freq__L"() -> (w1143:u16)
              n535 = local read "Audio_Freq__R"() -> (w1138:u16)
              n536 = local read "Audio_Amp__L"() -> (w1135:u16)
              n537 = local read "TpB_Min_L"() -> (w1151:u16)
              n538 = local read "TpB_Min_R"() -> (w1149:u16)
              n539 = local read "TpB_Max_L"() -> (w1147:u16)
              n540 = local read "TpB_Max_R"() -> (w1145:u16)
              n541 = local read "Audio_Amp__R"() -> (w1133:u16)
              n542 = local read "TrialUntilReward"() -> (w1164:bool)
              n543 = local read "CueCycles"() -> (w1159:u16)
              n544 = local read "Tcycle_ENL_min"() -> (w1157:u16)
              n545 = local read "Tcycle_ENL_max"() -> (w1155:u16)
              n546 = local read "Tcycle_ENLPenalty"() -> (w1153:u16)
              n547 = Multiply(x=w1143, y=u16 1000) -> (x*y=w1141:u16)
              n548 = Multiply(x=w1138, y=u16 1000) -> (x*y=w1137:u16)
              n549 = Boolean To (0,1)(Boolean=w1164) -> (0, 1=w1163:i16)
              n550 = To Unsigned Word Integer(number=w1163) -> (unsigned 16bit integer=w1162:u16)
              n551 = local read "BUR_min"() -> (w1127:u16)
              n552 = local read "BUR_max"() -> (w1128:u16)
              n553 = Not Equal To 0?(x=w1127) -> (x != 0?=w1126:bool)
              n554 = Not Equal To 0?(x=w1128) -> (x != 0?=w1125:bool)
              n555 = And(x=w1126, y=w1125) -> (x .and. y?=w1124:bool)
              n556 = Boolean To (0,1)(Boolean=w1124) -> (0, 1=w1129:i16)
              n557 = To Unsigned Word Integer(number=w1129) -> (unsigned 16bit integer=w1123:u16)
              n558 = Replace Array Subset(array=w1167, new element #1=w1162, index #1=w1165, new element #2=w1123, index #2=w1161, new element #3=w1159, index #3=w1160, new element #4=w1157, index #4=w1158, new element #5=w1155, index #5=w1156, new element #6=w1153, index #6=w1154, new element #7=w1151, index #7=w1152, new element #8=w1149, index #8=w1150, new element #9=w1147, index #9=w1148, new element #10=w1145, index #10=w1146, new element #11=w1141, index #11=w1142, new element #12=w1137, index #12=w1139, new element #13=w1135, index #13=w1136, new element #14=w1133, index #14=w1134) -> (w1166:u16[])
            }
            frame "saveSettings2" {
              n559 = call "myRIO_BRig_RT_dataExp_Tcycle_RewardPost.vi"() -> ("output_Tcycle_RewardPost"=w1200:i32)  [unwired: 11 in]
              n560 = call "myRIO_BRig_RT_dataExp_Tcycle_Wrong.vi"() -> ("output_Tcycle_Wrong"=w1198:i32)  [unwired: 11 in]
              n561 = call "myRIO_BRig_RT_dataExp_Tcycle_Timeout.vi"() -> ("output_Tcycle_Timeout"=w1196:i32)  [unwired: 11 in]
              n562 = call "myRIO_BRig_RT_dataExp_Tcycle_Cue_min.vi"() -> ("output_Tcycle_Cue_min"=w1194:i32)  [unwired: 11 in]
              n563 = call "myRIO_BRig_RT_dataExp_Tcycle_Cue_max.vi"() -> ("output_Tcycle_Cue_max"=w1193:i32)  [unwired: 11 in]
              n564 = call "myRIO_BRig_RT_dataExp_Tcycle_CuePenalty.vi"() -> ("output_Tcycle_CuePenalty"=w1192:i32)  [unwired: 11 in]
              n565 = call "myRIO_BRig_RT_dataExp_nBlock.vi"() -> ("output_nBlock"=w1209:i32)  [unwired: 11 in]
              n566 = call "myRIO_BRig_RT_dataExp_nTrial.vi"() -> ("output_nTrial"=w1208:i32)  [unwired: 11 in]
              n567 = call "myRIO_BRig_RT_dataExp_runTime_seconds.vi"() -> ("output_RunTime_minutes"=w1207:i32)  [unwired: 11 in]
              n568 = call "myRIO_BRig_RT_dataExp_Tcycle_Selection.vi"() -> ("output_Tcycle_Selection"=w1206:i32)  [unwired: 11 in]
              n569 = call "myRIO_BRig_RT_dataExp_Tcycle_Reward__L.vi"() -> ("output_Tcycle_Reward__L"=w1204:i32)  [unwired: 11 in]
              n570 = call "myRIO_BRig_RT_dataExp_Tcycle_Reward__R.vi"() -> ("output_Tcycle_Reward__R"=w1202:i32)  [unwired: 11 in]
              n571 = local read "Tcycle_RewardPost"() -> (w1199:u16)
              n572 = local read "Tcycle_Wrong"() -> (w1197:u16)
              n573 = local read "Tcycle_Timeout"() -> (w1195:u16)
              n574 = local read "Tcycle_CuePenalty"() -> (w1185:u16)
              n575 = local read "Tcycle_Cue_max"() -> (w1173:u16)
              n576 = local read "Tcycle_Cue_min"() -> (w1174:u16)
              n577 = local read "Tcycle_Selection"() -> (w1205:u16)
              n578 = local read "Tcycle_Reward_L"() -> (w1203:u16)
              n579 = local read "Tcycle_Reward_R"() -> (w1201:u16)
              n580 = Replace Array Subset(array=w1211, new element #1=u16 0, index #1=w1209, new element #2=u16 0, index #2=w1208, new element #3=u16 0, index #3=w1207, new element #4=w1205, index #4=w1206, new element #5=w1203, index #5=w1204, new element #6=w1201, index #6=w1202, new element #7=w1199, index #7=w1200, new element #8=w1197, index #8=w1198, new element #9=w1195, index #9=w1196, new element #10=w1174, index #10=w1194, new element #11=w1173, index #11=w1193, new element #12=w1185, index #12=w1192) -> (w1210:u16[])
            }
            frame "saveSettings3" {
              n581 = call "myRIO_BRig_RT_dataExp_BUR_min.vi"() -> ("output_BUR_min"=w1235:i32)  [unwired: 11 in]
              n582 = call "myRIO_BRig_RT_dataExp_BUR_max.vi"() -> ("output_BUR_max"=w1233:i32)  [unwired: 11 in]
              n583 = call "myRIO_BRig_RT_dataExp_Audio_sp__L.vi"() -> ("output_Audio_sp__L"=w1230:i32)  [unwired: 11 in]
              n584 = call "myRIO_BRig_RT_dataExp_Audio_sp__R.vi"() -> ("output_Audio_sp__R"=w1229:i32)  [unwired: 11 in]
              n585 = local read "sp_LeftSpout"() -> (w1228:u16)
              n586 = local read "BUR_max"() -> (w1232:u16)
              n587 = local read "sp_RightSpout"() -> (w1227:u16)
              n588 = local read "BUR_min"() -> (w1234:u16)
              n589 = Replace Array Subset(array=w1236, new element #1=w1234, index #1=w1235, new element #2=w1232, index #2=w1233, new element #3=w1228, index #3=w1230, new element #4=w1227, index #4=w1229) -> (w1231:u16[])
            }
            frame "saveSettings4_LC_ENL" {
              # "delayOpt"
              # "Trial"
              # "Tdelay"
              # "Probability"
              # "OnOff"
              # "Block"
              # "ENL1"
              n590 = call "myRIO_BRig_RT_dataLC_ENL1_First_Block.vi"() -> ("output_ENL1_First_Block"=w1270:i32)  [unwired: 11 in]
              n591 = call "myRIO_BRig_RT_dataLC_ENL1_First_OnOff.vi"() -> ("output_ENL1_First_OnOff"=w1268:i32)  [unwired: 11 in]
              n592 = call "myRIO_BRig_RT_dataLC_ENL1_First_Probability.vi"() -> ("output_ENL1_First_Probability"=w1264:i32)  [unwired: 11 in]
              n593 = call "myRIO_BRig_RT_dataLC_ENL1_First_Tdelay.vi"() -> ("output_ENL1_First_Tdelay"=w1262:i32)  [unwired: 11 in]
              n594 = call "myRIO_BRig_RT_dataLC_ENL1_First_Count.vi"() -> ("output_ENL1_First_Count"=w1260:i32)  [unwired: 11 in]
              n595 = local read "LC_ENL1_delayOpt"() -> (w1247:bool)
              n596 = local read "LC_ENL1_Probability"() -> (w1263:u16)
              n597 = local read "LC_ENL1_Block"() -> (w1269:u16)
              n598 = local read "LC_ENL1_Tdelay"() -> (w1261:u16)
              n599 = local read "LC_ENL1_OnOff"() -> (w1267:bool)
              n600 = local read "LC_ENL2_Trial"() -> (w1259:u16)
              n601 = call "myRIO_BRig_RT_dataLC_ENL1_First_delayOpt.vi"() -> ("output_ENL1_First_delayOpt"=w1246:i32)  [unwired: 11 in]
              n602 = Boolean To (0,1)(Boolean=w1247) -> (0, 1=w1248:i16)
              n603 = Boolean To (0,1)(Boolean=w1267) -> (0, 1=w1266:i16)
              n604 = To Unsigned Word Integer(number=w1248) -> (unsigned 16bit integer=w1245:u16)
              n605 = To Unsigned Word Integer(number=w1266) -> (unsigned 16bit integer=w1265:u16)
              n606 = Replace Array Subset(array=w1271, new element #1=w1269, index #1=w1270, new element #2=w1265, index #2=w1268, new element #3=w1263, index #3=w1264, new element #4=w1261, index #4=w1262, new element #5=w1259, index #5=w1260, new element #6=w1245, index #6=w1246) -> (w1272:u16[])
            }
            frame "saveSettings5_LC_Cue" {
              # "delayOpt"
              # "Trial"
              # "Tdelay"
              # "Probability"
              # "OnOff"
              # "Block"
              # "Cue1"
              n607 = call "myRIO_BRig_RT_dataLC_Cue1_First_Block.vi"() -> ("output_Cue1_First_Block"=w1306:i32)  [unwired: 11 in]
              n608 = call "myRIO_BRig_RT_dataLC_Cue1_First_OnOff.vi"() -> ("output_Cue1_First_OnOff"=w1304:i32)  [unwired: 11 in]
              n609 = call "myRIO_BRig_RT_dataLC_Cue1_First_Probability.vi"() -> ("output_Cue1_First_Probability"=w1300:i32)  [unwired: 11 in]
              n610 = call "myRIO_BRig_RT_dataLC_Cue1_First_Tdelay.vi"() -> ("output_Cue1_First_Tdelay"=w1298:i32)  [unwired: 11 in]
              n611 = call "myRIO_BRig_RT_dataLC_Cue1_First_Count.vi"() -> ("output_Cue1_First_Count"=w1296:i32)  [unwired: 11 in]
              n612 = local read "LC_Cue1_delayOpt"() -> (w1282:bool)
              n613 = local read "LC_Cue1_Probability"() -> (w1299:u16)
              n614 = local read "LC_Cue1_Block"() -> (w1305:u16)
              n615 = local read "LC_Cue1_Tdelay"() -> (w1297:u16)
              n616 = local read "LC_Cue1_OnOff"() -> (w1303:bool)
              n617 = local read "LC_Cue2_Trial"() -> (w1295:u16)
              n618 = call "myRIO_BRig_RT_dataLC_Cue1_First_delayOpt.vi"() -> ("output_Cue1_First_delayOpt"=w1283:i32)  [unwired: 11 in]
              n619 = Boolean To (0,1)(Boolean=w1282) -> (0, 1=w1284:i16)
              n620 = To Unsigned Word Integer(number=w1284) -> (unsigned 16bit integer=w1281:u16)
              n621 = Boolean To (0,1)(Boolean=w1303) -> (0, 1=w1302:i16)
              n622 = To Unsigned Word Integer(number=w1302) -> (unsigned 16bit integer=w1301:u16)
              n623 = Replace Array Subset(array=w1307, new element #1=w1305, index #1=w1306, new element #2=w1301, index #2=w1304, new element #3=w1299, index #3=w1300, new element #4=w1297, index #4=w1298, new element #5=w1295, index #5=w1296, new element #6=w1281, index #6=w1283) -> (w1308:u16[])
            }
            frame "saveSettings6_LC_Other" {
              # "Trial"
              # "Tdelay"
              # "Probability"
              # "OnOff"
              # "Block"
              # "Wrong"
              # "Trial"
              # "Tdelay"
              # "Probability"
              # "OnOff"
              # "Block"
              # "Reward"
              n624 = call "myRIO_BRig_RT_dataLC_Wrong_Block.vi"() -> ("output_Wrong_Block"=w1338:i32)  [unwired: 11 in]
              n625 = call "myRIO_BRig_RT_dataLC_Wrong_OnOff.vi"() -> ("output_Wrong_OnOff"=w1337:i32)  [unwired: 11 in]
              n626 = call "myRIO_BRig_RT_dataLC_Wrong_Probability.vi"() -> ("output_Wrong_Probability"=w1336:i32)  [unwired: 11 in]
              n627 = call "myRIO_BRig_RT_dataLC_Wrong_Tdelay.vi"() -> ("output_Wrong_Tdelay"=w1335:i32)  [unwired: 11 in]
              n628 = call "myRIO_BRig_RT_dataLC_Wrong_Trial.vi"() -> ("output_Wrong_Trial"=w1334:i32)  [unwired: 11 in]
              n629 = call "myRIO_BRig_RT_dataLC_Reward_Block.vi"() -> ("output_Reward_Block"=w1350:i32)  [unwired: 11 in]
              n630 = call "myRIO_BRig_RT_dataLC_Reward_OnOff.vi"() -> ("output_Reward_OnOff"=w1348:i32)  [unwired: 11 in]
              n631 = call "myRIO_BRig_RT_dataLC_Reward_Probability.vi"() -> ("output_Reward_Probability"=w1344:i32)  [unwired: 11 in]
              n632 = call "myRIO_BRig_RT_dataLC_Reward_Tdelay.vi"() -> ("output_Reward_Tdelay"=w1342:i32)  [unwired: 11 in]
              n633 = call "myRIO_BRig_RT_dataLC_Reward_Trial.vi"() -> ("output_Reward_Trial"=w1340:i32)  [unwired: 11 in]
              n634 = local read "LC_Wrong_OnOff"() -> (w1332:bool)
              n635 = local read "LC_Wrong_Probability"() -> (w1329:u16)
              n636 = local read "LC_Wrong_Block"() -> (w1331:u16)
              n637 = local read "LC_Wrong_Tdelay"() -> (w1328:u16)
              n638 = local read "LC_Wrong_Trial"() -> (w1327:u16)
              n639 = local read "LC_Reward_Probability"() -> (w1343:u16)
              n640 = local read "LC_Reward_Block"() -> (w1349:u16)
              n641 = local read "LC_Reward_Tdelay"() -> (w1341:u16)
              n642 = local read "LC_Reward_OnOff"() -> (w1347:bool)
              n643 = local read "LC_Reward_Trial"() -> (w1339:u16)
              n644 = Boolean To (0,1)(Boolean=w1332) -> (0, 1=w1333:i16)
              n645 = Boolean To (0,1)(Boolean=w1347) -> (0, 1=w1346:i16)
              n646 = To Unsigned Word Integer(number=w1333) -> (unsigned 16bit integer=w1330:u16)
              n647 = To Unsigned Word Integer(number=w1346) -> (unsigned 16bit integer=w1345:u16)
              n648 = Replace Array Subset(array=w1351, new element #1=w1349, index #1=w1350, new element #2=w1345, index #2=w1348, new element #3=w1343, index #3=w1344, new element #4=w1341, index #4=w1342, new element #5=w1339, index #5=w1340, new element #6=w1331, index #6=w1338, new element #7=w1330, index #7=w1337, new element #8=w1329, index #8=w1336, new element #9=w1328, index #9=w1335, new element #10=w1327, index #10=w1334) -> (w1352:u16[])
            }
            frame "setSettings_Audio" {
              # "amp_L"
              # "amp_R"
              # "freq_L"
              # "freq_R"
              n649 = call "myRIO_BRig_RT_dataExp_Audio_amp__L.vi"() -> ("output_Audio_amp__L"=w1375:i32)  [unwired: 11 in]
              n650 = call "myRIO_BRig_RT_dataExp_Audio_amp__R.vi"() -> ("output_Audio_amp__R"=w1374:i32)  [unwired: 11 in]
              n651 = call "myRIO_BRig_RT_dataExp_Audio_freq__L.vi"() -> ("output_Audio_freq__L"=w1373:i32)  [unwired: 11 in]
              n652 = call "myRIO_BRig_RT_dataExp_Audio_freq__R.vi"() -> ("output_Audio_freq__R"=w1372:i32)  [unwired: 11 in]
              n653 = Index Array(array=w1371, index #1=w1375, index #2=w1374, index #3=w1373, index #4=w1372) -> (element #1=w1370:u16, element #2=w1368:u16, element #3=w1369:u16, element #4=w1367:u16)
            }
            frame "initBlock" {
              n654 = call "myRIO_Brig_RT__Case_Exp_State_initBlock.vi"("input_spout"=w1407, "input_dataExp"=w1405, "input_dataCurrent"=w1406) -> ("output_spout"=w1384:enum16{"Left", "Right"}, "output_state"=w1408:T2, "output_dataExp"=w1404:u16[], "output_dataCurrent"=w1390:u16[], "output_TpB_target"=→"TpB_target":u16)  [unwired: 4 in]
              "cSpout" <- w1384
              n655 = call "myRIO_BRig_RT_dataCurrent_iBlock.vi"() -> ("output_iBlock"=w1389:i32)  [unwired: 11 in]
              n656 = Index Array(array=w1390, index=w1389) -> (element=→"iBlock":u16)
            }
            frame "initBlock2" {
              n657 = local write "nRewards_cur"(u16 0 ("nRewards_cur")) -> ()
              n658 = call "myRIO_BRig_RT__Case_Exp_State_initBlock2.vi"("input_spout"=w1416, "input_dataBlock"=w1417, "input_dataCurrent"=w1415) -> ("idxDataBlock"=w1412:i32, "output_dataBlock"=w1414:u16[][])  [unwired: 7 in]
            }
            frame "initTrial" {
              n659 = call "myRIO_Brig_RT__Case_Exp_State_initTrial.vi"("input_dataExp"=w1446, "input_dataCurrent"=w1447) -> ("output_state"=w1448:T2, "output_dataExp"=w1445:u16[], "output_dataCurrent"=w1435:u16[])  [unwired: 7 in]
              n660 = call "myRIO_BRig_RT_dataCurrent_iTrial.vi"() -> ("output_iTrial"=w1434:i32)  [unwired: 11 in]
              n661 = Index Array(array=w1435, index=w1434) -> (element=→"iTrial":u16)
            }
            frame "initTrial2" {
              w1453 = u32 10
              # "laser time"
              # "Wrong tDelay"
              # "Reward tDelay"
              # "trialUntilReward"
              n662 = call "myRIO_BRig_RT__Case_Exp_subState_LC__initTrial.vi"("input_dataTrial"=w1463, "input_spout"=w1472, "input_dataCurrent"=w1461, "input_dataLC"=w1458) -> ("output_LC_Wrong"=w1473:bool, "output_LC_led_Wrong"=w1465:bool, "output_LC_Reward"=w1474:bool, "output_LC_led_Reward"=w1464:bool, "output_dataTrial"=w1462:u16[][])  [unwired: 2 in]
              n663 = Equal?(x=w1472, y=enum16{"Left", "Right"}."Right") -> (x = y?=w1470:bool)
              n664 = call "myRIO_BRig_RT_dataExp_ItrialUntilReward.vi"() -> ("output_I_trialUntilReward"=w1468:i32)  [unwired: 11 in]
              n665 = Index Array(array=w1469, index=w1468) -> (element=w1467:u16)
              n666 = call "myRIO_BRig_RT_dataLC_Reward_Tdelay.vi"() -> ("output_Reward_Tdelay"=w1459:i32)  [unwired: 11 in]
              n667 = call "myRIO_BRig_RT_dataLC_Wrong_Tdelay.vi"() -> ("output_Wrong_Tdelay"=w1460:i32)  [unwired: 11 in]
              n668 = Not Equal To 0?(x=w1467) -> (x != 0?=w1466:bool)
              n669 = Index Array(array=w1458, index #1=w1459, index #2=w1460) -> (element #1=w1457:u16, element #2=w1456:u16)
              n670 = To Unsigned Long Integer(number=w1457) -> (unsigned 32bit integer=w1455:u32)
              n671 = To Unsigned Long Integer(number=w1456) -> (unsigned 32bit integer=w1454:u32)
              n672 = xnode "Read/Write Control"("FPGA VI Reference In"=w1487, "error in"=w1486, "SelectionState"=FALSE, "laserResponse_reward"=w1474, "laserResponse_wrong"=w1473, "laserResponse_reward_LED"=w1464, "laserResponse_wrong_LED"=w1465, "Left(F)_or_Right(T)"=w1470, "ignoreWrong"=w1466, "tCycle_laser_rew"=w1453, "tDelay_laser_rew"=w1455, "tCycle_laser_wro"=w1453, "tDelay_laser_wro"=w1454) -> ("error out"=→"error_initTrial":errorcluster)  [unwired: 1 out]
            }
            frame "initTrial3" {
              n673 = call "myRIO_BRig_RT__Case_Exp_State_initTrial_dataTrial.vi"("input_spout"=w1493, "input_dataCurrent"=w1494, "input_dataTrial"=w1496) -> ("output_dataTrial"=w1495:u16[][])  [unwired: 8 in]
            }
            frame "initTrial4" {
              n674 = call "myRIO_BRig_RT__Case_Exp_State_initTrial_LC_ENL1.vi"("input_dataTrial"=w1514, "input_spout"=w1521, "input_dataLC"=w1522, "input_dataCurrent"=w1516) -> (0:w1520, 1:w1519, "output_LC__ENL1"=w1518:bool, "output_LC_led__ENL1"=w1517:bool, "output_dataTrial"=w1513:u16[][], "output_dataCurrent"=w1515:u16[])  [unwired: 2 in]
            }
            frame "ENL1_pre" {
              # "ENL1_n"
              # "Tcycle"
              # "counter"
              n675 = call "myRIO_BRig_RT_dataCurrent_Tcycle_generic.vi"() -> ("output_Tcycle_generic"=w1569:i32)  [unwired: 11 in]
              n676 = call "myRIO_BRig_RT_dataCurrent_count_generic.vi"() -> ("output_count_generic"=w1571:i32)  [unwired: 11 in]
              n677 = call "myRIO_BRig_RT_dataCurrent_ENL.vi"() -> ("output_ENL"=w1568:i32)  [unwired: 11 in]
              n678 = call "myRIO_BRig_RT_dataCurrent_ENL1_n.vi"() -> ("output_ENL1_n"=w1540:i32)  [unwired: 11 in]
              n679 = Index Array(array=w1562, index #1=w1568, index #2=w1540) -> (element #1=w1567:u16, element #2=w1539:u16)
              n680 = Increment(x=w1539) -> (x+1=w1538:u16)
              n681 = Replace Array Subset(array=w1562, new element #1=u16 0 ("new element/subarray"), index #1=w1571, new element #2=w1567, index #2=w1569, new element #3=w1538, index #3=w1540) -> (w1566:u16[])
              n682 = Select(t=myRIO_BRig_RT__Case_Exp_stateList."ENL1Penalty_pre" ("Enum"), s=w1550, f=myRIO_BRig_RT__Case_Exp_stateList."ENL1" ("Enum")) -> (s? t:f=w1547:T2)
            }
            frame "ENL1" {
              n683 = call "myRIO_BRig_RT__Case_Exp_State_ENL1.vi"("input_LC"=w1577, "I_lick"=w1582, "input_LC_led"=w1578, "input_state"=w1588, "input_dataCurrent"=w1587) -> ("output_trigger_laser_led"=w1576:bool, "output_state"=w1585:T2, "output_dataCurrent"=w1586:u16[], "output_trigger_laser"=w1575:bool)  [unwired: 3 in]
              n684 = Or(x=w1576, y=w1580) -> (x .or. y?=w1579:bool)
            }
            frame "ENL1Penalty_pre" {
              w1607 = FALSE
              # "Tcycle"
              # "counter"
              n685 = call "myRIO_BRig_RT_dataCurrent_Tcycle_generic.vi"() -> ("output_Tcycle_generic"=w1631:i32)  [unwired: 11 in]
              n686 = call "myRIO_BRig_RT_dataCurrent_count_generic.vi"() -> ("output_count_generic"=w1633:i32)  [unwired: 11 in]
              n687 = Select(t=w1607, s=w1609, f=w1610) -> (s? t:f=w1605:bool)
              n688 = Select(t=w1607, s=w1609, f=w1608) -> (s? t:f=w1606:bool)
              n689 = call "myRIO_BRig_RT_dataExp_ENL_penalty.vi"() -> ("output_ENL_penalty"=w1626:i32)  [unwired: 11 in]
              n690 = Index Array(array=w1627, index=w1626) -> (element=w1630:u16)
              n691 = Replace Array Subset(array=w1628, new element #1=u16 0 ("new element/subarray"), index #1=w1633, new element #2=w1630, index #2=w1631) -> (w1629:u16[])
            }
            frame "ENL1Penalty" {
              n692 = call "myRIO_BRig_RT__Case_Exp_State_ENL1Penalty.vi"("input_state"=w1656, "input_dataCurrent"=w1660) -> ("output_state"=w1657:T2, "output_dataCurrent"=w1659:u16[])  [unwired: 8 in]
            }
            frame "ENL2_pre" {
            }
            frame "ENL2" {
            }
            frame "ENL2Penalty_pre" {
            }
            frame "ENL2Penalty" {
            }
            frame "Cue1_pre" {
              # "Cue1_n"
              # "Tcycle_Cue1"
              # "0 = L, 1 = R, 2 = both"
              # "sp_R"
              # "sp_L"
              # "Tcycle"
              # "counter"
              n693 = Equal?(x=w1769, y=enum16{"Left", "Right"}."Left") -> (x = y?=w1768:bool)
              n694 = call "myRIO_BRig_RT_dataExp_Audio_sp__L.vi"() -> ("output_Audio_sp__L"=w1767:i32)  [unwired: 11 in]
              n695 = call "myRIO_BRig_RT_dataExp_Audio_sp__R.vi"() -> ("output_Audio_sp__R"=w1766:i32)  [unwired: 11 in]
              n696 = call "myRIO_BRig_RT_dataCurrent_Tcycle_generic.vi"() -> ("output_Tcycle_generic"=w1779:i32)  [unwired: 11 in]
              n697 = call "myRIO_BRig_RT_dataCurrent_count_generic.vi"() -> ("output_count_generic"=w1781:i32)  [unwired: 11 in]
              n698 = Select(t=w1767, s=w1768, f=w1766) -> (s? t:f=w1765:i32)
              n699 = call "myRIO_BRig_RT_dataCurrent_Cue1_n.vi"() -> ("output_Cue1_n"=w1743:i32)  [unwired: 11 in]
              n700 = call "myRIO_BRig_RT_dataCurrent_Tcycle_cue.vi"() -> ("output_Tcycle_cue"=w1752:i32)  [unwired: 11 in]
              n701 = Index Array(array=w1771, index=w1765) -> (element=w1763:u16)
              n702 = Index Array(array=w1753, index #1=w1752, index #2=w1743) -> (element #1=w1754:u16, element #2=w1745:u16)
              n703 = Increment(x=w1745) -> (x+1=w1744:u16)
              n704 = Not Equal To 0?(x=w1763) -> (x != 0?=w1761:bool)
              n705 = Not Equal?(x=w1763, y=u16 1) -> (x != y?=w1762:bool)
              n706 = Replace Array Subset(array=w1753, new element #1=u16 0 ("new element/subarray"), index #1=w1781, new element #2=w1754, index #2=w1779, new element #3=w1744, index #3=w1743) -> (w1778:u16[])
              n707 = Select(t=myRIO_BRig_RT__Case_Exp_stateList."Cue1Penalty_pre" ("Enum"), s=w1749, f=myRIO_BRig_RT__Case_Exp_stateList."Cue1" ("Enum")) -> (s? t:f=w1750:T2)
            }
            frame "Cue1" {
              n708 = call "myRIO_BRig_RT__Case_Exp_State_Cue1.vi"("input_LC"=w1789, "I_lick"=w1792, "input_LC_led"=w1790, "input_state"=w1794, "input_dataCurrent"=w1812) -> ("output_trigger_laser_led"=w1787:bool, "output_state"=w1793:T2, "output_dataCurrent"=w1811:u16[], "output_trigger_laser"=w1788:bool)  [unwired: 3 in]
              n709 = Or(x=w1787, y=w1786) -> (x .or. y?=w1785:bool)
              n710 = Equal?(x=myRIO_BRig_RT__Case_Exp_stateList."Selection_pre", y=w1793) -> (x = y?=w1797:bool)
              n711 = xnode "Read/Write Control"("FPGA VI Reference In"=w1796, "error in"=w1795, "SelectionState"=w1797) -> ()  [unwired: 2 out]
            }
            frame "Cue1Penalty_pre" {
              w1824 = FALSE
              # "Tcycle"
              # "counter"
              n712 = call "myRIO_BRig_RT_dataCurrent_Tcycle_generic.vi"() -> ("output_Tcycle_generic"=w1844:i32)  [unwired: 11 in]
              n713 = call "myRIO_BRig_RT_dataCurrent_count_generic.vi"() -> ("output_count_generic"=w1846:i32)  [unwired: 11 in]
              n714 = call "myRIO_BRig_RT_dataExp_Tcycle_CuePenalty.vi"() -> ("output_Tcycle_CuePenalty"=w1843:i32)  [unwired: 11 in]
              n715 = Select(t=w1824, s=w1819, f=w1823) -> (s? t:f=w1820:bool)
              n716 = Select(t=w1824, s=w1819, f=w1822) -> (s? t:f=w1821:bool)
              n717 = Index Array(array=w1838, index=w1843) -> (element=w1842:u16)
              n718 = Replace Array Subset(array=w1840, new element #1=u16 0 ("new element/subarray"), index #1=w1846, new element #2=w1842, index #2=w1844) -> (w1839:u16[])
            }
            frame "Cue1Penalty" {
              n719 = call "myRIO_BRig_RT__Case_Exp_State_Cue1Penalty.vi"("input_state"=w1870, "input_dataCurrent"=w1871) -> ("output_state"=w1868:T2, "output_dataCurrent"=w1869:u16[])  [unwired: 8 in]
            }
            frame "Cue2_pre" {
              n720 = call "myRIO_BRig_RT__Case_Exp_subState_LC__Cue2.vi"("input_spout"=w1888, "input_dataCurrent"=w1889, "input_dataLC"=w1887) -> ()  [unwired: 6 in, 2 out]
            }
            frame "Cue2" {
            }
            frame "Cue2Penalty_pre" {
            }
            frame "Cue2Penalty" {
            }
            frame "Selection_pre" {
              # "Tcycle"
              # "counter"
              n721 = xnode "Read/Write Control"("FPGA VI Reference In"=w1960, "error in"=w1961) -> ("error out"=→"error_Selection_pre":errorcluster, "SelectReward"=w1953:bool, "SelectWrong"=w1955:bool)  [unwired: 1 out]
              n722 = call "myRIO_BRig_RT_dataCurrent_Tcycle_generic.vi"() -> ("output_Tcycle_generic"=w1982:i32)  [unwired: 11 in]
              n723 = call "myRIO_BRig_RT_dataCurrent_count_generic.vi"() -> ("output_count_generic"=w1984:i32)  [unwired: 11 in]
              n724 = call "myRIO_BRig_RT_dataExp_Tcycle_Selection.vi"() -> ("output_Tcycle_Selection"=w1981:i32)  [unwired: 11 in]
              n725 = Index Array(array=w1978, index=w1981) -> (element=w1980:u16)
              n726 = Replace Array Subset(array=w1976, new element #1=u16 0 ("new element/subarray"), index #1=w1984, new element #2=w1980, index #2=w1982) -> (w1979:u16[])
              n727 = Or(x=w1953, y=w1955) -> (x .or. y?=w1954:bool)
              n728 = Select(t=myRIO_BRig_RT__Case_Exp_stateList."SelectReward_pre" ("Enum"), s=w1953, f=myRIO_BRig_RT__Case_Exp_stateList."SelectWrong_pre" ("Enum")) -> (s? t:f=w1959:T2)
              n729 = Select(t=w1959, s=w1954, f=myRIO_BRig_RT__Case_Exp_stateList."Selection" ("Enum")) -> (s? t:f=w1956:T2)
            }
            frame "Selection" {
              # "counter\nSelection"
              # "increment"
              # "get Tcycle"
              # "get count"
              n730 = xnode "Read/Write Control"("FPGA VI Reference In"=w2012, "error in"=w2011) -> ("FPGA VI Reference Out"=w1987:refnum<k20>, "error out"=w1988:errorcluster, "SelectReward"=w2008:bool, "SelectWrong"=w2009:bool)
              n731 = call "myRIO_BRig_RT_dataCurrent_Tcycle_generic.vi"() -> ("output_Tcycle_generic"=w2005:i32)  [unwired: 11 in]
              n732 = call "myRIO_BRig_RT_dataCurrent_count_generic.vi"() -> ("output_count_generic"=w1997:i32)  [unwired: 11 in]
              n733 = Index Array(array=w2006, index #1=w2005, index #2=w1997) -> (element #1=w1996:u16, element #2=w2004:u16)
              n734 = call "myRIO_BRig_RT__increment_u16.vi"() -> ("output_increment__u16"=w2003:u16)  [unwired: 11 in]
              n735 = Add(x=w2004, y=w2003) -> (x+y=w1998:u16)
              n736 = Greater?(x=w1996, y=w1998) -> (0:w1999:bool)
              n737 = Select(t=w2002, s=w1999, f=myRIO_BRig_RT__Case_Exp_stateList."SelectTimeout_pre" ("Enum")) -> (s? t:f=w1991:T2)
              n738 = Select(t=w1998, s=w1999, f=w1996) -> (s? t:f=w1994:u16)
              n739 = call "myRIO_BRig_RT_dataCurrent_count_selection.vi"() -> ("output_count_generic"=w1995:i32)  [unwired: 11 in]
              n740 = Select(t=myRIO_BRig_RT__Case_Exp_stateList."SelectReward_pre" ("Enum"), s=w2008, f=myRIO_BRig_RT__Case_Exp_stateList."SelectWrong_pre" ("Enum")) -> (s? t:f=w2007:T2)
              n741 = Replace Array Subset(array=w2006, new element #1=w1994, index #1=w1997, new element #2=w1994, index #2=w1995) -> (w2001:u16[])
              n742 = Or(x=w2008, y=w2009) -> (x .or. y?=w1990:bool)
              n743 = Not(x=w1990) -> (.not. x?=w1989:bool)
              n744 = xnode "Read/Write Control"("FPGA VI Reference In"=w1987, "error in"=w1988, "SelectionState"=w1989) -> ("error out"=→"error_Selection":errorcluster)  [unwired: 1 out]
              n745 = Select(t=w2007, s=w1990, f=w1991) -> (s? t:f=w2010:T2)
            }
            frame "SelectReward_pre" {
              # "iState"
              # "Tcycle\nReward"
              # "nRewTrials"
              # "Tcycle\nGeneric"
              # "counter"
              n746 = call "myRIO_BRig_RT_dataCurrent_nRewTrials.vi"() -> ("output_nRewTrials"=w2044:i32)  [unwired: 11 in]
              n747 = Equal?(x=w2053, y=enum16{"Left", "Right"}."Left") -> (x = y?=w2054:bool)
              n748 = Index Array(array=w2045, index=w2044) -> (element=w2043:u16)
              n749 = call "myRIO_BRig_RT_dataExp_Tcycle_Reward__L.vi"() -> ("output_Tcycle_Reward__L"=w2057:i32)  [unwired: 11 in]
              n750 = call "myRIO_BRig_RT_dataExp_Tcycle_Reward__R.vi"() -> ("output_Tcycle_Reward__R"=w2058:i32)  [unwired: 11 in]
              n751 = Increment(x=w2043) -> (x+1=w2042:u16)
              n752 = Select(t=w2057, s=w2054, f=w2058) -> (s? t:f=w2056:i32)
              n753 = call "myRIO_BRig_RT__Case_Exp_subState_LC__Reward.vi"("input_spout"=w2053, "input_dataCurrent"=w2045, "input_dataLC"=w2052) -> ()  [unwired: 6 in, 2 out]
              n754 = call "myRIO_BRig_RT_dataCurrent_count_generic.vi"() -> ("output_count_generic"=w2047:i32)  [unwired: 11 in]
              n755 = call "myRIO_BRig_RT_dataCurrent_Tcycle_generic.vi"() -> ("output_Tcycle_generic"=w2048:i32)  [unwired: 11 in]
              n756 = Index Array(array=w2059, index=w2056) -> (element=w2049:u16)
              n757 = call "myRIO_BRig_RT_dataCurrent_iState.vi"() -> ("output_iState"=w2037:i32)  [unwired: 11 in]
              n758 = Replace Array Subset(array=w2045, new element #1=w2042, index #1=w2044, new element #2=u16 0 ("new element/subarray"), index #2=w2047, new element #3=w2049, index #3=w2048, new element #4=u16 1 ("new element/subarray"), index #4=w2037) -> (w2060:u16[])
            }
            frame "SelectReward" {
              n759 = call "myRIO_BRig_RT__Case_Exp_State_Reward.vi"("input_dataCurrent"=w2082, "input_state"=w2079, "input_spout"=w2076, "input_LC"=w2077, "input_dataLC"=w2078) -> ("output_dataCurrent"=w2081:u16[], "output_state"=w2080:T2, "output__L"=w2074:bool, "output__R"=w2075:bool)  [unwired: 6 in, 1 out]
            }
            frame "SelectRewardPost_pre" {
              # "nRewards"
              # "nRewTrials"
              # "Tcycle"
              # "counter"
              n760 = call "myRIO_BRig_RT_dataBlock_nRewards__L.vi"() -> ("output_nRewards__L"=w2098:i32)  [unwired: 11 in]
              n761 = call "myRIO_BRig_RT_dataBlock_nRewards__R.vi"() -> ("output_nRewards__R"=w2097:i32)  [unwired: 11 in]
              n762 = call "myRIO_BRig_RT_dataCurrent_Tcycle_generic.vi"() -> ("output_Tcycle_generic"=w2117:i32)  [unwired: 11 in]
              n763 = call "myRIO_BRig_RT_dataCurrent_count_generic.vi"() -> ("output_count_generic"=w2119:i32)  [unwired: 11 in]
              n764 = case shown="\"Left\", Default" w2091 {
                tunnel: w2103 -> [w2124 w2128]
                tunnel: [w2123 w2128] -> w2102
                tunnel: [w2125 w2126] -> w2101
                tunnel: w2100 -> [w2125 w2127]
                frame "Left", Default {
                  n765 = Increment(x=w2124) -> (x+1=w2123:u16)
                }
                frame "Right" {
                  n766 = Increment(x=w2127) -> (x+1=w2126:u16)
                }
              }
              "nRewards_Left" <- w2102
              "nRewards_Right" <- w2101
              n767 = Equal?(x=w2091, y=enum16{"Left", "Right"}."Left") -> (x = y?=w2090:bool)
              n768 = Select(t=w2098, s=w2090, f=w2097) -> (s? t:f=w2096:i32)
              n769 = call "myRIO_BRig_RT_dataExp_Tcycle_RewardPost.vi"() -> ("output_Tcycle_RewardPost"=w2113:i32)  [unwired: 11 in]
              n770 = call "myRIO_BRig_RT_dataCurrent_nRewTrials.vi"() -> ("output_nRewTrials"=w2099:i32)  [unwired: 11 in]
              n771 = Index Array(array=w2114, index=w2113) -> (element=w2116:u16)
              n772 = Index Array(array=w2093, index=w2099) -> (element=w2088:u16)
              n773 = Replace Array Subset(array=w2093, new element #1=u16 0 ("new element/subarray"), index #1=w2119, new element #2=w2116, index #2=w2117) -> (w2115:u16[])
              n774 = Replace Array Subset(array=w2095, new element=w2088, index (row)=w2089, index (col)=w2096) -> (w2094:u16[][])
              n775 = local write "nRewards_cur"(w2088) -> ()
            }
            frame "SelectRewardPost" {
              n776 = call "myRIO_BRig_RT__Case_Exp_State_RewardPost.vi"("input_state"=w2143, "input_dataCurrent"=w2146) -> ("output_state"=w2144:T2, "output_dataCurrent"=w2145:u16[])  [unwired: 8 in]
            }
            frame "SelectWrong_pre" {
              # "iState"
              # "Tcycle"
              # "counter"
              n777 = call "myRIO_BRig_RT_dataCurrent_Tcycle_generic.vi"() -> ("output_Tcycle_generic"=w2171:i32)  [unwired: 11 in]
              n778 = call "myRIO_BRig_RT_dataCurrent_count_generic.vi"() -> ("output_count_generic"=w2173:i32)  [unwired: 11 in]
              n779 = call "myRIO_BRig_RT_dataExp_Tcycle_Wrong.vi"() -> ("output_Tcycle_Wrong"=w2169:i32)  [unwired: 11 in]
              n780 = call "myRIO_BRig_RT__Case_Exp_subState_LC__Wrong.vi"("input_spout"=w2165, "input_dataCurrent"=w2166, "input_dataLC"=w2163) -> ()  [unwired: 6 in, 2 out]
              n781 = Index Array(array=w2167, index=w2169) -> (element=w2170:u16)
              n782 = call "myRIO_BRig_RT_dataCurrent_iState.vi"() -> ("output_iState"=w2157:i32)  [unwired: 11 in]
              n783 = Replace Array Subset(array=w2166, new element #1=u16 0 ("new element/subarray"), index #1=w2173, new element #2=w2170, index #2=w2171, new element #3=u16 2 ("new element/subarray"), index #3=w2157) -> (w2168:u16[])
            }
            frame "SelectWrong" {
              n784 = call "myRIO_BRig_RT__Case_Exp_State_Wrong.vi"("input_dataLC"=w2194, "input_LC"=w2193, "input_state"=w2187, "input_dataCurrent"=w2197) -> ("output_state"=w2184:T2, "output_dataCurrent"=w2196:u16[])  [unwired: 5 in, 1 out]
              n785 = Not Equal?(x=w2187, y=w2184) -> (x != y?=w2186:bool)
              n786 = Select(t=myRIO_BRig_RT__Case_Exp_stateList."SelectWrong_post" ("Enum"), s=w2186, f=w2184) -> (s? t:f=w2183:T2)
            }
            frame "SelectWrong_post" {
            }
            frame "SelectTimeout_pre" {
              # "iState"
              # "Tcycle"
              # "counter"
              n787 = call "myRIO_BRig_RT_dataCurrent_Tcycle_generic.vi"() -> ("output_Tcycle_generic"=w2242:i32)  [unwired: 11 in]
              n788 = call "myRIO_BRig_RT_dataCurrent_count_generic.vi"() -> ("output_count_generic"=w2240:i32)  [unwired: 11 in]
              n789 = call "myRIO_BRig_RT_dataExp_Tcycle_Timeout.vi"() -> ("output_Tcycle_Timeout"=w2244:i32)  [unwired: 11 in]
              n790 = call "myRIO_BRig_RT__Case_Exp_subState_LC__Timeout.vi"("input_spout"=w2235, "input_dataCurrent"=w2236, "input_dataLC"=w2234) -> ()  [unwired: 6 in, 2 out]
              n791 = Index Array(array=w2238, index=w2244) -> (element=w2243:u16)
              n792 = call "myRIO_BRig_RT_dataCurrent_iState.vi"() -> ("output_iState"=w2228:i32)  [unwired: 11 in]
              n793 = Replace Array Subset(array=w2236, new element #1=u16 0 ("new element/subarray"), index #1=w2240, new element #2=w2243, index #2=w2242, new element #3=u16 3 ("new element/subarray"), index #3=w2228) -> (w2239:u16[])
            }
            frame "SelectTimeout" {
              n794 = call "myRIO_BRig_RT__Case_Exp_State_Timeout.vi"("input_dataLC"=w2263, "input_LC"=w2264, "input_state"=w2254, "input_dataCurrent"=w2269) -> ("output_state"=w2255:T2, "output_dataCurrent"=w2268:u16[])  [unwired: 5 in, 1 out]
              n795 = Not Equal?(x=w2254, y=w2255) -> (x != y?=w2258:bool)
              n796 = Select(t=myRIO_BRig_RT__Case_Exp_stateList."SelectTimeout_post" ("Enum"), s=w2258, f=w2255) -> (s? t:f=w2256:T2)
            }
            frame "SelectTimeout_post" {
            }
            frame "endTrial1" {
              # "Update dataBlock"
              n797 = call "myRIO_BRig_RT__Case_Exp_State_endTrial1.vi"("input_spout"=w2302, "input_dataBlock"=w2301, "input_dataCurrent"=w2299) -> ("output_dataBlock"=w2300:u16[][], "output_dataCurrent"=w2298:u16[])  [unwired: 7 in]
            }
            frame "endTrial2" {
              # "update dataTrial"
              n798 = call "myRIO_BRig_RT__Case_Exp_State_endTrial2.vi"("input_spout"=w2321, "input_dataTrial"=w2325, "input_dataCurrent"=w2323) -> ("output_dataTrial"=w2324:u16[][], "output_dataCurrent"=w2322:u16[])  [unwired: 7 in]
            }
            frame "endTrial3" {
              w2347 = myRIO_BRig_RT__Case_Exp_stateList."endBlock" ("Enum")
              # "nRewTrials"
              # "iTrial"
              # "I_blockUntilReward"
              # "TPB"
              # "end block?"
              n799 = local read "STOP_endTrial"() -> (w2345:bool)
              n800 = local read "STOP_abort"() -> (w2344:bool)
              n801 = local read "START"() -> (w2342:bool)
              n802 = call "myRIO_BRig_RT_dataExp_IblockUntilReward.vi"() -> ("output_I_blockUntilReward"=w2354:i32)  [unwired: 11 in]
              n803 = Index Array(array=w2338, index=w2354) -> (element=w2334:u16)
              n804 = Not(x=w2342) -> (.not. x?=w2343:bool)
              n805 = Not Equal To 0?(x=w2334) -> (x != 0?=w2352:bool)
              n806 = Compound Arithmetic op=OR(w2345, w2343, w2344) -> (w2346:bool)
              n807 = call "myRIO_BRig_RT_dataCurrent_nRewTrials.vi"() -> ("output_nRewTrials"=w2350:i32)  [unwired: 11 in]
              n808 = call "myRIO_BRig_RT_dataCurrent_iTrial.vi"() -> ("output_iTrial"=w2351:i32)  [unwired: 11 in]
              n809 = Select(t=w2350, s=w2352, f=w2351) -> (s? t:f=w2349:i32)
              n810 = call "myRIO_BRig_RT_dataCurrent_TpB.vi"() -> ("output_TpB"=w2353:i32)  [unwired: 11 in]
              n811 = Index Array(array=w2339, index #1=w2353, index #2=w2349) -> (element #1=w2340:u16, element #2=w2341:u16)
              n812 = Less Or Equal?(x=w2340, y=w2341) -> (x <= y?=w2337:bool)
              n813 = Select(t=w2347, s=w2337, f=myRIO_BRig_RT__Case_Exp_stateList."initTrial" ("Enum")) -> (s? t:f=w2348:T2)
              n814 = Select(t=w2347, s=w2346, f=w2348) -> (s? t:f=w2335:T2)
            }
            frame "endBlock" {
              # "R"
              # "L"
              # "idxDataBlock"
              n815 = Equal?(x=w2378, y=enum16{"Left", "Right"}."Left") -> (x = y?=w2377:bool)
              n816 = call "myRIO_BRig_RT_dataCurrent_idxDataBlockL.vi"() -> ("output_idxDataBlock__L"=w2381:i32)  [unwired: 11 in]
              n817 = call "myRIO_BRig_RT_dataCurrent_idxDataBlockR.vi"() -> ("output_idxDataBlock__R"=w2380:i32)  [unwired: 11 in]
              n818 = Increment(x=w2372) -> (x+1=w2371:i32)
              n819 = Select(t=w2381, s=w2377, f=w2380) -> (s? t:f=w2375:i32)
              n820 = To Unsigned Word Integer(number=w2371) -> (unsigned 16bit integer=w2373:u16)
              n821 = local read "START"() -> (w2401:bool)
              n822 = local read "STOP_endBlock"() -> (w2396:bool)
              n823 = local read "STOP_endTrial"() -> (w2399:bool)
              n824 = local read "STOP_abort"() -> (w2398:bool)
              n825 = Replace Array Subset(array=w2376, new element=w2373, index=w2375) -> (w2374:u16[])
              n826 = Not(x=w2401) -> (.not. x?=w2400:bool)
              n827 = Compound Arithmetic op=OR(w2400, w2396, w2399, w2398) -> (w2397:bool)
              n828 = Select(t=myRIO_BRig_RT__Case_Exp_stateList."endExp" ("Enum"), s=w2397, f=myRIO_BRig_RT__Case_Exp_stateList."initBlock" ("Enum")) -> (s? t:f=w2405:T2)
            }
            frame "endExp" {
            }
            frame "commConnect" {
              n829 = call "myRIO_BRig_RT_comm_webdav_connect.vi"("input_password"="Host Password", "input_username"="Host UserName") -> ("output_Iconnected"=w2426:bool, "output_hSession"=w2444:T6)  [unwired: 7 in, 1 out]
              "Connected To Host?" <- w2426
              n830 = case shown="False" w2426 {
                frame False {
                  n831 = One Button Dialog(message="Connection Failed!\nData not being saved!") -> ()  [unwired: 1 in, 1 out]
                }
                frame True {
                }
              }
            }
            frame "commUpload_pre" {
              n832 = Select(t=myRIO_BRig_RT__Case_Exp_stateList."commUpload_dataBlock" ("Enum"), s=w2451, f=myRIO_BRig_RT__Case_Exp_stateList."endTrial3") -> (s? t:f=w2449:T2)
            }
            frame "commUpload_dataBlock" {
              n833 = call "myRIO_BRig_RT_comm_webdav_uploadFile__data.vi"("input_fileName_prefix"=w2472, "input_fileName"="dataBlock" ("input_filename"), "input_hSession"=w2474) -> ()  [unwired: 8 in, 1 out]
            }
            frame "commUpload_dataCurrent" {
              n834 = call "myRIO_BRig_RT_comm_webdav_uploadFile__data.vi"("input_fileName_prefix"=w2493, "input_fileName"="dataCurrent" ("input_filename"), "input_hSession"=w2495) -> ()  [unwired: 8 in, 1 out]
            }
            frame "commUpload_dataExp" {
              n835 = call "myRIO_BRig_RT_comm_webdav_uploadFile__data.vi"("input_fileName_prefix"=w2514, "input_fileName"="dataExp" ("input_filename"), "input_hSession"=w2516) -> ()  [unwired: 8 in, 1 out]
            }
            frame "commUpload_dataLC" {
              n836 = call "myRIO_BRig_RT_comm_webdav_uploadFile__data.vi"("input_fileName_prefix"=w2535, "input_fileName"="dataLC" ("input_filename"), "input_hSession"=w2537) -> ()  [unwired: 8 in, 1 out]
            }
            frame "commUpload_dataTrial" {
              n837 = call "myRIO_BRig_RT_comm_webdav_uploadFile__data.vi"("input_fileName_prefix"=w2559, "input_fileName"="dataTrial" ("input_filename"), "input_hSession"=w2561) -> ()  [unwired: 8 in, 1 out]
            }
            frame "saveData_dataBlock" {
              # "idxDataBlockR"
              # "idxDataBlockL"
              n838 = call "myRIO_BRig_RT_dataCurrent_idxDataBlockL.vi"() -> ("output_idxDataBlock__L"=w2585:i32)  [unwired: 11 in]
              n839 = call "myRIO_BRig_RT_dataCurrent_idxDataBlockR.vi"() -> ("output_idxDataBlock__R"=w2586:i32)  [unwired: 11 in]
              n840 = Index Array(array=w2587, index #1=w2585, index #2=w2586) -> (element #1=w2584:u16, element #2=w2583:u16)
              n841 = Greater?(x=w2584, y=w2583) -> (0:w2582:bool)
              n842 = Select(t=w2584, s=w2582, f=w2583) -> (s? t:f=w2580:u16)
              n843 = Increment(x=w2580) -> (x+1=w2579:u16)
              n844 = To Long Integer(number=w2579) -> (32bit integer=w2578:i32)
              n845 = Array Subset(array=w2581, length (row)=w2578) -> (w2577:u16[][])  [unwired: 3 in]
              n846 = call "myRIO_BRig_RT_comm_webdav_saveArrayToFile__2D_u16.vi"("Array"=w2577, "input_filename"="dataBlock") -> ()  [unwired: 10 in]
            }
            frame "saveData_dataCurrent" {
              n847 = call "myRIO_BRig_RT_comm_webdav_saveArrayToFile__1D_u16.vi"("Array"=w2606, "input_filename"="dataCurrent") -> ()  [unwired: 10 in]
            }
            frame "saveData_dataExp" {
              # "runTime"
              n848 = Get Date/Time In Seconds() -> (seconds since 1Jan1904=w2634:timestamp)
              n849 = To Double Precision Float(number=w2634) -> (double precision float=w2633:dbl)
              n850 = call "myRIO_BRig_RT_dataExp_runTime_seconds.vi"() -> ("output_RunTime_minutes"=w2632:i32)  [unwired: 11 in]
              n851 = Subtract(x=w2633, y=w2631) -> (x-y=w2628:dbl)
              n852 = To Unsigned Word Integer(number=w2628) -> (unsigned 16bit integer=w2627:u16)
              n853 = Replace Array Subset(array=w2626, new element=w2627, index=w2632) -> (w2629:u16[])
              n854 = call "myRIO_BRig_RT_comm_webdav_saveArrayToFile__1D_u16.vi"("Array"=w2629, "input_filename"="dataExp") -> ()  [unwired: 10 in]
            }
            frame "saveData_dataLC" {
              n855 = call "myRIO_BRig_RT_comm_webdav_saveArrayToFile__1D_u16.vi"("Array"=w2653, "input_filename"="dataLC") -> ()  [unwired: 10 in]
            }
            frame "saveData_dataTrial" {
              # "idxTrial"
              n856 = call "myRIO_BRig_RT_dataCurrent_idxDataTrial.vi"() -> ("output_idxDataTrial"=w2678:i32)  [unwired: 11 in]
              n857 = Index Array(array=w2679, index=w2678) -> (element=w2675:u16)
              n858 = Increment(x=w2675) -> (x+1=w2674:u16)
              n859 = To Long Integer(number=w2674) -> (32bit integer=w2673:i32)
              n860 = Array Subset(array=w2676, length (row)=w2673) -> (w2677:u16[][])  [unwired: 3 in]
              n861 = call "myRIO_BRig_RT_comm_webdav_saveArrayToFile__2D_u16.vi"("Array"=w2677, "input_filename"="dataTrial") -> ()  [unwired: 10 in]
            }
          }
          n862 = case shown="True" w1023 {
            tunnel: w1019 -> [w1046 w1054]
            tunnel: w1022 -> [_ w1050]
            tunnel: w1021 -> [_ w1049]
            tunnel: w1020 -> [_ w1048]
            tunnel: w989 -> [_ w1047]
            tunnel: [w1046 w1053] -> w1018
            tunnel: w1017 -> [w1045 w1052]
            tunnel: [w1045 w1051] -> w1016
            frame False {
            }
            frame True {
              n863 = call "myRIO_BRig_RT__Case_Exp__recordLick.vi"("intput_state__trialEnd"=w1047, "intput_state__trialStart"=w1048, "input_lick__R"=w1049, "input_lick__L"=w1050, "input_dataCurrent"=w1052, "input_dataLick"=w1054) -> ("output_dataCurrent"=w1051:u16[], "output_dataLick"=w1053:u16[][])  [unwired: 4 in]
            }
          }
          n864 = Or(x=w991, y=w992) -> (x .or. y?=w978:bool)
          n865 = Or(x=w995, y=w975) -> (x .or. y?=w964:bool)
          n866 = Or(x=w974, y=w996) -> (x .or. y?=w990:bool)
          n867 = Or(x=w994, y=w993) -> (x .or. y?=w979:bool)
          n868 = Or(x=w1024, y="STOP_abort") -> (x .or. y?=w1026:bool)
          n869 = Or(x=w952, y=w953) -> (x .or. y?=w950:bool)
          n870 = Or(x=w954, y=w953) -> (x .or. y?=w951:bool)
          n871 = xnode "Read/Write Control"("FPGA VI Reference In"=w966, "error in"=w965, "A1_SR"=w979, "A3_SL"=w978, "A6_Act"=w963, "audioTrigger_L"=w964, "audioAmp_L"=w1005, "audioFreq_L_Hz"=w973, "audioTrigger_R"=w990, "audioAmp_R"=w1006, "audioFreq_R_Hz"=w1007, "laserledMTrig"=w950, "laserMTrig"=w951) -> ("FPGA VI Reference Out"=w1015:refnum<k20>, "error out"=w1014:errorcluster)
          n872 = node-c288() -> ()  [unwired: 1 in, 1 out]
          "cState" <- w1020
        }
        n873 = node-c288(w910) -> ()  [unwired: 1 out]
        n874 = flat-sequence {
          tunnel: w906 -> [w942]
          tunnel: w905 -> [w941]
          tunnel: [w940] -> w898
          tunnel: [w939] -> w897
          tunnel: [w946] -> w899
          tunnel: [w947] -> w904
          tunnel: w898 -> [w947]
          tunnel: w897 -> [w946]
          frame #0 {
            w943 = u16 0 ("AudioLeft_phase_inc")
            w938 = FALSE
            n875 = xnode "Read/Write Control"("FPGA VI Reference In"=w942, "error in"=w941, "Counts_Reset"=TRUE, "audioTrigger_L"=w938, "audioFreq_L_Hz"=w943, "audioAmp_L"=w943, "audioTrigger_R"=w938, "audioFreq_R_Hz"=w943, "audioAmp_R"=w943, "A3_SL"=w938, "A1_SR"=w938, "A6_Act"=w938) -> ("FPGA VI Reference Out"=w940:refnum<k20>, "error out"=w939:errorcluster)
          }
          frame #1 {
            w945 = FALSE ("START")
            n876 = local write "START"(w945) -> ()
            n877 = local write "STOP_endTrial"(w945) -> ()
            n878 = local write "STOP_endBlock"(w945) -> ()
          }
        }
        n879 = stacked-sequence {
          tunnel: w882 -> [w918 _]
          tunnel: w880 -> [w919 _]
          tunnel: w879 -> [_ w924]
          tunnel: w878 -> [_ w923]
          tunnel: w877 -> [_ w922]
          tunnel: w876 -> [w912 _]
          frame #0 {
            n880 = call "myRIO_BRig_RT_dataCurrent_idxDataLick.vi"() -> ("output_idxDataLick"=w913:i32)  [unwired: 11 in]
            n881 = Index Array(array=w912, index=w913) -> (element=w915:u16)
            n882 = Increment(x=w915) -> (x+1=w916:u16)
            n883 = call "myRIO_BRig_RT_comm_webdav_saveArrayToFile__1D_u16.vi"("Array"=w919, "input_filename"="dataMTrig") -> ()  [unwired: 10 in]
            n884 = To Long Integer(number=w916) -> (32bit integer=w914:i32)
            n885 = Array Subset(array=w918, length (row)=w914) -> (w917:u16[][])  [unwired: 3 in]
            n886 = call "myRIO_BRig_RT_comm_webdav_saveArrayToFile__2D_u16.vi"("Array"=w917, "input_filename"="dataLick") -> ()  [unwired: 10 in]
          }
          frame #1 {
            n887 = case shown="True" w924 {
              tunnel: w923 -> [_ w926]
              tunnel: w922 -> [_ w925]
              frame False {
              }
              frame True {
                n888 = stacked-sequence {
                  tunnel: w926 -> [w928 w935 w937]
                  tunnel: w925 -> [w929 w934 _]
                  frame #0 {
                    n889 = call "myRIO_BRig_RT_comm_webdav_uploadFile__announce.vi"("input_addText"=TRUE, "input_fileName_prefix"=w929, "intput_fileName"="curExp_end", "intput_hSession"=w928) -> ("output_Isuccess"=w927:bool)  [unwired: 6 in, 1 out]
                    n890 = case shown="True" w927 {
                      frame False {
                        n891 = One Button Dialog(message="!!! Warning !!! Your data is located at C:\\BehaviorRig\\commTransfer") -> ()  [unwired: 1 in, 1 out]
                      }
                      frame True {
                        n892 = Wait (ms)(milliseconds to wait=u32 20) -> ()  [unwired: 1 out]
                      }
                    }
                  }
                  frame #1 {
                    n893 = call "myRIO_BRig_RT__endExp_sendData.vi"("input_fileName_prefix"=w934, "input_hSession"=w935) -> ()  [unwired: 8 in, 2 out]
                  }
                  frame #2 {
                    n894 = local write "Connected To Host?"(FALSE ("Connected To Host?")) -> ()
                    n895 = call <vilib>:"Close Session.vi"("session handle"=w937) -> ()  [unwired: 14 in, 1 out]
                  }
                }
              }
            }
          }
        }
      }
    }
    n896 = local read "STOP_abort"() -> (w30:bool)
  }
  n897 = xnode "Read/Write Control"("FPGA VI Reference In"=w8, "error in"=w7, "FPGA_Stop"=TRUE) -> ("FPGA VI Reference Out"=w13:refnum<k20>, "error out"=w14:errorcluster)
  n898 = xnode "Close FPGA VI Reference"("FPGA VI Reference In"=w13, "error in"=w14) -> ("error out"=w12:errorcluster)
  n899 = call <vilib>:"Reset myRIO.vi"("error in (no error)"=w12) -> ()  [unwired: 10 in, 1 out]
